vi "WVDIAL_3A_Data_v2.vi"() -> ()   [LabVIEW 2012]
uses:
  C:/H2O_DIAL/LabVIEW-2012/Newport_LabVIEW_v3-0-2/LabVIEW 2009/PowerMeterCommands.dll
  H2O_DIAL/LabVIEW-2012/Newport_LabVIEW_v3-0-2/LabVIEW 2009/PowerMeterCommands.dll
  <vilib>/DAQmx/write.llb/DAQmx Write (Digital 1D Bool NChan 1Samp 1Line).vi
  <vilib>/DAQmx/miscellaneous.llb/DAQmx Fill In Error Info.vi
  <vilib>/Analysis/baseanly.llb/Mean (DBL).vi
  H2O_DIAL/LabVIEW-2012/Scalar_Data.vi
  H2O_DIAL/LabVIEW-2012/Bristol WM V2_31b/CLDevIFace.dll
  <vilib>/Analysis/NI_AALBase.lvlib
panel:
  out "FileHour":i32=1
  out "L_Count":i32=91
  out "sigma_off_total":dbl[](array[numeric])=[5.2234200558950385e-25, 5.188441808210764e-25, 5.153565757684458e-25, 5.118792258898494e-25, 5.08412169128079e-25, 5.049554458516742e-25, 5.015090988058244e-25, 4.980731730520144e-25, 4.9464771591183625e-25, 4.912327769020908e-25, 4.878284076745431e-25, 4.844346619505553e-25, 4.810515954528075e-25, 4.776792658367297e-25, 4.743177326209202e-25, 4.709670571178148e-25, 4.676273023536675e-25, 4.642985329979768e-25, 4.60980815288796e-25, 4.576742169547043e-25, 4.543788071301696e-25, 4.510946562860497e-25, 4.478218361454665e-25, 4.445604195984992e-25, 4.413104806264462e-25, 4.380720942207995e-25, 4.348453362900999e-25, 4.316302835906913e-25, 4.284270136293901e-25, 4.252356045994737e-25, 4.220561352713886e-25, 4.188886849357295e-25, 4.157333332959233e-25, 4.125901604102425e-25, 4.0945924658480525e-25, 4.0634067231055894e-25, 4.0323451816809216e-25, 4.0014086475994155e-25, 3.970597926185606e-25, 3.9399138213596143e-25, 3.9093571347801357e-25, 3.878928665154662e-25, 3.848629207415147e-25, 3.8184595520156785e-25, 3.7884204841767665e-25, 3.7585127831272873e-25, 3.728737221470386e-25, 3.699094564429195e-25, 3.6695855692870667e-25, 3.6402109845120747e-25, 3.610971549313007e-25, 3.581867992981925e-25, 3.552901034160713e-25, 3.524071380427552e-25, 3.49537972759939e-25, 3.466826759230286e-25, 3.4384131460904257e-25, 3.4101395456540365e-25, 3.38200660154994e-25, 3.3540149432465886e-25, 3.326165185385074e-25, 3.298457927536896e-25, 3.270893753698064e-25, 3.2434732319867498e-25, 3.216196914181406e-25, 3.1890653354567716e-25, 3.1620790140097576e-25, 3.135238450817045e-25, 3.1085441293269563e-25, 3.081996515166733e-25, 3.0555960559996366e-25, 3.0293431812397327e-25, 3.0032383018574547e-25, 2.9772818102740086e-25, 2.951474080128153e-25, 2.925815466205591e-25, 2.9003063042754744e-25, 2.874946911049838e-25, 2.84973758409989e-25, 2.824678601768354e-25, 2.7997702231895546e-25, 2.775012688207971e-25, 2.7504062174242674e-25, 2.725951012245797e-25, 2.7016472548149107e-25, 2.677495108166955e-25, 2.6534947162834797e-25, 2.629646204115954e-25, 2.6059496777421353e-25, 2.5824052244655604e-25, 2.5590129129175218e-25, 2.535772793262254e-25, 2.5126848972851255e-25, 2.4897492386178596e-25, 2.4669658128642407e-25, 2.4443345978445496e-25, 2.4218555537559024e-25, 2.399528623422043e-25, 2.37735373247562e-25, 2.355330789669388e-25, 2.3334596869947745e-25, 2.311740300089403e-25, 2.2901724883551664e-25, 2.268756095284891e-25, 2.247490948773977e-25, 2.2263768613169987e-25, 2.205413630361226e-25, 2.184601038574965e-25, 2.163938854116898e-25, 2.1434268310139646e-25, 2.1230647093544735e-25, 2.1028522156937155e-25, 2.0827890633082375e-25, 2.0628749525435776e-25, 2.0431095710820085e-25, 2.0234925943095863e-25, 2.0040236856159133e-25, 1.9847024966907277e-25, 1.9655286678713153e-25, 1.946501828442999e-25, 1.9276215969536646e-25, 1.908887581541266e-25, 1.8902993802421601e-25, 1.8718565813176687e-25, 1.8535587635175008e-25, 1.8354054964632128e-25, 1.8173963408589502e-25, 1.7995308488869285e-25, 1.7818085644394773e-25, 1.7642290234549009e-25, 1.7467917541391984e-25, 1.729496277358023e-25, 1.7123421068169184e-25, 1.6953287493942957e-25, 1.6784557053870135e-25, 1.6617224687716046e-25, 1.645128527500769e-25, 1.6286733636906083e-25, 1.6123564539396905e-25, 1.5961772694937406e-25, 1.5801352765602062e-25, 1.5642299364526662e-25, 1.548460705871435e-25, 1.5328270370926741e-25, 1.51732837817522e-25, 1.5019641731424406e-25, 1.4867338622066092e-25, 1.4716368819285135e-25, 1.4566726653864935e-25, 1.44184064237116e-25, 1.42714023950682e-25, 1.412570880435065e-25, 1.3981319859339977e-25, 1.383822974081728e-25, 1.3696432603470826e-25, 1.3555922577345145e-25, 1.341669376883176e-25, 1.3278740261649085e-25, 1.3142056117906531e-25, 1.3006635378746162e-25, 1.2872472065372546e-25, 1.2739560179342136e-25, 1.2607893703627722e-25, 1.2477466602699388e-25, 1.234827282310524e-25, 1.222030629393837e-25, 1.2093560926749042e-25, 1.1968030615982307e-25, 1.1843709238949383e-25, 1.1720590655757887e-25, 1.1598668709159086e-25, 1.1477937224574596e-25, 1.1358390009609953e-25, 1.1240020853546206e-25, 1.1122823527270164e-25, 1.100679178237489e-25, 1.0891919350583027e-25, 1.077819994310042e-25, 1.0665627249682734e-25, 1.055419493776449e-25, 1.0443896651464614e-25, 1.0334726010358994e-25, 1.0226676608409127e-25, 1.0119742012573873e-25, 1.0013915761470858e-25, 9.909191363844297e-26, 9.805562297021883e-26, 9.703022005144416e-26, 9.60156389756751e-26, 9.501181346712233e-26, 9.401867686339235e-26, 9.303616209277055e-26, 9.206420165441348e-26, 9.110272759315423e-26, 9.015167147734415e-26, 8.921096437321057e-26, 8.828053681989907e-26, 8.73603188005984e-26, 8.645023971702555e-26, 8.555022835840961e-26, 8.466021287248513e-26, 8.378012073408909e-26, 8.290987871284668e-26, 8.204941284051091e-26, 8.119864837645385e-26, 8.035750977236182e-26, 7.952592063685049e-26, 7.870380369750861e-26, 7.78910807636565e-26, 7.708767268635035e-26, 7.629349932029705e-26, 7.550847948159768e-26, 7.47325309074078e-26, 7.396557021337458e-26, 7.320751285077931e-26, 7.245827306419816e-26, 7.171776384642328e-26, 7.098589689477262e-26, 7.026258256696376e-26, 6.954772983531929e-26, 6.884124624288349e-26, 6.814303785802483e-26, 6.745300923016202e-26, 6.677106334525768e-26, 6.609710158212605e-26, 6.543102366959471e-26, 6.477272764391407e-26, 6.412210980842389e-26, 6.34790646930539e-26, 6.284348501716449e-26, 6.221526165291305e-26, 6.159428359128027e-26, 6.098043791110177e-26, 6.037360974977726e-26, 5.977368227808834e-26, 5.918053667850245e-26, 5.859405212623739e-26, 5.801410577641224e-26, 5.744057275480635e-26, 5.687332615316891e-26, 5.631223703211629e-26, 5.575717442793144e-26, 5.520800536756566e-26, 5.466459488975701e-26, 5.412680607402506e-26, 5.35945000776066e-26, 5.306753618135332e-26, 5.254577184417943e-26, 5.202906276764818e-26, 5.1517262970050066e-26, 5.1010224871886087e-26, 5.050779939197868e-26, 5.000983605519522e-26, 4.9516183112447033e-26, 4.9026687672528495e-26, 4.854119584799368e-26, 4.8059552912484194e-26, 4.7581603473050947e-26, 4.710719165491264e-26, 4.663616130109859e-26, 4.616835618489491e-26, 4.570362023679514e-26, 4.524179778545254e-26, 4.478273381142984e-26, 4.432627421488372e-26, 4.3872266096240307e-26, 4.3420558048809627e-26, 4.297100046345158e-26, 4.252344584422084e-26, 4.2077749134265266e-26, 4.163376805034476e-26, 4.119136342586736e-26, 4.075039955995771e-26, 4.0310744572065636e-26, 3.987227076009789e-26, 3.943485496023477e-26, 3.8998378906971834e-26]
  out "sigma_on_total":dbl[](array[numeric])=[4.9081568957923354e-23, 4.92540132407037e-23, 4.9424189538428444e-23, 4.959204027078022e-23, 4.9757507806516237e-23, 4.992053449322544e-23, 5.008106268873085e-23, 5.0239034790046195e-23, 5.0394393268030595e-23, 5.054708069641985e-23, 5.0697039787676814e-23, 5.084421342075185e-23, 5.0988544683523154e-23, 5.1129976895868996e-23, 5.126845365311698e-23, 5.140391885773363e-23, 5.153631675468891e-23, 5.166559196475097e-23, 5.1791689527760933e-23, 5.1914554929330853e-23, 5.203413414598583e-23, 5.215037367456545e-23, 5.226322057682808e-23, 5.237262250900696e-23, 5.2478527766919827e-23, 5.2580885314179625e-23, 5.2679644828952156e-23, 5.277475673477536e-23, 5.2866172240694114e-23, 5.295384338012182e-23, 5.303772304537347e-23, 5.311776502184215e-23, 5.319392403512445e-23, 5.326615577767154e-23, 5.333441694809072e-23, 5.339866529189547e-23, 5.345885962979486e-23, 5.351495989921125e-23, 5.356692718784368e-23, 5.361472376181958e-23, 5.365831311243196e-23, 5.36976599768476e-23, 5.373273037898196e-23, 5.376349165681213e-23, 5.37899124988806e-23, 5.381196297008713e-23, 5.382961454332835e-23, 5.38428401304352e-23, 5.385161411059042e-23, 5.385591235070043e-23, 5.385571224246857e-23, 5.385099272271794e-23, 5.38417342942276e-23, 5.382791905459925e-23, 5.380953072059697e-23, 5.378655464011758e-23, 5.375897781966347e-23, 5.37267889433291e-23, 5.36899783827954e-23, 5.364853822719629e-23, 5.360246228475637e-23, 5.355174610231828e-23, 5.349638697779521e-23, 5.34363839732697e-23, 5.337173791660417e-23, 5.3302451421763e-23, 5.322852888345e-23, 5.314997649053672e-23, 5.306680222579485e-23, 5.29790158702747e-23, 5.28866290020075e-23, 5.278965499950113e-23, 5.268810903096198e-23, 5.2582008061107946e-23, 5.247137083724484e-23, 5.2356217884409377e-23, 5.2236571501233056e-23, 5.211245574333022e-23, 5.198389641603278e-23, 5.185092105901141e-23, 5.17135589337794e-23, 5.1571841000701964e-23, 5.142579991244177e-23, 5.127546998799546e-23, 5.112088718505753e-23, 5.096208909373192e-23, 5.0799114899221017e-23, 5.063200536129518e-23, 5.0460802792496746e-23, 5.028555101876762e-23, 5.0106295364265944e-23, 4.992308260936456e-23, 4.973596096602486e-23, 4.954498004029935e-23, 4.935019080307414e-23, 4.915164555028606e-23, 4.894939786914789e-23, 4.8743502601017755e-23, 4.8534015803309426e-23, 4.8320994710498925e-23, 4.8104497689477555e-23, 4.7884584208487056e-23, 4.766131478615105e-23, 4.7434750956610527e-23, 4.7204955219616444e-23, 4.69719910069179e-23, 4.6735922624026386e-23, 4.649681522533156e-23, 4.6254734750186114e-23, 4.600974789249439e-23, 4.57619220410126e-23, 4.5511325250906414e-23, 4.525802618610929e-23, 4.500209407611472e-23, 4.474359867273473e-23, 4.448261020445578e-23, 4.421919932603377e-23, 4.395343707548312e-23, 4.368539483365195e-23, 4.341514426954153e-23, 4.314275730762695e-23, 4.286830607379014e-23, 4.2591862848902865e-23, 4.2313500037219867e-23, 4.2033290113601744e-23, 4.1751305583264584e-23, 4.146761894203741e-23, 4.11823026276728e-23, 4.089542898843256e-23, 4.060707023565222e-23, 4.031729840885392e-23, 4.0026185329749454e-23, 3.9733802571128887e-23, 3.9440221417049496e-23, 3.914551282848814e-23, 3.8849747398167707e-23, 3.8552995327156094e-23, 3.8255326381372917e-23, 3.7956809869749994e-23, 3.7657514597924226e-23, 3.735750884129758e-23, 3.705686031888425e-23, 3.6755636163448055e-23, 3.64539028858424e-23, 3.6151726349373734e-23, 3.584917174725625e-23, 3.554630356985923e-23, 3.5243185586260696e-23, 3.4939880817830895e-23, 3.463645150634312e-23, 3.433295910921002e-23, 3.402946426295741e-23, 3.372602676523462e-23, 3.34227055661974e-23, 3.311955873523278e-23, 3.2816643454298113e-23, 3.25140159993815e-23, 3.221173171682913e-23, 3.1909845025572505e-23, 3.1608409383034083e-23, 3.1307477295284364e-23, 3.1007100281088115e-23, 3.070732888376049e-23, 3.04082126474433e-23, 3.0109800110649004e-23, 2.981213880845769e-23, 2.9515275248158936e-23, 2.921925492114598e-23, 2.8924122286396243e-23, 2.862992077239196e-23, 2.833669276844683e-23, 2.8044479630192115e-23, 2.7753321674532616e-23, 2.746325817565861e-23, 2.7174327372944447e-23, 2.688656646317821e-23, 2.6600011615395604e-23, 2.6314697957689884e-23, 2.6030659595305698e-23, 2.5747929606268752e-23, 2.5466540053635235e-23, 2.5186521982816548e-23, 2.4907905435188057e-23, 2.463071945366495e-23, 2.4354992087370023e-23, 2.4080750405260247e-23, 2.380802050198059e-23, 2.353682750766613e-23, 2.326719560301616e-23, 2.299914802049696e-23, 2.2732707065177826e-23, 2.2467894118572504e-23, 2.2204729660047475e-23, 2.1943233268536394e-23, 2.1683423643079143e-23, 2.1425318612924744e-23, 2.116893515101761e-23, 2.0914289389174596e-23, 2.0661396630556457e-23, 2.0410271362434758e-23, 2.016092727615468e-23, 1.991337727178575e-23, 1.9667633486579524e-23, 1.9423707291781575e-23, 1.9181609326455474e-23, 1.8941349497350253e-23, 1.8702937000488233e-23, 1.8466380333351368e-23, 1.8231687314796873e-23, 1.799886509336085e-23, 1.7767920163348423e-23, 1.753885838197544e-23, 1.7311684983845758e-23, 1.7086404592966803e-23, 1.686302123717775e-23, 1.6641538364768544e-23, 1.6421958857376648e-23, 1.620428504171699e-23, 1.598851870911703e-23, 1.5774661121324435e-23, 1.556271303190841e-23, 1.5352674693034418e-23, 1.5144545875226826e-23, 1.4938325872962545e-23, 1.473401352401079e-23, 1.4531607219009912e-23, 1.4331104915117057e-23, 1.4132504146459468e-23, 1.3935802040397153e-23, 1.374099532469008e-23, 1.3548080345265754e-23, 1.3357053070330198e-23, 1.3167909108681765e-23, 1.2980643720076896e-23, 1.2795251821945616e-23, 1.2611728005968538e-23, 1.2430066544509207e-23, 1.2250261405770924e-23, 1.2072306260846092e-23, 1.1896194495023627e-23, 1.1721919218843238e-23, 1.1549473277291007e-23, 1.1378849259678912e-23, 1.121003950934157e-23, 1.1043036133917084e-23, 1.0877831013862512e-23, 1.0714415811598837e-23, 1.0552781980469257e-23, 1.0392920773510609e-23, 1.023482325203656e-23, 1.0078480294731518e-23, 9.923882603736919e-24, 9.771020716164171e-24, 9.619885008426139e-24, 9.470465705295025e-24, 9.322752887996336e-24, 9.176736499509695e-24, 9.032406354244015e-24, 8.889752142972557e-24, 8.748763440184707e-24, 8.609429710000158e-24, 8.471740313713177e-24, 8.335684515307783e-24, 8.201251486848566e-24, 8.068430314303916e-24, 7.937210004283393e-24, 7.807579488329678e-24, 7.67952762979291e-24, 7.553043225158898e-24, 7.428115013769768e-24, 7.304731678841886e-24, 7.182881854618292e-24, 7.062554128232828e-24, 6.943737045965018e-24, 6.826419116313546e-24, 6.710588814858551e-24, 6.596234585700559e-24]
  out "background start":u32=269
  in  "Tab Control 2":enum32{"WV ND far", "WV ND near"}(tab)
  out "Water Vapor Number Density":dbl[][](graph)=[[-1.0252849343578538, 0.01224336928867699, 0.15835340670906267, 0.08290480575754477, 0.07669745638764922, 0.2620759623415424, 0.40352824259012626, 0.3765601485315456, 0.36227285880487015, 0.4059580103922654, 0.4019673046611201, 0.33405985865603577, 0.3170502464024163, 0.326931496733142, 0.3429736770934233, 0.3444364774253561, 0.2845356515320602, 0.21313783544633252, 0.23326342211099127, 0.28103729065715927, 0.21313141961111057, 0.18344699568861908, 0.1985633443430128, 0.15664306550500462, 0.14542928691246532, 0.1603391816642332, 0.16807578278873733, 0.15615183024203905, 0.07890698232192461, 0.05400641926340679, 0.10685143060938126, 0.08945067942871926, 0.0581898104690232, 0.029308456616610103, 0.03630780670213719, 0.10681104177716703, 0.100411545675493, 0.06706138343354981, 0.05685684243729449, 0.05193125527448508, 0.11348707030004936, 0.1035008699196596, 0.10995022367210285, 0.11937133833259062, 0.12610932475837994, 0.14237040514772434, 0.13877337413129362, 0.1368529199507475, 0.12016466926308586, 0.0995255538846496, 0.11327076262624056, 0.1147160375476178, 0.10327876531608772, 0.11333749442300015, 0.12152503880277782, 0.0905009235216747, 0.07461770257070978, 0.08412413953978554, 0.10800968932015705, 0.11174027116353434, 0.10857447444700312, 0.1321594882555679, 0.14442251058556227, 0.12312399237245467, 0.08690887689465081, 0.08885386048416666, 0.09841400838528362, 0.08885871503781699, 0.09065384006052782, 0.07631420811267337, 0.028801438306251165, 0.017317933019278177, 0.00535924647765615, -0.009366925462381862, 0.02537030105111806, 0.04553727504960618, 0.04087573332295979, 0.009566848406822514, -0.03765211983627373, -0.030845499715426574, 0.0094243698383032, -0.01191307862878305, -0.007766189150850719, 0.02512004862547047, -0.009588975820370573, -0.021862900628392096, -0.02332999129653946, -0.008298987729287529, 0.03829137791338236, 0.06788185167298495, 0.04415872088882591, 0.04626176957978276, 0.05722361632703139, -0.022937610835842275, -0.004658082206540099, 0.03497441915011394, 0.014559704329153577, 0.018331797591107316, 0.0002765651829681014, -0.01750292048905302, -0.01389136569261041, -0.0148966495460508, 0.03341365244368827, 0.07959799083893267, 0.001172873742239602, -0.04989443850404001, 0.019178610287384813, 0.022978059399375285, -0.021897118324035424, 0.014353504774367415, 0.05207825830382806, 0.02543732315528786, -0.08859996249031706, -0.07930855892996377, 0.02199957803258167, -0.005751854282845175, -0.06734218818626583, -0.06101837900811169, 0.00811186048587734, -0.030347870972451, -0.018601423955109716, 0.025343088130804294, -0.000654365715296774, -0.021410549313652594, -0.00711404508875446, 0.015640507400628483, 0.01980450921423653, -0.020816862317439747, -0.13136076782915793, -0.04953574617480027, -0.015688088030325335, 0.012270851704896515, 0.07078369570658659, -0.010036414876574785, -0.07560094992065346, 0.029113962431097925, 0.022316828296317252, 0.01590620564861339, 0.115062446638934, -0.02408844575634284, -0.17020265488657252, -0.1451398382852584, -0.02445566701513559, -0.03235393341027663, 0.02164604133106217, 0.03204665984442202, -0.027642125840527564, 0.0006023003531748955, 0.0003496841625749631, 0.020854103047599864, 0.10842911005120683, -0.03471048223400414, -0.24585708970897793, -0.05744168418466623, 0.10508588586604846, -0.0012595297900689863, -0.1422957818224093, -0.1528480963241691, -0.024891406845158556, 0.18064750429676343, 0.18870158459369052, 0.08124391772376854, 0.1925945351989546, 0.18885896239951047, -0.028423489511011396, 0.08782982844147444, 0.4018531072514305, 0.28295974281274405, 0.141752362604584, -0.04596416681267469, -0.19599669013524573, -0.1832886215602881, -0.221330016936266, -0.20746810479592004, -0.2533548550992385, -0.2640461399425933, -0.5552226085781474, -0.25658834207217607, 0.07631635532473394, 0.24357172305557667, 0.24357507864442013, 0.0054930164331440596, -0.26352244101342837, -0.21458731889229515, 0.4671152360442577, 0.35493908142470326, 0.540206234420223, 0.6253545626789414, -0.1918135463763898, -0.857997351327124, -0.6115474584870345, 0.12686579467009856, 1.1193396529920683, 0.9491303824250846, -0.24898239698578367, -0.2173961551411876, -0.4716937237467244, -0.9264813435003413, -0.0023983309321438844, 0.13861484422091855, 0.18306415863530784, 0.05031596208368666, -0.9039913856241271, -0.8292733524419981, -0.5087347525929017, -0.6153644321851048, -0.14914507407421404, -0.42810566981401466, -1.247232243863552, 0.05482762929954191, 0.6860297651363804, 0.9481996959641221, 0.5629045863681271, -0.04576191379675542, -0.08731851988840891, 0.15154855903866532, 0.9587585142774312, 2.6746560753275936, 2.531440286016611, 1.3601958991015755, 1.2395200095649133, -0.6781596022648028, -1.1160153572546019, 0.5812137856885836, 3.4687378449956365, 1.4464917210606263, -0.9295342166169639, -1.1204191549870324, 0.1034792544561276, -0.3306455660619927, -1.6655638739808207, -0.17082350185743553, 1.078813649527156, 1.0096264846682745, 5.118342980436561, -0.5598249934362547, -3.0525737805264908, -2.493481796852318, -0.6766514276077036, -1.9364332962989481, -0.9603886125585042, 9.722825473022084, 12.019451658920579, 1.5485181169999382, -10.639197997428594, 1.410760631694313, 1.6311961050885482, -0.7606371982561374, 8.050945482359824, 12.222718623912504, 2.8379417404869214, -8.467893225176228, -7.892104308000269, 7.561105736814597, 1.8338678599324048, -24.44144266759318, -5.501789806042863, inf, nan, nan, nan, nan, nan, nan, nan, nan, nan, -inf, -28.22132689188821, -35.53185818775793, -6.267550590333384, -0.5649805048183769, 4.752482348133581, -307.43485402739964, 20.288829520425445, 9.757029206652764, 0.0, 0.0, 0.0, 0.0]]
  out "Water Vapor Number Density 2":dbl[][](graph)=[[-0.2865898034035239, 0.005398347357826392, 0.270180194427171, 0.49934908193536914, 0.4610856820815434, 0.47919125201054663, 0.41713553122041214, 0.2839520922325461, 0.2139053579349078, 0.19008321561295816, 0.16210313849803437, 0.19767316841001897, 0.24678082445960892, 0.22934149302256987, 0.23106320058472932, 0.24935743336579463, 0.228712861153675, 0.19177244383258807, 0.13822796107116675, 0.12952096392054793, 0.184961155888618, 0.15625046859598593, 0.08149130905587414, 0.08347671564892852, 0.09292450724175014, 0.09897778476272892, 0.11869505217402627, 0.1020949650068219, 0.0680375451406521, 0.05526436285002661, 0.07701578642588422, 0.08986190584998056, 0.04739696394569468, 0.05155875974538851, 0.1075732163983899, 0.05848975405725049, 0.06027341501459341, 0.15577956438219154, 0.15426807453320523, 0.119550419057958, 0.09023852284476494, 0.10731660449440052, 0.10201202655632406, 0.09015213641438144, 0.10411287521775274, 0.10329612538676994, 0.09329592009020822, 0.094255010754596, 0.11657739187690068, 0.1226902118059504, 0.09973483618224008, 0.10146470794396166, 0.11296540573869736, 0.1015626599598415, 0.0670589224001955, 0.05571375145680353, 0.11089663210326146, 0.11357746332799534, 0.06533120875001214, 0.06501193077064142, 0.07135694632306648, 0.08396571641123735, 0.10053779135695375, 0.10873851949177482, 0.1112833067067629, 0.1253430050297553, 0.0751893159577234, 0.03758941994591285, 0.07455579053102862, 0.0833519595042809, 0.08073822675968761, 0.07046574397017079, 0.01628475622108129, -0.00979323785755199, -0.0064363595850521265, -0.05424049805498369, -0.04770145348367631, -0.0651157050563226, -0.05842221368779357, -0.010132741906781893, -0.04719311826522132, -0.08061528212640966, -0.05584093426722229, -0.03736190901125273, -0.026288927003514956, -0.02735758962233305, -0.016680414061933085, 0.08698302754384295, 0.03703409407182322, -0.07428276239552731, -0.08287843499135167, -0.07246514962772428, -0.037888971379870164, 0.05050165939688743, 0.04070516703725998, 0.0013689744815177922, -0.004086178413386218, -0.0567087326925041, -0.02261065358974721, 0.013323062997568018, 0.009012099767637038, 0.06812410181727888, 0.0873623313874923, -0.04033859274693685, -0.04056170573479139, 0.018164119949206622, 0.01698920493116969, 0.03200462135731041, 0.05597485931968883, 0.004660639245897041, -0.03363415325850763, -0.044356505658716565, -0.1326763990388899, -0.1163166059591595, -0.10490018463375138, -0.05536956764781129, -0.04811219794033331, -0.14629275993812393, -0.2638330330801213, -0.11815301138792501, -0.05480137234021616, -0.09557382991076353, 0.05065173829933405, -0.021513840363060137, -0.06814917790551435, 0.04024699076309072, 0.0523783228597919, 0.024958814896366536, 0.2367237292842569, 0.15812901488128575, 0.1896038115178739, 0.17481292374171756, 0.0304620500948119, 0.17383097270155906, -0.0259345430012192, -0.08930431039819542, -0.03743898194871775, -0.11917226232517714, -0.33721378185498047, -0.457167967758754, -0.3235026283764478, -0.10013715416333623, -0.02199546241885382, -0.14544493363592895, -0.0012521147959781197, -0.12646742039302086, -0.09850072568755051, 0.0784720451940167, 0.023479703348949714, 0.1557391494055616, 0.0758192113998383, -0.07227019057095403, -0.1648907418364726, -0.2554862575973906, -0.19723726926026697, -0.23979967592154308, -0.3956428807050192, -0.15151433375207188, 0.05856942593990406, 0.023473089930657325, -0.14087719685328506, -0.4039827327250235, -0.5481665412712616, -0.038628654542470754, 0.06243643308227342, -0.11889452169279512, 0.16177519315495192, -0.12021089755834058, -0.3297469880649382, -0.518217006463964, -0.6546943085223443, -0.40952325606659373, 0.011280533075510508, 0.03250743328819382, -0.10886758905219632, -0.021942577298229692, -0.4883511099304952, -0.44815383519345425, -0.03907380619628987, 0.023132386308057345, 0.8029360270671851, 1.1829320153858496, 0.40773978168304786, -0.38586510407162455, -0.17087296696587043, 0.24229231771964327, 0.7259049980139611, 1.087664173140548, 0.33172479606023236, 0.17410391403140907, -0.4906222320735112, -0.8636149031554697, -0.714888070381581, -0.5064304478291466, -0.15804241196057325, -0.708135007951393, -1.0726075380347868, -1.5391461936251392, -0.22970891454111933, 0.36396836324290655, -0.04868841888359483, 0.05730398934642209, 0.29784952872844606, 0.6519924801558464, 0.4451080921193637, 0.12546276730951203, 0.2049887743797555, 0.5372091833320591, -0.9537044878290641, -1.2245695847958014, -0.41139863470143095, -1.7400865412460473, -1.1839668465437496, 0.13325930619296222, 0.43022454257193565, 1.251772185641275, 0.3265410906776107, -0.2873287006786283, -0.6181403368800276, 0.2720806718243457, 0.8886029089360986, 1.1163369370933798, -0.47349237339872063, -2.3967729698196005, -2.207549933190577, -1.4281793307099488, -2.552445952127832, -3.068147980767434, 1.6399347380926848, 1.9114132952232707, 2.6314283459178442, 3.2209701873261984, 4.083938620485938, 1.6750231442344234, 0.7521082601842183, 0.6308908979632994, -1.7929692303061833, 0.4854925493859792, -1.848037270233985, -1.9599707690472083, 0.22935120759831343, -3.8719930860396916, -5.299588916827538, -1.5732432106802883, -2.5938334904711406, -4.391792042628007, 4.266433069695473, 13.43473735963336, 5.908032793145804, 1.2717711422320495, -3.429469533815916, -1.1590160228244126, -0.6038000728103482, -12.455047324042539, -5.212730955931867, -6.095310308846368, -9.413121255666667, -16.629619714029694, -4.639137025788683, -7.453414942524888, -8.645137330486625, -6.187073306219781, -3.0975960529606095, 31.089273555509546, 10.980893562167019, 19.41155124836945, 9.628163529298224, 13.46382743910762, -10.97019753650602, -9.201787138642892, -10.247187579852502, -10.523303442697749, -12.419610661601844, -35.596073167566956, -21.555444628010434, -28.144694005095776, 0.0, 0.0, 0.0, 0.0]] caption="Water Vapor Number Density"
  out "RingBuffer offline near":dbl[][](array[numeric])
  out "RingBuffer aerosol near":dbl[][](array[numeric])=[[17571.5, 17868.5, 12324.5, 82.5, 83.5, 164.5, 248.5, 292.5, 320.5, 359.5, 383.5, 402.5, 395.5, 359.5, 311.5, 314.5, 336.5, 344.5, 270.5, 256.5, 274.5, 222.5, 209.5, 199.5, 193.5, 161.5, 148.5, 149.5, 165.5, 133.5, 119.5, 104.5, 109.5, 100.5, 83.5, 89.5, 69.5, 67.5, 57.5, 61.5, 58.5, 72.5, 54.5, 63.5, 66.5, 59.5, 46.5, 39.5, 47.5, 38.5, 34.5, 33.5, 44.5, 28.5, 34.5, 23.5, 21.5, 26.5, 37.5, 16.5, 22.5, 15.5, 18.5, 14.5, 18.5, 16.5, 22.5, 10.5, 21.5, 17.5, 19.5, 21.5, 12.5, 14.5, 17.5, 18.5, 20.5, 16.5, 11.5, 12.5, 12.5, 16.5, 6.5, 9.5, 0.5, 14.5, 7.5, 8.5, 5.5, 7.5, 8.5, 8.5, 5.5, 8.5, 5.5, 5.5, 6.5, 8.5, 4.5, 2.5, 6.5, 3.5, 5.5, 2.5, 7.5, 10.5, 7.5, 3.5, 8.5, 3.5, 10.5, 10.5, 5.5, 3.5, 2.5, 5.5, 4.5, 9.5, 6.5, 3.5, 4.5, -0.5, 4.5, 1.5, 2.5, 3.5, 1.5, 6.5, -0.5, -0.5, -1.5, -0.5, 5.5, 5.5, 2.5, 0.5, -0.5, 2.5, -0.5, 0.5, -0.5, 0.5, 5.5, 0.5, 1.5, -0.5, 3.5, 1.5, 3.5, 3.5, 3.5, -1.5, 0.5, 1.5, 0.5, 0.5, 0.5, 0.5, -0.5, -0.5, 4.5, -0.5, 1.5, -1.5, 2.5, -0.5, -0.5, 4.5, -0.5, 0.5, 1.5, -0.5, -0.5, 4.5, 0.5, -0.5, -0.5, 0.5, -0.5, 1.5, -0.5, 0.5, -0.5, 0.5, -0.5, -0.5, -0.5, -1.5, -0.5, 1.5, 1.5, -1.5, -1.5, 0.5, 0.5, -1.5, 0.5, -1.5, 0.5, -0.5, 3.5, 1.5, 1.5, -1.5, -0.5, -0.5, 1.5, -0.5, -0.5, -0.5, -1.5, 0.5, -1.5, 0.5, 3.5, -0.5, -0.5, -0.5, 0.5, 0.5, -1.5, -0.5, -1.5, 0.5, -1.5, 1.5, 0.5, 0.5, -0.5, 3.5, -0.5, 1.5, 0.5, -1.5, -0.5, 0.5, -0.5, -0.5, -1.5, -0.5, -1.5, -0.5, 0.5, -1.5, -1.5, -1.5, 0.5, -0.5, -1.5, -1.5, 0.5, 0.5, -1.5, -0.5, 0.5, 0.5, 0.5, 0.5, -0.5, 0.5, -1.5, -1.5, -1.5, 0.5, -0.5, -0.5, 1.5, -1.5, 0.5, -1.5, -0.5, -0.5, -0.5, 0.5, -0.5, 0.5, 1.5, 0.5, 0.5], [18920.5, 19235.5, 12427.5, 85.5, 107.5, 173.5, 275.5, 258.5, 313.5, 342.5, 323.5, 399.5, 353.5, 364.5, 366.5, 322.5, 323.5, 295.5, 273.5, 289.5, 284.5, 247.5, 210.5, 195.5, 218.5, 157.5, 162.5, 151.5, 134.5, 117.5, 113.5, 101.5, 110.5, 98.5, 88.5, 87.5, 78.5, 75.5, 60.5, 47.5, 60.5, 44.5, 61.5, 54.5, 47.5, 60.5, 62.5, 41.5, 30.5, 48.5, 52.5, 37.5, 36.5, 24.5, 24.5, 26.5, 29.5, 35.5, 28.5, 19.5, 23.5, 23.5, 16.5, 25.5, 20.5, 19.5, 13.5, 13.5, 18.5, 19.5, 24.5, 18.5, 20.5, 21.5, 21.5, 26.5, 21.5, 11.5, 16.5, 11.5, 4.5, 13.5, 9.5, 6.5, 9.5, 8.5, 12.5, 10.5, 12.5, 7.5, 10.5, 10.5, 4.5, 8.5, 10.5, 1.5, 7.5, 3.5, 9.5, 8.5, 6.5, 4.5, 6.5, 3.5, 12.5, 6.5, 9.5, 1.5, 8.5, 8.5, 9.5, 11.5, -0.5, 2.5, 4.5, 3.5, -1.5, 4.5, 5.5, 7.5, 4.5, 3.5, 5.5, 1.5, 3.5, 3.5, 3.5, 2.5, 5.5, 4.5, 2.5, 3.5, -0.5, 8.5, 3.5, 0.5, 0.5, 3.5, 0.5, -0.5, 3.5, 0.5, 2.5, 1.5, 0.5, 2.5, 2.5, 4.5, 2.5, 2.5, 2.5, 0.5, 2.5, 3.5, 1.5, 0.5, 2.5, -0.5, 1.5, 1.5, 1.5, 2.5, 1.5, 3.5, 2.5, 2.5, 2.5, -1.5, -0.5, -0.5, -1.5, 0.5, -0.5, 3.5, 2.5, 1.5, 1.5, 1.5, 2.5, -0.5, -1.5, -1.5, -1.5, -0.5, 0.5, -1.5, -1.5, 0.5, -0.5, 0.5, -0.5, -1.5, 2.5, 1.5, 1.5, 0.5, 0.5, -0.5, 0.5, -1.5, -0.5, -0.5, 1.5, -0.5, -1.5, -1.5, 1.5, -1.5, 2.5, 0.5, 0.5, -0.5, 2.5, -1.5, -0.5, 0.5, -1.5, -0.5, -1.5, 1.5, 0.5, -0.5, -1.5, 2.5, -1.5, -0.5, 0.5, -0.5, -0.5, -0.5, 1.5, -0.5, -1.5, -1.5, -1.5, -1.5, 2.5, -1.5, -0.5, -1.5, -1.5, -1.5, -0.5, -0.5, 0.5, 0.5, -1.5, 2.5, 0.5, -0.5, 0.5, -1.5, -1.5, 1.5, -0.5, -0.5, -0.5, 2.5, 0.5, -0.5, -1.5, -1.5, 1.5, -0.5, 0.5, 0.5, -0.5, -0.5, -0.5, 0.5, -0.5, 0.5, -1.5, -0.5, 0.5, -0.5, -0.5, 2.5, -0.5], [18593.2, 18818.2, 12421.2, 94.2, 101.2, 173.2, 229.2, 257.2, 290.2, 347.2, 331.2, 348.2, 331.2, 330.2, 316.2, 327.2, 321.2, 310.2, 272.2, 279.2, 230.2, 216.2, 216.2, 158.2, 152.2, 184.2, 151.2, 139.2, 144.2, 124.2, 98.2, 113.2, 80.2, 87.2, 67.2, 85.2, 78.2, 68.2, 75.2, 67.2, 53.2, 82.2, 36.2, 50.2, 49.2, 34.2, 46.2, 51.2, 32.2, 39.2, 45.2, 46.2, 38.2, 28.2, 18.2, 31.2, 20.2, 21.2, 24.2, 22.2, 14.2, 28.2, 26.2, 14.2, 13.2, 18.2, 15.2, 20.2, 15.2, 14.2, 19.2, 14.2, 21.2, 13.2, 18.2, 12.2, 11.2, 18.2, 9.2, 13.2, 10.2, 10.2, 11.2, 11.2, 8.2, 8.2, 17.2, 13.2, 8.2, 3.2, 1.2, 7.2, 7.2, 6.2, 5.2, 10.2, 3.2, 6.2, 4.2, 6.2, 1.2, 2.2, 6.2, 2.2, 2.2, 5.2, 9.2, 3.2, 8.2, 6.2, 9.2, 4.2, 3.2, 1.2, 3.2, 8.2, 4.2, 2.2, 4.2, 3.2, 3.2, 1.2, 3.2, 2.2, 8.2, 1.2, 4.2, 3.2, -0.8, 3.2, 3.2, 6.2, 1.2, 2.2, -0.8, 1.2, 3.2, 2.2, 1.2, -0.8, 5.2, 2.2, 2.2, 0.19999999999999996, -1.8, -0.8, 2.2, 1.2, 2.2, 3.2, 1.2, 2.2, 2.2, 2.2, 1.2, 0.19999999999999996, 4.2, 0.19999999999999996, 0.19999999999999996, 1.2, 1.2, 0.19999999999999996, 1.2, 1.2, 0.19999999999999996, 3.2, -1.8, 0.19999999999999996, 0.19999999999999996, -0.8, 0.19999999999999996, -1.8, -0.8, 2.2, 0.19999999999999996, 0.19999999999999996, 0.19999999999999996, 0.19999999999999996, -0.8, 4.2, -0.8, 0.19999999999999996, -0.8, 1.2, 2.2, -1.8, -0.8, -0.8, 0.19999999999999996, 1.2, -0.8, 1.2, 2.2, -0.8, -1.8, 1.2, -0.8, 0.19999999999999996, 0.19999999999999996, -1.8, 0.19999999999999996, 0.19999999999999996, 0.19999999999999996, 1.2, -0.8, 1.2, 0.19999999999999996, 0.19999999999999996, 2.2, -1.8, 0.19999999999999996, -1.8, 0.19999999999999996, -1.8, -0.8, 0.19999999999999996, 1.2, -0.8, 1.2, 0.19999999999999996, 1.2, 0.19999999999999996, 1.2, -1.8, -1.8, -0.8, -0.8, 1.2, 1.2, 0.19999999999999996, -1.8, -0.8, -1.8, -0.8, -0.8, -1.8, 1.2, 1.2, 0.19999999999999996, -1.8, -0.8, -0.8, 0.19999999999999996, -1.8, -0.8, -0.8, -0.8, -1.8, -0.8, -0.8, -0.8, 0.19999999999999996, 0.19999999999999996, -0.8, 3.2, -0.8, -0.8, -1.8, 0.19999999999999996, -1.8, -1.8, -0.8, -0.8, -0.8, -0.8, 0.19999999999999996, 1.2, -1.8, -1.8, 0.19999999999999996, 2.2, 1.2, -1.8, 0.19999999999999996, 0.19999999999999996, -1.8, 0.19999999999999996, 0.19999999999999996, -0.8], [17590.3, 17550.3, 14081.3, 143.3, 259.3, 405.3, 599.3, 814.3, 813.3, 814.3, 799.3, 805.3, 855.3, 762.3, 747.3, 683.3, 617.3, 521.3, 525.3, 458.3, 410.3, 371.3, 318.3, 270.3, 239.3, 238.3, 243.3, 221.3, 194.3, 177.3, 178.3, 133.3, 132.3, 128.3, 84.3, 119.3, 97.3, 96.3, 88.3, 91.3, 71.3, 87.3, 70.3, 60.3, 74.3, 44.3, 57.3, 42.3, 68.3, 43.3, 43.3, 54.3, 53.3, 47.3, 36.3, 30.3, 41.3, 36.3, 45.3, 26.3, 29.3, 28.3, 19.3, 20.3, 32.3, 30.3, 31.3, 21.3, 22.3, 25.3, 33.3, 27.3, 19.3, 30.3, 26.3, 31.3, 31.3, 23.3, 34.3, 32.3, 23.3, 22.3, 23.3, 11.3, 22.3, 5.3, 8.3, 8.3, 7.3, 13.3, 4.3, 8.3, 12.3, 14.3, 4.3, 11.3, 9.3, 5.3, 12.3, 8.3, 8.3, 6.3, 9.3, 11.3, 1.3, 6.3, 7.3, 3.3, 3.3, 3.3, 5.3, 7.3, 4.3, 7.3, 2.3, 0.30000000000000004, 2.3, 4.3, 11.3, 4.3, 6.3, 3.3, 6.3, 2.3, 5.3, 5.3, 2.3, 2.3, 10.3, 1.3, 6.3, 3.3, 4.3, 7.3, 2.3, 2.3, 4.3, 3.3, 3.3, 3.3, 2.3, -0.7, 4.3, 1.3, 1.3, 0.30000000000000004, 4.3, -1.7, 2.3, 2.3, -0.7, -0.7, 1.3, 2.3, 0.30000000000000004, 1.3, 1.3, 4.3, 0.30000000000000004, 0.30000000000000004, 1.3, 4.3, 0.30000000000000004, 2.3, 1.3, 2.3, 0.30000000000000004, 3.3, 0.30000000000000004, -0.7, 0.30000000000000004, 2.3, 0.30000000000000004, 2.3, -0.7, 1.3, 0.30000000000000004, 0.30000000000000004, 4.3, 1.3, 1.3, -0.7, 2.3, 3.3, -0.7, -1.7, 0.30000000000000004, 1.3, 1.3, -0.7, 0.30000000000000004, 0.30000000000000004, 3.3, 1.3, 2.3, 0.30000000000000004, 1.3, 2.3, -0.7, -0.7, 0.30000000000000004, 0.30000000000000004, 2.3, 1.3, 2.3, 0.30000000000000004, 1.3, -0.7, 1.3, -0.7, -0.7, 0.30000000000000004, -1.7, -0.7, -0.7, 0.30000000000000004, 1.3, 2.3, -1.7, 2.3, -0.7, 1.3, -0.7, 3.3, 2.3, 1.3, 0.30000000000000004, -0.7, 2.3, 0.30000000000000004, 2.3, -0.7, -1.7, 1.3, -1.7, -1.7, -0.7, 0.30000000000000004, -0.7, 1.3, 2.3, 1.3, 0.30000000000000004, 2.3, 0.30000000000000004, -0.7, -1.7, 3.3, 2.3, -0.7, -0.7, 2.3, 3.3, 1.3, -0.7, -1.7, -1.7, 1.3, 1.3, 0.30000000000000004, -0.7, -1.7, -1.7, 0.30000000000000004, 2.3, -1.7, -0.7, 4.3, 0.30000000000000004, 0.30000000000000004, 0.30000000000000004, 0.30000000000000004, -0.7, -0.7, -0.7, 0.30000000000000004, 2.3, -1.7, 0.30000000000000004], [18528.9, 18571.9, 14214.9, 143.9, 231.9, 461.9, 613.9, 737.9, 830.9, 845.9, 835.9, 898.9, 891.9, 780.9, 732.9, 651.9, 604.9, 546.9, 495.9, 448.9, 415.9, 348.9, 315.9, 273.9, 291.9, 245.9, 228.9, 195.9, 196.9, 195.9, 165.9, 142.9, 135.9, 130.9, 127.9, 112.9, 108.9, 106.9, 103.9, 81.9, 66.9, 70.9, 77.9, 62.9, 69.9, 84.9, 56.9, 53.9, 47.9, 58.9, 51.9, 47.9, 47.9, 43.9, 31.9, 40.9, 43.9, 33.9, 42.9, 37.9, 27.9, 28.9, 34.9, 24.9, 20.9, 25.9, 23.9, 25.9, 32.9, 46.9, 44.9, 24.9, 36.9, 37.9, 43.9, 36.9, 31.9, 33.9, 34.9, 26.9, 33.9, 29.9, 24.9, 8.9, 15.9, 15.9, 13.9, 11.9, 8.9, 4.9, 5.9, 10.9, 4.9, 14.9, 7.9, 8.9, 8.9, 7.9, 14.9, 8.9, 11.9, 4.9, 6.9, 3.9, 3.9, 3.9, 5.9, 2.9, 6.9, 3.9, 4.9, 5.9, 8.9, 5.9, 8.9, 6.9, 4.9, 8.9, 2.9, 3.9, 3.9, 8.9, 2.9, 1.9, 0.8999999999999999, 2.9, 1.9, 7.9, 3.9, 8.9, 5.9, 4.9, 1.9, 4.9, 6.9, 2.9, 1.9, 3.9, 1.9, -0.10000000000000009, 1.9, 3.9, 3.9, 2.9, 2.9, 3.9, -1.1, 0.8999999999999999, 0.8999999999999999, 2.9, 3.9, 4.9, 5.9, 2.9, 3.9, 1.9, 2.9, 2.9, 2.9, 2.9, -0.10000000000000009, 6.9, 4.9, 2.9, -1.1, 2.9, 0.8999999999999999, 3.9, 0.8999999999999999, 2.9, 4.9, -0.10000000000000009, 0.8999999999999999, 2.9, 0.8999999999999999, 3.9, 1.9, 0.8999999999999999, -0.10000000000000009, 0.8999999999999999, 0.8999999999999999, -0.10000000000000009, 7.9, -0.10000000000000009, 5.9, 1.9, 3.9, 3.9, 2.9, 1.9, 0.8999999999999999, 0.8999999999999999, 0.8999999999999999, 0.8999999999999999, 3.9, 2.9, 1.9, 2.9, -1.1, 0.8999999999999999, -0.10000000000000009, 0.8999999999999999, 3.9, 5.9, -0.10000000000000009, 1.9, 0.8999999999999999, 0.8999999999999999, 3.9, -0.10000000000000009, 0.8999999999999999, 1.9, 2.9, 0.8999999999999999, 0.8999999999999999, 2.9, 2.9, 0.8999999999999999, 2.9, 0.8999999999999999, 2.9, 0.8999999999999999, -0.10000000000000009, 2.9, -0.10000000000000009, 0.8999999999999999, -0.10000000000000009, 0.8999999999999999, -1.1, -0.10000000000000009, -0.10000000000000009, 0.8999999999999999, 0.8999999999999999, -0.10000000000000009, -0.10000000000000009, 4.9, 2.9, -1.1, 1.9, -0.10000000000000009, 0.8999999999999999, 0.8999999999999999, 0.8999999999999999, -0.10000000000000009, 2.9, 0.8999999999999999, -0.10000000000000009, 2.9, -0.10000000000000009, -0.10000000000000009, 4.9, 1.9, -1.1, 1.9, 0.8999999999999999, 0.8999999999999999, 1.9, 0.8999999999999999, -0.10000000000000009, -0.10000000000000009, -0.10000000000000009, -0.10000000000000009, -0.10000000000000009, 0.8999999999999999, 0.8999999999999999, -1.1, -1.1, 1.9, 0.8999999999999999, -0.10000000000000009, -0.10000000000000009, -1.1, 0.8999999999999999, -1.1, 2.9, -0.10000000000000009, -1.1, -0.10000000000000009, -0.10000000000000009], [18991.7, 18829.7, 14030.7, 140.7, 236.7, 363.7, 432.7, 605.7, 702.7, 785.7, 796.7, 842.7, 723.7, 703.7, 710.7, 679.7, 614.7, 578.7, 569.7, 506.7, 417.7, 380.7, 358.7, 331.7, 292.7, 266.7, 264.7, 216.7, 198.7, 217.7, 189.7, 174.7, 149.7, 139.7, 132.7, 118.7, 126.7, 94.7, 81.7, 91.7, 89.7, 75.7, 65.7, 75.7, 60.7, 68.7, 56.7, 60.7, 61.7, 51.7, 53.7, 55.7, 59.7, 56.7, 50.7, 36.7, 32.7, 33.7, 34.7, 26.7, 17.7, 35.7, 31.7, 14.7, 24.7, 23.7, 16.7, 26.7, 33.7, 37.7, 27.7, 24.7, 34.7, 34.7, 40.7, 31.7, 30.7, 48.7, 30.7, 31.7, 16.7, 19.7, 22.7, 17.7, 12.7, 5.7, 7.7, 16.7, 14.7, 14.7, 11.7, 7.7, 7.7, 16.7, 10.7, 13.7, 5.7, 11.7, 3.7, 12.7, 5.7, 7.7, 7.7, 6.7, 3.7, 4.7, 10.7, 6.7, 6.7, 8.7, 7.7, 1.7, 8.7, 6.7, 8.7, 4.7, 8.7, 2.7, 7.7, 6.7, 4.7, 5.7, 5.7, 0.7, 3.7, 4.7, 0.7, 4.7, 0.7, 0.7, 2.7, 3.7, 8.7, 3.7, 1.7, 2.7, 6.7, 3.7, 3.7, 3.7, 0.7, 4.7, 2.7, 5.7, 3.7, -0.30000000000000004, 0.7, 0.7, 4.7, 1.7, 4.7, -0.30000000000000004, 1.7, 1.7, 2.7, 1.7, 2.7, 3.7, -0.30000000000000004, 3.7, 5.7, 0.7, 1.7, 3.7, 1.7, 0.7, 2.7, 3.7, 1.7, 0.7, -1.3, 1.7, 0.7, 0.7, 1.7, 1.7, 2.7, 4.7, 1.7, -0.30000000000000004, 0.7, -1.3, 1.7, 2.7, -0.30000000000000004, -0.30000000000000004, -0.30000000000000004, 4.7, 1.7, 1.7, -0.30000000000000004, 1.7, 2.7, 2.7, -0.30000000000000004, 1.7, -0.30000000000000004, 2.7, -0.30000000000000004, 0.7, -1.3, -0.30000000000000004, 2.7, -0.30000000000000004, 1.7, 0.7, 0.7, 0.7, 1.7, -1.3, 0.7, 2.7, 3.7, -0.30000000000000004, 0.7, -0.30000000000000004, -0.30000000000000004, 0.7, 2.7, 1.7, 0.7, 2.7, 0.7, -1.3, 2.7, 0.7, 2.7, -0.30000000000000004, 0.7, -0.30000000000000004, 3.7, 0.7, 0.7, 0.7, -1.3, -0.30000000000000004, 1.7, 0.7, -1.3, -0.30000000000000004, -0.30000000000000004, 1.7, 0.7, -0.30000000000000004, 1.7, 1.7, 1.7, -0.30000000000000004, 1.7, 0.7, -0.30000000000000004, 0.7, 1.7, 0.7, -1.3, 0.7, 2.7, -0.30000000000000004, 1.7, 0.7, 0.7, -0.30000000000000004, -0.30000000000000004, -0.30000000000000004, 0.7, 0.7, 0.7, -0.30000000000000004, 3.7, 0.7, 0.7, -0.30000000000000004, 0.7, -1.3, 0.7, -1.3, -0.30000000000000004, -1.3, 1.7], [18330.6, 18215.6, 13817.6, 117.6, 230.6, 328.6, 427.6, 580.6, 738.6, 764.6, 774.6, 740.6, 765.6, 753.6, 683.6, 637.6, 584.6, 556.6, 554.6, 484.6, 458.6, 361.6, 311.6, 294.6, 274.6, 279.6, 226.6, 211.6, 190.6, 176.6, 180.6, 166.6, 154.6, 133.6, 124.6, 136.6, 79.6, 85.6, 88.6, 86.6, 87.6, 75.6, 80.6, 75.6, 57.6, 57.6, 49.6, 56.6, 46.6, 37.6, 53.6, 46.6, 46.6, 55.6, 55.6, 43.6, 44.6, 26.6, 36.6, 39.6, 32.6, 22.6, 32.6, 23.6, 25.6, 21.6, 23.6, 41.6, 50.6, 45.6, 32.6, 37.6, 37.6, 32.6, 30.6, 31.6, 30.6, 28.6, 32.6, 32.6, 25.6, 26.6, 24.6, 16.6, 12.6, 11.6, 13.6, 8.6, 8.6, 5.6, 9.6, 8.6, 11.6, 9.6, 11.6, 10.6, 6.6, 10.6, 16.6, 7.6, 7.6, 9.6, 11.6, 2.6, 4.6, 8.6, 8.6, 2.6, 5.6, 1.6, 7.6, 4.6, 3.6, 5.6, 3.6, 7.6, 4.6, 5.6, 0.6000000000000001, 0.6000000000000001, 2.6, 4.6, 8.6, 3.6, 4.6, 5.6, 5.6, 2.6, 7.6, 0.6000000000000001, 3.6, 3.6, 2.6, 3.6, 3.6, 1.6, 3.6, 0.6000000000000001, 2.6, 2.6, 5.6, 3.6, -0.3999999999999999, 5.6, 1.6, 2.6, 2.6, 3.6, 0.6000000000000001, 3.6, 1.6, 0.6000000000000001, 1.6, 1.6, 1.6, 3.6, 1.6, 2.6, 1.6, 3.6, 1.6, 0.6000000000000001, 1.6, 3.6, -0.3999999999999999, 4.6, -0.3999999999999999, -0.3999999999999999, -0.3999999999999999, 3.6, 0.6000000000000001, 4.6, -1.4, 2.6, 0.6000000000000001, 0.6000000000000001, 0.6000000000000001, 0.6000000000000001, -0.3999999999999999, 0.6000000000000001, 1.6, 2.6, -0.3999999999999999, 0.6000000000000001, 1.6, 0.6000000000000001, 3.6, -0.3999999999999999, -0.3999999999999999, 1.6, -0.3999999999999999, 0.6000000000000001, 0.6000000000000001, 1.6, 1.6, -1.4, 2.6, -0.3999999999999999, -0.3999999999999999, 1.6, 1.6, 1.6, -0.3999999999999999, 1.6, -0.3999999999999999, -1.4, -1.4, 1.6, -0.3999999999999999, -1.4, 0.6000000000000001, 0.6000000000000001, 4.6, 0.6000000000000001, 0.6000000000000001, -0.3999999999999999, -0.3999999999999999, 0.6000000000000001, -0.3999999999999999, 0.6000000000000001, -1.4, 0.6000000000000001, 0.6000000000000001, 0.6000000000000001, -1.4, -0.3999999999999999, 1.6, 0.6000000000000001, -0.3999999999999999, 0.6000000000000001, 1.6, 0.6000000000000001, -0.3999999999999999, -0.3999999999999999, -0.3999999999999999, 0.6000000000000001, 1.6, 1.6, 0.6000000000000001, 0.6000000000000001, -1.4, -1.4, 1.6, 0.6000000000000001, -0.3999999999999999, 0.6000000000000001, 0.6000000000000001, -1.4, 1.6, -0.3999999999999999, 0.6000000000000001, 2.6, -1.4, 0.6000000000000001, 2.6, 0.6000000000000001, -0.3999999999999999, 0.6000000000000001, -0.3999999999999999, -0.3999999999999999, 0.6000000000000001, -1.4, 1.6, -0.3999999999999999, 0.6000000000000001, -0.3999999999999999, -0.3999999999999999, -0.3999999999999999, 2.6, -0.3999999999999999, 1.6, -0.3999999999999999, 0.6000000000000001, 0.6000000000000001, 1.6, -0.3999999999999999, -1.4, -1.4, -0.3999999999999999], [17633.1, 17673.1, 13273.1, 119.1, 160.1, 304.1, 408.1, 519.1, 552.1, 588.1, 584.1, 582.1, 591.1, 537.1, 551.1, 502.1, 484.1, 463.1, 448.1, 409.1, 404.1, 351.1, 329.1, 311.1, 265.1, 238.1, 242.1, 199.1, 213.1, 190.1, 170.1, 127.1, 147.1, 127.1, 121.1, 113.1, 103.1, 106.1, 78.1, 83.1, 88.1, 78.1, 64.1, 76.1, 78.1, 74.1, 56.1, 53.1, 63.1, 59.1, 43.1, 51.1, 60.1, 48.1, 43.1, 40.1, 41.1, 31.1, 37.1, 36.1, 29.1, 27.1, 30.1, 30.1, 25.1, 19.1, 21.1, 33.1, 115.1, 124.1, 36.1, 32.1, 37.1, 34.1, 30.1, 40.1, 32.1, 25.1, 37.1, 29.1, 29.1, 27.1, 13.1, 21.1, 10.1, 10.1, 16.1, 13.1, 6.1, 5.1, 13.1, 11.1, 9.1, 11.1, 12.1, 8.1, 6.1, 11.1, 6.1, 10.1, 4.1, 6.1, 5.1, -0.8999999999999999, 8.1, 9.1, 14.1, 5.1, 0.10000000000000009, 3.1, 2.1, 7.1, 3.1, 7.1, 3.1, 8.1, 6.1, 3.1, 9.1, 6.1, 3.1, 6.1, 8.1, 4.1, 2.1, 3.1, 5.1, 7.1, 4.1, 4.1, 5.1, -0.8999999999999999, 2.1, 3.1, 3.1, 2.1, 3.1, 4.1, 0.10000000000000009, 11.1, 0.10000000000000009, 3.1, 4.1, 3.1, 4.1, 3.1, 3.1, 3.1, -0.8999999999999999, -0.8999999999999999, 3.1, 0.10000000000000009, 3.1, 3.1, 1.1, 1.1, 0.10000000000000009, 0.10000000000000009, 2.1, 4.1, 1.1, 4.1, -1.9, 5.1, 2.1, 2.1, 0.10000000000000009, -0.8999999999999999, 0.10000000000000009, 4.1, 2.1, 3.1, 0.10000000000000009, 0.10000000000000009, 1.1, -0.8999999999999999, 0.10000000000000009, 0.10000000000000009, 2.1, 2.1, 1.1, -0.8999999999999999, 2.1, -1.9, -1.9, 2.1, 2.1, 1.1, -1.9, 3.1, 1.1, 3.1, 1.1, 0.10000000000000009, -0.8999999999999999, 0.10000000000000009, -0.8999999999999999, 0.10000000000000009, -1.9, -0.8999999999999999, 2.1, 3.1, 0.10000000000000009, 0.10000000000000009, -1.9, -0.8999999999999999, 1.1, 0.10000000000000009, -0.8999999999999999, -1.9, 0.10000000000000009, 0.10000000000000009, -0.8999999999999999, 0.10000000000000009, -0.8999999999999999, 0.10000000000000009, -0.8999999999999999, 0.10000000000000009, 0.10000000000000009, -0.8999999999999999, 2.1, 3.1, 3.1, -0.8999999999999999, 1.1, -1.9, -0.8999999999999999, -0.8999999999999999, -0.8999999999999999, -1.9, 0.10000000000000009, -0.8999999999999999, 0.10000000000000009, 0.10000000000000009, -0.8999999999999999, -0.8999999999999999, -1.9, -0.8999999999999999, -1.9, 2.1, 0.10000000000000009, -1.9, 0.10000000000000009, -0.8999999999999999, -0.8999999999999999, -1.9, -0.8999999999999999, -0.8999999999999999, 2.1, -0.8999999999999999, -0.8999999999999999, -0.8999999999999999, 1.1, 0.10000000000000009, 2.1, 1.1, 0.10000000000000009, -0.8999999999999999, 2.1, 1.1, -1.9, -1.9, 0.10000000000000009, 1.1, -0.8999999999999999, -0.8999999999999999, 1.1, 0.10000000000000009, -0.8999999999999999, 0.10000000000000009, -0.8999999999999999, 0.10000000000000009, -0.8999999999999999, 2.1, -0.8999999999999999, -0.8999999999999999, 0.10000000000000009, 0.10000000000000009, 1.1], [18619.1, 18688.1, 13301.1, 100.1, 146.1, 240.1, 373.1, 501.1, 528.1, 550.1, 521.1, 579.1, 542.1, 593.1, 538.1, 466.1, 457.1, 479.1, 416.1, 432.1, 344.1, 347.1, 321.1, 282.1, 258.1, 232.1, 226.1, 201.1, 190.1, 169.1, 179.1, 138.1, 145.1, 134.1, 111.1, 114.1, 109.1, 125.1, 115.1, 81.1, 75.1, 86.1, 80.1, 70.1, 70.1, 62.1, 62.1, 64.1, 55.1, 36.1, 51.1, 50.1, 45.1, 44.1, 45.1, 47.1, 38.1, 37.1, 33.1, 30.1, 27.1, 25.1, 26.1, 31.1, 22.1, 28.1, 21.1, 29.1, 99.1, 177.1, 58.1, 26.1, 42.1, 33.1, 40.1, 31.1, 35.1, 26.1, 25.1, 28.1, 23.1, 14.1, 17.1, 15.1, 16.1, 8.1, 12.1, 9.1, 15.1, 10.1, 2.1, 11.1, 2.1, 8.1, 5.1, 18.1, 11.1, 12.1, 11.1, 11.1, 4.1, 11.1, 7.1, 7.1, 4.1, 7.1, 5.1, 9.1, 0.10000000000000009, 2.1, 7.1, 4.1, 1.1, 8.1, 3.1, 4.1, 2.1, 7.1, 6.1, 1.1, 3.1, -0.8999999999999999, 5.1, 2.1, 8.1, 4.1, 2.1, 0.10000000000000009, 2.1, 4.1, 0.10000000000000009, 4.1, -0.8999999999999999, 0.10000000000000009, 5.1, 2.1, 4.1, 2.1, 4.1, 0.10000000000000009, 5.1, 4.1, -0.8999999999999999, 1.1, -0.8999999999999999, 2.1, 2.1, 5.1, 3.1, 1.1, 6.1, 2.1, 2.1, 0.10000000000000009, 1.1, 1.1, 5.1, -0.8999999999999999, 0.10000000000000009, 5.1, 2.1, 1.1, -0.8999999999999999, 1.1, 3.1, 5.1, -0.8999999999999999, 1.1, 2.1, 0.10000000000000009, 4.1, 0.10000000000000009, 3.1, 0.10000000000000009, 1.1, -0.8999999999999999, 1.1, 0.10000000000000009, 1.1, 2.1, -1.9, -1.9, 2.1, 2.1, 0.10000000000000009, -0.8999999999999999, 1.1, 1.1, 1.1, 0.10000000000000009, 2.1, -0.8999999999999999, -0.8999999999999999, 0.10000000000000009, 2.1, 1.1, 1.1, -1.9, 1.1, -1.9, 0.10000000000000009, 1.1, 0.10000000000000009, 0.10000000000000009, 1.1, 0.10000000000000009, 0.10000000000000009, -0.8999999999999999, 1.1, 0.10000000000000009, 1.1, 1.1, 1.1, 0.10000000000000009, 0.10000000000000009, -0.8999999999999999, 0.10000000000000009, -0.8999999999999999, 2.1, -0.8999999999999999, -0.8999999999999999, 0.10000000000000009, -0.8999999999999999, -1.9, -0.8999999999999999, -0.8999999999999999, 0.10000000000000009, 2.1, 1.1, -0.8999999999999999, -0.8999999999999999, -0.8999999999999999, -1.9, -1.9, 4.1, -0.8999999999999999, 4.1, 0.10000000000000009, -1.9, -0.8999999999999999, -0.8999999999999999, 2.1, 0.10000000000000009, -0.8999999999999999, 0.10000000000000009, 1.1, 2.1, 1.1, 1.1, 0.10000000000000009, 0.10000000000000009, 0.10000000000000009, 3.1, -0.8999999999999999, 2.1, 2.1, 2.1, 0.10000000000000009, 0.10000000000000009, -1.9, 0.10000000000000009, 0.10000000000000009, 0.10000000000000009, -1.9, 0.10000000000000009, -1.9, 2.1, -1.9, 1.1, -0.8999999999999999, -0.8999999999999999, -0.8999999999999999, 2.1, -0.8999999999999999, -0.8999999999999999, 1.1, -1.9, -0.8999999999999999, 4.1], [18654.9, 18674.9, 13816.9, 87.9, 177.9, 202.9, 300.9, 434.9, 539.9, 579.9, 550.9, 583.9, 598.9, 569.9, 526.9, 522.9, 513.9, 444.9, 411.9, 378.9, 323.9, 304.9, 264.9, 255.9, 239.9, 250.9, 214.9, 165.9, 193.9, 159.9, 166.9, 138.9, 111.9, 108.9, 115.9, 110.9, 91.9, 86.9, 85.9, 64.9, 80.9, 42.9, 71.9, 60.9, 64.9, 68.9, 61.9, 50.9, 61.9, 55.9, 39.9, 41.9, 64.9, 29.9, 43.9, 38.9, 36.9, 31.9, 29.9, 30.9, 23.9, 24.9, 16.9, 16.9, 18.9, 19.9, 35.9, 16.9, 18.9, 16.9, 21.9, 40.9, 28.9, 29.9, 30.9, 26.9, 23.9, 24.9, 37.9, 29.9, 14.9, 13.9, 15.9, 11.9, 13.9, 13.9, 8.9, 4.9, 9.9, 16.9, 12.9, 3.9, 8.9, 10.9, 7.9, 10.9, 1.9, 8.9, 3.9, 6.9, 6.9, 2.9, 7.9, 8.9, 5.9, 5.9, 6.9, 2.9, 6.9, 2.9, 2.9, 2.9, 2.9, 5.9, 4.9, 2.9, 5.9, 3.9, 6.9, 2.9, 5.9, -1.1, 1.9, -0.10000000000000009, 3.9, 0.8999999999999999, 3.9, 6.9, -0.10000000000000009, 0.8999999999999999, 3.9, 1.9, 5.9, 1.9, 5.9, 3.9, 1.9, 4.9, -1.1, 4.9, 1.9, 1.9, 1.9, 2.9, -1.1, -2.1, 1.9, -1.1, 0.8999999999999999, 0.8999999999999999, 2.9, 2.9, 1.9, 4.9, -1.1, 0.8999999999999999, -0.10000000000000009, -0.10000000000000009, -0.10000000000000009, 0.8999999999999999, -0.10000000000000009, 1.9, 2.9, 0.8999999999999999, 1.9, -0.10000000000000009, 2.9, -0.10000000000000009, 1.9, 0.8999999999999999, 3.9, 1.9, 0.8999999999999999, -0.10000000000000009, -1.1, -2.1, 3.9, 0.8999999999999999, 0.8999999999999999, 1.9, 5.9, -0.10000000000000009, 0.8999999999999999, 2.9, 1.9, -1.1, 3.9, 0.8999999999999999, -0.10000000000000009, 3.9, 0.8999999999999999, -0.10000000000000009, -2.1, -1.1, -2.1, -0.10000000000000009, -0.10000000000000009, -1.1, -0.10000000000000009, -0.10000000000000009, 1.9, -0.10000000000000009, -2.1, -1.1, -0.10000000000000009, -0.10000000000000009, 0.8999999999999999, 0.8999999999999999, 1.9, 0.8999999999999999, 0.8999999999999999, -0.10000000000000009, 3.9, -0.10000000000000009, 0.8999999999999999, -1.1, 1.9, -1.1, -1.1, -0.10000000000000009, -0.10000000000000009, 0.8999999999999999, -2.1, -1.1, 2.9, 1.9, -1.1, 1.9, -2.1, -0.10000000000000009, -2.1, -1.1, -1.1, -1.1, -1.1, -0.10000000000000009, 0.8999999999999999, -2.1, 0.8999999999999999, -1.1, 1.9, -0.10000000000000009, 5.9, -0.10000000000000009, -2.1, 1.9, 1.9, -0.10000000000000009, -2.1, -0.10000000000000009, 0.8999999999999999, -0.10000000000000009, 2.9, -0.10000000000000009, 0.8999999999999999, -2.1, -2.1, -0.10000000000000009, -1.1, -2.1, -2.1, -0.10000000000000009, -2.1, -2.1, -0.10000000000000009, -1.1, 0.8999999999999999, -0.10000000000000009, -0.10000000000000009, 0.8999999999999999, 0.8999999999999999, -1.1, -0.10000000000000009, -1.1, 0.8999999999999999, -1.1, 0.8999999999999999, -0.10000000000000009, -0.10000000000000009], [18976.7, 19074.7, 13689.7, 111.7, 150.7, 226.7, 284.7, 434.7, 461.7, 523.7, 525.7, 542.7, 525.7, 539.7, 542.7, 497.7, 470.7, 435.7, 387.7, 338.7, 320.7, 297.7, 300.7, 270.7, 245.7, 201.7, 205.7, 215.7, 175.7, 174.7, 150.7, 150.7, 100.7, 106.7, 89.7, 94.7, 95.7, 97.7, 88.7, 85.7, 93.7, 69.7, 77.7, 65.7, 56.7, 69.7, 55.7, 56.7, 67.7, 51.7, 42.7, 50.7, 51.7, 38.7, 38.7, 37.7, 31.7, 38.7, 27.7, 32.7, 34.7, 19.7, 22.7, 17.7, 20.7, 26.7, 29.7, 23.7, 50.7, 44.7, 26.7, 24.7, 27.7, 31.7, 28.7, 21.7, 28.7, 25.7, 29.7, 31.7, 17.7, 13.7, 14.7, 14.7, 8.7, 7.7, 10.7, 13.7, 15.7, 10.7, 8.7, 7.7, 8.7, 9.7, 5.7, 4.7, 14.7, 11.7, 13.7, 7.7, 7.7, 6.7, 8.7, 4.7, 4.7, 3.7, 5.7, 9.7, 9.7, 6.7, 4.7, 4.7, 7.7, 7.7, 6.7, 8.7, 1.7, 1.7, 0.7, 1.7, 2.7, 3.7, 3.7, 2.7, 0.7, 5.7, 7.7, 0.7, 4.7, 4.7, 3.7, 4.7, 0.7, 2.7, 3.7, 4.7, 1.7, 2.7, 1.7, 0.7, 1.7, 2.7, 1.7, 3.7, 2.7, 2.7, 3.7, 3.7, 1.7, 3.7, 2.7, 3.7, -0.30000000000000004, 0.7, 4.7, -0.30000000000000004, 0.7, 2.7, 1.7, 1.7, 0.7, 1.7, 3.7, 0.7, 1.7, 2.7, 2.7, 1.7, 1.7, 3.7, 0.7, 1.7, 0.7, 1.7, 0.7, -1.3, 1.7, 2.7, 2.7, 2.7, 2.7, 1.7, 1.7, 2.7, 2.7, 0.7, 0.7, 2.7, -0.30000000000000004, 1.7, -0.30000000000000004, 1.7, 0.7, 1.7, 1.7, -0.30000000000000004, 1.7, 0.7, 2.7, -1.3, 1.7, 0.7, -0.30000000000000004, 0.7, -1.3, -1.3, 1.7, 4.7, 0.7, 3.7, 1.7, 4.7, -1.3, 0.7, 1.7, 0.7, -0.30000000000000004, 2.7, 0.7, -0.30000000000000004, -0.30000000000000004, 0.7, 0.7, 0.7, 1.7, -1.3, -0.30000000000000004, 1.7, 0.7, -0.30000000000000004, 0.7, 0.7, 0.7, -0.30000000000000004, -0.30000000000000004, 3.7, 2.7, 0.7, 0.7, 0.7, 1.7, 1.7, 0.7, -1.3, 3.7, -0.30000000000000004, 1.7, 0.7, -1.3, 1.7, -0.30000000000000004, 2.7, 1.7, -0.30000000000000004, -0.30000000000000004, -1.3, 1.7, 0.7, 1.7, 4.7, 1.7, -0.30000000000000004, -1.3, -0.30000000000000004, 3.7, -1.3, 0.7, -0.30000000000000004, 0.7, -0.30000000000000004, 1.7, -0.30000000000000004, 1.7, -0.30000000000000004, -1.3, -0.30000000000000004, -1.3, -0.30000000000000004, 0.7], [17594.3, 17546.3, 13773.3, 117.3, 224.3, 547.3, 765.3, 909.3, 872.3, 906.3, 880.3, 804.3, 768.3, 745.3, 718.3, 637.3, 571.3, 524.3, 459.3, 417.3, 379.3, 331.3, 361.3, 274.3, 263.3, 263.3, 223.3, 197.3, 181.3, 162.3, 158.3, 157.3, 135.3, 108.3, 121.3, 101.3, 104.3, 91.3, 95.3, 79.3, 80.3, 70.3, 77.3, 58.3, 64.3, 59.3, 57.3, 55.3, 58.3, 40.3, 40.3, 41.3, 49.3, 37.3, 37.3, 33.3, 37.3, 27.3, 22.3, 30.3, 25.3, 20.3, 21.3, 19.3, 20.3, 16.3, 17.3, 19.3, 29.3, 20.3, 24.3, 22.3, 23.3, 28.3, 21.3, 23.3, 25.3, 28.3, 21.3, 23.3, 11.3, 18.3, 10.3, 10.3, 12.3, 10.3, 5.3, 12.3, 11.3, 5.3, 4.3, 12.3, 4.3, 11.3, 12.3, 10.3, 8.3, 8.3, 6.3, 8.3, 7.3, 19.3, 10.3, 6.3, 4.3, 10.3, 9.3, 6.3, 2.3, 7.3, 10.3, 9.3, 0.30000000000000004, 3.3, 9.3, 2.3, 1.3, 9.3, -0.7, 9.3, 4.3, 7.3, 1.3, 2.3, 0.30000000000000004, 2.3, 4.3, 9.3, 4.3, 6.3, 8.3, 5.3, 8.3, 3.3, 3.3, 4.3, 2.3, 2.3, 0.30000000000000004, 1.3, 10.3, 6.3, 1.3, 3.3, 1.3, 4.3, 0.30000000000000004, 0.30000000000000004, -0.7, 2.3, 2.3, 2.3, 2.3, 3.3, 4.3, 2.3, 3.3, 1.3, -0.7, 1.3, 0.30000000000000004, 4.3, -1.7, 0.30000000000000004, 2.3, 0.30000000000000004, 1.3, 0.30000000000000004, 1.3, 4.3, 0.30000000000000004, -0.7, 4.3, 3.3, 4.3, -0.7, -0.7, 2.3, -0.7, -0.7, 2.3, 0.30000000000000004, 0.30000000000000004, 3.3, 3.3, -0.7, -0.7, 1.3, 1.3, 3.3, 1.3, 2.3, 0.30000000000000004, 1.3, 1.3, -0.7, 0.30000000000000004, 0.30000000000000004, 0.30000000000000004, 0.30000000000000004, -0.7, 3.3, 1.3, -0.7, 1.3, 0.30000000000000004, 0.30000000000000004, -0.7, 0.30000000000000004, 0.30000000000000004, -0.7, 0.30000000000000004, 0.30000000000000004, -0.7, -1.7, -0.7, -1.7, -0.7, -0.7, 2.3, 1.3, 0.30000000000000004, 2.3, 0.30000000000000004, -1.7, 5.3, -1.7, 2.3, -1.7, 0.30000000000000004, 0.30000000000000004, 0.30000000000000004, 0.30000000000000004, 1.3, -0.7, 0.30000000000000004, -0.7, -0.7, -0.7, 0.30000000000000004, -1.7, -0.7, -0.7, 1.3, -1.7, -0.7, -0.7, 0.30000000000000004, 0.30000000000000004, -1.7, 0.30000000000000004, 1.3, 0.30000000000000004, -0.7, 0.30000000000000004, -0.7, 0.30000000000000004, -1.7, 1.3, 2.3, 0.30000000000000004, -0.7, 1.3, -0.7, -0.7, -0.7, 0.30000000000000004, -0.7, 0.30000000000000004, 0.30000000000000004, -0.7, 0.30000000000000004, 1.3, -0.7, 0.30000000000000004, -1.7, 1.3, -0.7, 0.30000000000000004], [18616.4, 18519.4, 13914.4, 118.4, 232.4, 502.4, 866.4, 940.4, 867.4, 832.4, 821.4, 863.4, 699.4, 742.4, 695.4, 681.4, 611.4, 503.4, 479.4, 424.4, 442.4, 377.4, 297.4, 314.4, 262.4, 270.4, 236.4, 208.4, 198.4, 160.4, 151.4, 140.4, 141.4, 120.4, 109.4, 96.4, 110.4, 94.4, 70.4, 97.4, 70.4, 69.4, 71.4, 66.4, 66.4, 58.4, 55.4, 59.4, 55.4, 46.4, 41.4, 53.4, 46.4, 43.4, 41.4, 33.4, 29.4, 33.4, 29.4, 25.4, 20.4, 25.4, 21.4, 15.4, 20.4, 33.4, 26.4, 27.4, 27.4, 23.4, 20.4, 26.4, 29.4, 17.4, 14.4, 32.4, 47.4, 26.4, 15.4, 22.4, 16.4, 15.4, 18.4, 18.4, 19.4, 6.4, 13.4, 12.4, 5.4, 7.4, 13.4, 9.4, 7.4, 8.4, 10.4, 15.4, 13.4, 8.4, 10.4, 7.4, 16.4, 16.4, 13.4, 11.4, 5.4, 5.4, 6.4, 6.4, 5.4, 12.4, 5.4, 5.4, 8.4, 3.4, 6.4, 1.4, 5.4, 2.4, 6.4, 2.4, 5.4, 5.4, 1.4, 6.4, 5.4, 2.4, 2.4, 3.4, 1.4, 0.3999999999999999, 8.4, 6.4, 5.4, -0.6000000000000001, 3.4, 5.4, 2.4, 4.4, 6.4, -0.6000000000000001, 0.3999999999999999, -0.6000000000000001, 6.4, 0.3999999999999999, 4.4, 6.4, 5.4, 1.4, 5.4, 1.4, 1.4, 3.4, -0.6000000000000001, 1.4, -1.6, 3.4, 3.4, 5.4, 1.4, 1.4, -0.6000000000000001, 3.4, -0.6000000000000001, 2.4, 0.3999999999999999, 1.4, 0.3999999999999999, 1.4, 0.3999999999999999, -0.6000000000000001, 3.4, 1.4, -1.6, 0.3999999999999999, -0.6000000000000001, 0.3999999999999999, -0.6000000000000001, -1.6, -0.6000000000000001, 1.4, 0.3999999999999999, 0.3999999999999999, 3.4, 1.4, 1.4, -0.6000000000000001, -0.6000000000000001, -1.6, 0.3999999999999999, -0.6000000000000001, 3.4, -0.6000000000000001, 0.3999999999999999, -0.6000000000000001, 2.4, 2.4, 2.4, 0.3999999999999999, 0.3999999999999999, 1.4, 1.4, 1.4, -0.6000000000000001, 0.3999999999999999, 4.4, -0.6000000000000001, 0.3999999999999999, -0.6000000000000001, 2.4, 0.3999999999999999, 0.3999999999999999, 0.3999999999999999, -1.6, -0.6000000000000001, 2.4, -0.6000000000000001, 3.4, 0.3999999999999999, 2.4, 2.4, -0.6000000000000001, 0.3999999999999999, -0.6000000000000001, -0.6000000000000001, -0.6000000000000001, -1.6, -1.6, 0.3999999999999999, 2.4, -1.6, -0.6000000000000001, 0.3999999999999999, -1.6, 0.3999999999999999, 0.3999999999999999, -0.6000000000000001, -0.6000000000000001, 1.4, 0.3999999999999999, 1.4, 0.3999999999999999, 0.3999999999999999, 0.3999999999999999, -0.6000000000000001, 1.4, 4.4, -1.6, -0.6000000000000001, -1.6, 0.3999999999999999, -1.6, 0.3999999999999999, 0.3999999999999999, 2.4, 3.4, 1.4, -0.6000000000000001, 0.3999999999999999, 0.3999999999999999, -0.6000000000000001, 1.4, 0.3999999999999999, -0.6000000000000001, -0.6000000000000001, -0.6000000000000001, 0.3999999999999999, -1.6, 2.4, 0.3999999999999999, -0.6000000000000001, -1.6, 0.3999999999999999, -1.6, 0.3999999999999999, -0.6000000000000001, -0.6000000000000001, 0.3999999999999999, 2.4, 1.4]]
  in  "?":T1(tab)=enum."Raw Counts far"
  out "NRB":dbl[][](graph)=[[0.003961842600932212, 0.013051074816415641, 0.010858466862098867, 0.00021951418804836656, 0.00048452377151986947, 0.0008443870166457608, 0.001238879302351734, 0.00172727750403078, 0.0025362072077704475, 0.003726245329745556, 0.005170533167390487, 0.007206066556166077, 0.009635756794465189, 0.012129519317002879, 0.014477004652397188, 0.016794499043595167, 0.019652915616501884, 0.022538120487975717, 0.025313486781851594, 0.028619643827708114, 0.031888990965589926, 0.034517444485275176, 0.0367906791814455, 0.039716931671749486, 0.04296873847827615, 0.045774093090992146, 0.048744516571550066, 0.050773919152275124, 0.052417319738859165, 0.053016454525943, 0.0526834903480619, 0.05320797660795933, 0.053526115452312915, 0.05236762506095251, 0.05130924391748835, 0.05314848243831867, 0.05397318746392932, 0.054057646504209286, 0.055697110372541214, 0.05531537945239545, 0.05450573245843037, 0.053995970253363355, 0.053002488060428433, 0.05370530293095405, 0.053042373514835206, 0.05206210964169696, 0.052450933615806064, 0.05315852347394766, 0.053193583599966676, 0.052641806348536685, 0.05416730353838234, 0.05601935320289867, 0.058275823565837284, 0.05695714317169725, 0.05364621988637239, 0.05156105293310504, 0.048750479217275676, 0.04753719593641571, 0.047858579297538464, 0.04525846524897866, 0.04178374376478684, 0.04055686625542295, 0.03800852809796118, 0.038249213645015066, 0.04183224059190708, 0.044166766469529356, 0.0470056645634688, 0.06711181730172716, 0.09591785634625702, 0.0895166666206842, 0.0672318754089738, 0.06502250113398857, 0.0684954070305699, 0.0684478541099905, 0.06803642356624809, 0.06769475674540076, 0.06888875682821222, 0.0694600597095466, 0.06436039677096586, 0.05666982440905235, 0.05217705468206588, 0.046971695294495526, 0.042656580960271084, 0.04343609170640711, 0.04312108541926721, 0.03827198528813693, 0.03392505822211576, 0.03253064966142212, 0.030874233700402695, 0.02970211930891976, 0.029947676031988172, 0.02957152350255454, 0.02753511030068474, 0.027684281271117855, 0.028146239436553387, 0.027811210562454933, 0.029004464405071144, 0.030298353629432548, 0.029717966927168514, 0.02873443145616173, 0.03100440497563779, 0.030045396411648616, 0.028341657458681863, 0.028504565205114935, 0.028180594499924508, 0.02920620263052312, 0.02819079377001229, 0.02543903946000797, 0.02694067221240294, 0.03171387026899185, 0.03158212470716164, 0.027448786965273305, 0.02388872408081428, 0.02206374806885885, 0.0251233785033342, 0.026435698148335168, 0.023141544231533518, 0.022434109160955586, 0.02312237080419315, 0.024343504780048413, 0.02432852202659332, 0.02269262865222648, 0.02186586901908458, 0.022333755756307045, 0.019652694123838164, 0.01905237019657747, 0.021217238244350206, 0.02013467497890564, 0.01985040635068856, 0.020037469295420066, 0.02022315320399282, 0.02103575184913102, 0.02059021083006454, 0.019605964726734877, 0.019111023516254582, 0.02032898298757211, 0.0198168370389047, 0.01942044115804922, 0.017891408272449706, 0.016877541618261, 0.020417372260953744, 0.019544591653461528, 0.01701869200520285, 0.016210697290593858, 0.016436627629954466, 0.018662655311665437, 0.017204870965539007, 0.014438263212123308, 0.014313806326798248, 0.015642476037701792, 0.014042885406117317, 0.01239662141510811, 0.013404394749873996, 0.015803703197763055, 0.016529419196279118, 0.014286231843443303, 0.01535881670700328, 0.015735133807332914, 0.012653082156830222, 0.008935633342175477, 0.010169308124959881, 0.013324331241774326, 0.012914496144511836, 0.012103585136079033, 0.013037016218459152, 0.01518283976958455, 0.017377663967772104, 0.01575444548889581, 0.012028944066510032, 0.011338027267904041, 0.01168269029461451, 0.013526580419507992, 0.014331858894481688, 0.014498023986412097, 0.014002552911960259, 0.010365328776495238, 0.011161270104915352, 0.01425825369763266, 0.011877076801889545, 0.01084183407665437, 0.01143516734074261, 0.01203964198139985, 0.011447757221440496, 0.012061539170481476, 0.010465225355264935, 0.009830169600040291, 0.010440533757824716, 0.009023133161404672, 0.011180281354723534, 0.008174755301911158, 0.0069455709965262815, 0.012601454872082845, 0.01112126288842154, 0.007436891405158593, 0.009433349992653746, 0.0075910197741676155, 0.00654915444848017, 0.007181270191410626, 0.00811076902045925, 0.012231088800894007, 0.01177097680959652, 0.009239964413827781, 0.007251351350307669, 0.005522229638963633, 0.007394938981695256, 0.008079335840809991, 0.006303872349082529, 0.01042104558396347, 0.010206471276199726, 0.004261662710765189, 0.006549854158871927, 0.00823270603720945, 0.006020233479674669, 0.0054163591282148735, 0.004133654438571071, 0.004845134134027975, 0.012021568510564299, 0.0111044239126878, 0.004288895630682686, 0.002582926371369708, 0.002606460886447684, 0.007250578656495677, 0.005881520724233502, 0.0008684435727611659, 0.003066757181283906, 0.007145868773258068, 0.0042363516738209645, 0.0012746268470077554, 0.0031767666833325305, 0.0032045719484428375, 0.007080730867088101, 0.007142168591108674, 0.0032887146788093246, 0.0060811871558024986, 0.008522876069431933, 0.00136564359939489, -0.0022683917396588717, -0.0006535935072729, 0.0005767107421962387, 0.005150859830431448, 0.003937287526636484, 0.0027029967739010713, 0.0005961764082552068, -0.001975017490684558, -0.000692605576478635, 0.0014838280677424089, 0.001935892142976152, -0.002040302938508854, -0.0007154058866680866, 0.0010817467175058364, 0.0024534425930784736, 0.00430491050587151, 0.0020310859083046856, 0.0025124411094276425, -0.002626042352032583, -0.004537159087849791, -0.00028579291175139567, -0.0026881950499146, -0.0017415486632951151, -0.0002925040626564276, 0.0011790346902914401, -0.00029702143309153677, -0.0032922184696705286, 0.001206294707572589, -0.0008102994853513068, -0.0008164264917837962, 0.005346766001957353, 0.005386891684896477, 0.0017742627207665473, -0.0003154370734859993, 0.0012711129708855384, 0.0028811526294236257, 0.0002149905472429408, -0.0024905336792971295, -0.0019633669393970417, -0.0025270245291989187, 0.0013280215022000853, 0.0, 0.0, 0.0]] caption="Water Vapor Number Density"
  out "NRB 2":dbl[][](graph)=[[0.003988903663970116, 0.013550702370854173, 0.012065081846482703, 0.0004394509176526181, 0.0011625538196166428, 0.002582554348974244, 0.004650531265063094, 0.007007505685040279, 0.009431126233211769, 0.011859542617438693, 0.01448481417333002, 0.01714797341627186, 0.0193735012413644, 0.021611617366321282, 0.023405249573866253, 0.024899360244024876, 0.026177372823358604, 0.0271196654809561, 0.027911090207824348, 0.028436864878968876, 0.028263031565344217, 0.027893905337575155, 0.02770565221947318, 0.027589932681669743, 0.02793749153970001, 0.028148005588714255, 0.027628322480772884, 0.027461691997907153, 0.027548765774014855, 0.02717159281818379, 0.026443138734315346, 0.025453469191017746, 0.024984070454531607, 0.02420794565399193, 0.024378699878903197, 0.024630950671828102, 0.02419912945828684, 0.023814732743300347, 0.023140707080925606, 0.023037236352545613, 0.023062692305958216, 0.02309349476662312, 0.023071715937141222, 0.023276857559674884, 0.02379146366936723, 0.02330271087319686, 0.022461457864406616, 0.022961826007357213, 0.02257692170621881, 0.021649511900276575, 0.022580463084716115, 0.024469862206415467, 0.023717256845124463, 0.021611643949487926, 0.021044349897883223, 0.020617284252503983, 0.020188068848097925, 0.02044147332806986, 0.020172925194438543, 0.018239273845897824, 0.017536918449700335, 0.017839294763123723, 0.0167873157688366, 0.016290281225465195, 0.0177481783437778, 0.018769843359418528, 0.019666776766910418, 0.028164636246010996, 0.03944273751935134, 0.03543192678131093, 0.026558372870720146, 0.026638556059193273, 0.028075693122013023, 0.028573607873330843, 0.02955399657347168, 0.030597387685635538, 0.030252945446491243, 0.02955148246287524, 0.02977377105024874, 0.026053763001677114, 0.02273349095052214, 0.021988670793275687, 0.019149138723361388, 0.01706855671759974, 0.015028044298589302, 0.014583538669354083, 0.015852754117703646, 0.015213874476485511, 0.013790525895337169, 0.012758463008787902, 0.013342194805833476, 0.0129044790896195, 0.014496543308392253, 0.015765933603797317, 0.015517317268759594, 0.015446889019556372, 0.014752430949334636, 0.01602794409261325, 0.015791190833471063, 0.01445293994130676, 0.014375573175088082, 0.01556210859889397, 0.013496729510699931, 0.010795769053291236, 0.012356131758954936, 0.015672050259842148, 0.013987355407314194, 0.01138981371761689, 0.012201530119934243, 0.01373546174544363, 0.01478609722037933, 0.012339597251738551, 0.011547916453037602, 0.01269050232117191, 0.01253259476854113, 0.011101709346424815, 0.011392669688214363, 0.013295420415042463, 0.012296145722122275, 0.011153566427368417, 0.010706682857882944, 0.011313761248577657, 0.009754218983931901, 0.008915445843494752, 0.010637446725205163, 0.010350334941848447, 0.011911151956332765, 0.011863143164791786, 0.009888957870570803, 0.011139813171697476, 0.012178212894084245, 0.01148521329607437, 0.011659890839890925, 0.011706387894673142, 0.010304501804416607, 0.0092571984646083, 0.0102059987146353, 0.008844753006552079, 0.0070226346631023255, 0.009102980410019992, 0.010093767466255692, 0.009801185876390783, 0.009939716821380435, 0.007836036626067943, 0.00673221801689597, 0.008516399645489382, 0.008477621104649728, 0.007803513660204015, 0.008709873948092398, 0.010287582281446111, 0.009109702961005973, 0.007397915104036361, 0.009014972958544202, 0.008449056335162457, 0.006653238258986829, 0.008143416013506006, 0.00895921131467363, 0.0058330661016684935, 0.006818740812347128, 0.008566381079296258, 0.009421547181940654, 0.008592612021820394, 0.007740968080457038, 0.008612115851721, 0.008913803623459084, 0.007432349267237744, 0.00551087551582801, 0.005373527335857202, 0.0056436629354786405, 0.007794850262126972, 0.007043305483113002, 0.004352344782077432, 0.006561501863645563, 0.007729294291351213, 0.0031803438582356353, 0.0034401839787646807, 0.005738747253764722, 0.0058037750323432415, 0.0067934555074496755, 0.006869572062088245, 0.002693376826289675, 0.004395381564757591, 0.009032586173992047, 0.008399086417040243, 0.0030605563757129636, 0.001846257326803409, 0.00615332373320033, 0.004689963954377258, 0.0062856494916540065, 0.007393715940578716, 0.004314657418422362, 0.0046258076011028906, 0.0052113765557364276, 0.005808360821674596, 0.005045718633012542, 0.004543512496535553, 0.004030235585118915, 0.001526716913084968, -0.0007425280910033846, 0.0018461818001865812, 0.006817804969743297, 0.006885812578535321, 0.0051710315059095326, 0.003421372058327619, 0.0007273659545921828, 0.0022646483963530313, 0.004140767581890091, 0.006364921736472352, 0.004536182859480515, 0.0007632799190366503, 0.00462341514816355, 0.007260327610329335, 0.0030755439060461396, 0.0011228987359393245, 0.0021334938428406174, 0.0018169193015226074, 0.0028525515465482967, 0.0035643580277486923, 0.006018293141180983, 0.004677195522963907, 0.004719812118534713, 0.004051780577725353, 0.0015779624176307998, 0.0015921462781685338, 0.001971483617103523, 0.001252362124133918, 0.0031215173106688868, 0.0038988634734973488, 0.0001512741475782408, 0.001297085840055686, 0.0016932102509038397, -0.0025618446960600067, -0.004150019200274745, -0.003395961921942926, -0.0010354817763607459, 0.006185578734545382, 0.005022889439515602, -0.0018790783384070582, -0.0014829672721145214, -0.0002492340464667618, 0.00016754359690875122, 0.004814716292385108, 0.002725379727980436, -0.00025761107969522794, 0.003636186934986123, 0.0027930884455022774, 0.0028158426361895774, 0.003282235247650506, -0.0007154053572609187, -0.0002704362483363295, 0.006088181717815063, 0.00888462124608677, 0.006647204245609954, 0.008560935787703802, 0.006283773530593553, 0.0016069152668032045, 0.0025721386948359616, 0.004512343330513241, 0.004547390525721994, -0.0012675159453505915, -0.00717242102094157, -0.006732455924221976, -0.004289854813698413, 0.00020104885470553666, -0.001316735314530256, -0.0018369572014799284, 0.0027761994188581353, 0.004350945279774149, 0.0033397890310825295, 0.0007360197124427317, 0.0002118518844471613, -0.0008536725206301811, -0.0013974363297490288, -0.0003248523484815737, -0.002508744074253828, -0.0036257260992692314, -0.00033200484637757247, 0.0, 0.0, 0.0]] caption="Water Vapor Number Density"
  out "raw counts":dbl[][](graph)=[[16897.1, 18435.1, 11496.1, 29.1, 47.1, 65.1, 95.1, 94.1, 86.1, 128.1, 128.1, 158.1, 205.1, 190.1, 194.1, 234.1, 223.1, 240.1, 268.1, 251.1, 278.1, 273.1, 261.1, 275.1, 277.1, 284.1, 254.1, 225.1, 256.1, 233.1, 238.1, 207.1, 215.1, 208.1, 178.1, 177.1, 185.1, 151.1, 174.1, 159.1, 131.1, 149.1, 135.1, 131.1, 124.1, 114.1, 116.1, 107.1, 113.1, 92.1, 98.1, 85.1, 95.1, 91.1, 75.1, 74.1, 65.1, 61.1, 56.1, 45.1, 53.1, 47.1, 43.1, 40.1, 41.1, 40.1, 47.1, 41.1, 37.1, 59.1, 44.1, 52.1, 56.1, 62.1, 45.1, 30.1, 40.1, 38.1, 39.1, 29.1, 20.1, 29.1, 22.1, 22.1, 26.1, 16.1, 15.1, 19.1, 10.1, 21.1, 21.1, 22.1, 14.1, 15.1, 15.1, 17.1, 14.1, 10.1, 17.1, 13.1, 12.1, 19.1, 5.1, 18.1, 17.1, 18.1, 10.1, 14.1, 15.1, 20.1, 16.1, 23.1, 7.1, 11.1, 3.1, 16.1, 7.1, 4.1, 8.1, 10.1, 10.1, 5.1, 7.1, 5.1, 3.1, 5.1, 3.1, 4.1, 4.1, 7.1, 7.1, 4.1, 5.1, 2.1, 2.1, 6.1, 3.1, 5.1, 6.1, 4.1, 2.1, 4.1, 5.1, 4.1, 4.1, -0.8999999999999999, 3.1, 4.1, 3.1, 5.1, 3.1, 0.10000000000000009, 7.1, 1.1, 2.1, 3.1, 1.1, 1.1, 4.1, -0.8999999999999999, -0.8999999999999999, 3.1, 0.10000000000000009, 0.10000000000000009, 2.1, 3.1, 1.1, 1.1, 1.1, 0.10000000000000009, 2.1, 4.1, 2.1, 1.1, 4.1, 1.1, 0.10000000000000009, 2.1, -0.8999999999999999, 4.1, -0.8999999999999999, 4.1, 0.10000000000000009, 2.1, 1.1, 1.1, 1.1, 2.1, 0.10000000000000009, -0.8999999999999999, 1.1, 3.1, 1.1, -0.8999999999999999, 1.1, 3.1, 0.10000000000000009, 1.1, 0.10000000000000009, 2.1, 2.1, 1.1, 0.10000000000000009, -0.8999999999999999, -0.8999999999999999, 1.1, -0.8999999999999999, -0.8999999999999999, 0.10000000000000009, -0.8999999999999999, -1.9, -1.9, 1.1, 0.10000000000000009, 1.1, 0.10000000000000009, -0.8999999999999999, 4.1, -0.8999999999999999, 1.1, 0.10000000000000009, -0.8999999999999999, 3.1, 0.10000000000000009, 1.1, 4.1, -1.9, -0.8999999999999999, 0.10000000000000009, -1.9, -0.8999999999999999, 0.10000000000000009, 0.10000000000000009, -1.9, -0.8999999999999999, -0.8999999999999999, -1.9, -0.8999999999999999, 0.10000000000000009, -1.9, -1.9, 0.10000000000000009, 2.1, -0.8999999999999999, -0.8999999999999999, -1.9, -0.8999999999999999, -0.8999999999999999, -1.9, 0.10000000000000009, -1.9, -0.8999999999999999, -0.8999999999999999, 0.10000000000000009, 0.10000000000000009, -0.8999999999999999, -1.9, -0.8999999999999999, -1.9, 0.10000000000000009, -1.9, -0.8999999999999999, 0.10000000000000009, -0.8999999999999999, -1.9, -0.8999999999999999, -0.8999999999999999, -0.8999999999999999, 1.1, 1.1, 0.10000000000000009, 1.1, -0.8999999999999999, -0.8999999999999999, 0.10000000000000009, 0.10000000000000009, -1.9, 1.1, 0.10000000000000009, 0.0]] caption="Water Vapor Number Density"
  out "raw counts near":dbl[][](graph)=[[18593.2, 18818.2, 12421.2, 94.2, 101.2, 173.2, 229.2, 257.2, 290.2, 347.2, 331.2, 348.2, 331.2, 330.2, 316.2, 327.2, 321.2, 310.2, 272.2, 279.2, 230.2, 216.2, 216.2, 158.2, 152.2, 184.2, 151.2, 139.2, 144.2, 124.2, 98.2, 113.2, 80.2, 87.2, 67.2, 85.2, 78.2, 68.2, 75.2, 67.2, 53.2, 82.2, 36.2, 50.2, 49.2, 34.2, 46.2, 51.2, 32.2, 39.2, 45.2, 46.2, 38.2, 28.2, 18.2, 31.2, 20.2, 21.2, 24.2, 22.2, 14.2, 28.2, 26.2, 14.2, 13.2, 18.2, 15.2, 20.2, 15.2, 14.2, 19.2, 14.2, 21.2, 13.2, 18.2, 12.2, 11.2, 18.2, 9.2, 13.2, 10.2, 10.2, 11.2, 11.2, 8.2, 8.2, 17.2, 13.2, 8.2, 3.2, 1.2, 7.2, 7.2, 6.2, 5.2, 10.2, 3.2, 6.2, 4.2, 6.2, 1.2, 2.2, 6.2, 2.2, 2.2, 5.2, 9.2, 3.2, 8.2, 6.2, 9.2, 4.2, 3.2, 1.2, 3.2, 8.2, 4.2, 2.2, 4.2, 3.2, 3.2, 1.2, 3.2, 2.2, 8.2, 1.2, 4.2, 3.2, -0.8, 3.2, 3.2, 6.2, 1.2, 2.2, -0.8, 1.2, 3.2, 2.2, 1.2, -0.8, 5.2, 2.2, 2.2, 0.19999999999999996, -1.8, -0.8, 2.2, 1.2, 2.2, 3.2, 1.2, 2.2, 2.2, 2.2, 1.2, 0.19999999999999996, 4.2, 0.19999999999999996, 0.19999999999999996, 1.2, 1.2, 0.19999999999999996, 1.2, 1.2, 0.19999999999999996, 3.2, -1.8, 0.19999999999999996, 0.19999999999999996, -0.8, 0.19999999999999996, -1.8, -0.8, 2.2, 0.19999999999999996, 0.19999999999999996, 0.19999999999999996, 0.19999999999999996, -0.8, 4.2, -0.8, 0.19999999999999996, -0.8, 1.2, 2.2, -1.8, -0.8, -0.8, 0.19999999999999996, 1.2, -0.8, 1.2, 2.2, -0.8, -1.8, 1.2, -0.8, 0.19999999999999996, 0.19999999999999996, -1.8, 0.19999999999999996, 0.19999999999999996, 0.19999999999999996, 1.2, -0.8, 1.2, 0.19999999999999996, 0.19999999999999996, 2.2, -1.8, 0.19999999999999996, -1.8, 0.19999999999999996, -1.8, -0.8, 0.19999999999999996, 1.2, -0.8, 1.2, 0.19999999999999996, 1.2, 0.19999999999999996, 1.2, -1.8, -1.8, -0.8, -0.8, 1.2, 1.2, 0.19999999999999996, -1.8, -0.8, -1.8, -0.8, -0.8, -1.8, 1.2, 1.2, 0.19999999999999996, -1.8, -0.8, -0.8, 0.19999999999999996, -1.8, -0.8, -0.8, -0.8, -1.8, -0.8, -0.8, -0.8, 0.19999999999999996, 0.19999999999999996, -0.8, 3.2, -0.8, -0.8, -1.8, 0.19999999999999996, -1.8, -1.8, -0.8, -0.8, -0.8, -0.8, 0.19999999999999996, 1.2, -1.8, -1.8, 0.19999999999999996, 2.2, 1.2, -1.8, 0.19999999999999996, 0.19999999999999996, -1.8, 0.19999999999999996, 0.19999999999999996, -0.8, 0.0]] caption="Water Vapor Number Density"
  out "Aerosol Smoothed 2":dbl[](array[numeric])=[18380.284615384615, 15936.63076923077, 6790.323076923078, 146.3230769230769, 247.55384615384617, 381.5153846153846, 504.28461538461534, 581.4384615384615, 618.1307692307693, 629.5538461538463, 635.4384615384615, 632.1307692307693, 608.6307692307693, 585.5153846153846, 552.5153846153846, 516.7461538461539, 481.36153846153843, 444.9384615384615, 411.0923076923077, 378.0923076923077, 340.9384615384615, 306.66923076923075, 278.74615384615385, 254.97692307692307, 237.97692307692307, 221.7076923076923, 201.8230769230769, 186.55384615384617, 174.47692307692307, 160.8230769230769, 146.59230769230768, 132.43846153846152, 122.24615384615385, 111.59230769230768, 106.05384615384617, 101.28461538461539, 94.20769230769231, 87.9, 81.09230769230768, 76.74615384615385, 73.13076923076923, 69.78461538461538, 66.51538461538462, 64.09230769230768, 62.63076923076923, 58.70769230769231, 54.20769230769231, 53.13076923076923, 50.13076923076923, 46.16923076923077, 46.284615384615385, 48.246153846153845, 45.01538461538462, 39.51538461538462, 37.09230769230769, 35.05384615384615, 33.13076923076923, 32.4, 30.899999999999995, 27.015384615384612, 25.130769230769232, 24.746153846153845, 22.553846153846152, 21.207692307692305, 22.399999999999995, 22.976923076923075, 23.361538461538462, 32.47692307692307, 44.169230769230765, 38.55384615384615, 28.092307692307685, 27.4, 28.092307692307692, 27.823076923076922, 28.015384615384612, 28.24615384615384, 27.207692307692305, 25.9, 25.438461538461535, 21.70769230769231, 18.47692307692308, 17.43846153846154, 14.823076923076924, 12.899999999999999, 11.092307692307692, 10.515384615384615, 11.169230769230769, 10.476923076923075, 9.284615384615384, 8.399999999999999, 8.592307692307692, 8.130769230769232, 8.938461538461539, 9.515384615384615, 9.16923076923077, 8.93846153846154, 8.361538461538462, 8.9, 8.592307692307692, 7.707692307692307, 7.515384615384614, 7.976923076923077, 6.784615384615385, 5.323076923076924, 5.976923076923077, 7.438461538461539, 6.515384615384615, 5.207692307692307, 5.476923076923077, 6.0538461538461545, 6.4, 5.246153846153846, 4.823076923076923, 5.207692307692308, 5.053846153846154, 4.4, 4.43846153846154, 5.092307692307694, 4.63076923076923, 4.13076923076923, 3.8999999999999995, 4.053846153846154, 3.4384615384615382, 3.092307692307692, 3.6307692307692303, 3.4769230769230766, 3.938461538461538, 3.861538461538461, 3.1692307692307686, 3.5153846153846153, 3.7846153846153845, 3.5153846153846153, 3.5153846153846153, 3.476923076923077, 3.0153846153846158, 2.6692307692307695, 2.9000000000000004, 2.476923076923077, 1.9384615384615382, 2.4769230769230766, 2.7076923076923074, 2.592307692307692, 2.592307692307692, 2.0153846153846153, 1.7076923076923078, 2.130769230769231, 2.0923076923076924, 1.9, 2.092307692307693, 2.4384615384615387, 2.1307692307692307, 1.7076923076923078, 2.0538461538461537, 1.9, 1.476923076923077, 1.7846153846153845, 1.9384615384615385, 1.2461538461538462, 1.4384615384615382, 1.7846153846153845, 1.9384615384615382, 1.746153846153846, 1.5538461538461539, 1.7076923076923076, 1.746153846153846, 1.4384615384615382, 1.0538461538461539, 1.0153846153846153, 1.0538461538461539, 1.4384615384615382, 1.2846153846153845, 0.7846153846153845, 1.1692307692307693, 1.3615384615384616, 0.5538461538461538, 0.5923076923076922, 0.976923076923077, 0.976923076923077, 1.1307692307692307, 1.1307692307692307, 0.4384615384615385, 0.7076923076923076, 1.4384615384615382, 1.323076923076923, 0.4769230769230769, 0.2846153846153846, 0.9384615384615386, 0.7076923076923077, 0.9384615384615383, 1.0923076923076922, 0.6307692307692307, 0.6692307692307693, 0.7461538461538462, 0.823076923076923, 0.7076923076923078, 0.6307692307692307, 0.5538461538461539, 0.20769230769230768, -0.09999999999999998, 0.24615384615384622, 0.9000000000000001, 0.9000000000000001, 0.6692307692307693, 0.43846153846153846, 0.09230769230769231, 0.2846153846153846, 0.5153846153846153, 0.7846153846153846, 0.5538461538461538, 0.09230769230769224, 0.5538461538461539, 0.8615384615384616, 0.36153846153846153, 0.1307692307692308, 0.2461538461538462, 0.2076923076923077, 0.3230769230769231, 0.4, 0.6692307692307693, 0.5153846153846154, 0.5153846153846153, 0.43846153846153846, 0.16923076923076924, 0.16923076923076924, 0.20769230769230768, 0.13076923076923075, 0.3230769230769231, 0.4, 0.015384615384615365, 0.13076923076923067, 0.16923076923076913, -0.25384615384615383, -0.40769230769230763, -0.3307692307692307, -0.09999999999999994, 0.5923076923076924, 0.476923076923077, -0.1769230769230769, -0.13846153846153844, -0.02307692307692308, 0.0153846153846154, 0.4384615384615385, 0.2461538461538462, -0.023076923076923078, 0.3230769230769231, 0.24615384615384617, 0.24615384615384617, 0.28461538461538466, -0.0615384615384615, -0.023076923076923037, 0.5153846153846154, 0.7461538461538462, 0.5538461538461539, 0.7076923076923076, 0.5153846153846153, 0.13076923076923078, 0.20769230769230768, 0.3615384615384615, 0.36153846153846153, -0.09999999999999994, -0.5615384615384614, -0.523076923076923, -0.3307692307692308, 0.01538461538461533, -0.09999999999999995, -0.13846153846153836, 0.20769230769230773, 0.3230769230769231, 0.24615384615384617, 0.053846153846153835, 0.015384615384615372, -0.061538461538461556, -0.10000000000000002, -0.023076923076923134, -0.176923076923077, -0.2538461538461539, -0.023076923076923096]
  out "Off-Line Smoothed 2":dbl[](array[numeric])=[18288.89480286739, 15820.930645161294, 6707.0964157706085, 155.50053763440863, 299.60089605734765, 504.3580645161288, 636.4073476702506, 671.3777777777775, 671.6080645161288, 656.5820788530464, 635.1896057347668, 608.5372759856627, 576.9897849462362, 542.4826164874551, 504.20752688172036, 464.1627240143368, 424.314157706093, 385.86702508960553, 349.08476702508943, 314.6340501792113, 283.4646953405017, 255.64121863799278, 231.6940860215053, 211.74605734767022, 193.63315412186375, 177.38494623655913, 163.11523297491044, 149.80340501792125, 138.11164874551977, 126.87867383512551, 116.37688172043018, 107.43333333333338, 99.1376344086022, 91.4387096774194, 84.60627240143374, 78.82670250896061, 74.21827956989249, 70.18691756272402, 66.14659498207885, 62.40645161290324, 59.47455197132617, 56.75860215053764, 53.82580645161291, 51.121505376344096, 48.589247311827975, 46.07491039426523, 43.9853046594982, 42.03727598566307, 40.34283154121863, 39.03727598566307, 38.38405017921146, 37.698566308243706, 35.962903225806436, 33.416308243727585, 30.718279569892456, 27.982616487455186, 25.71200716845877, 24.49874551971325, 23.537275985663072, 22.410035842293897, 21.224551971326157, 19.919892473118267, 19.16272401433691, 18.636738351254476, 18.38046594982078, 18.70304659498207, 19.202150537634402, 21.52562724014336, 23.49605734767024, 22.438709677419347, 21.003225806451606, 20.88405017921146, 20.892114695340496, 20.643906810035837, 20.715591397849455, 20.40645161290322, 19.318637992831533, 17.856272401433685, 16.180645161290315, 14.540860215053758, 13.016666666666666, 11.821326164874549, 11.042652329749103, 10.27921146953405, 9.686917562724016, 9.308781362007172, 8.83476702508961, 8.26308243727599, 7.72813620071685, 7.396594982078856, 7.283691756272404, 7.054301075268819, 6.856272401433695, 6.804301075268821, 6.578494623655917, 6.364336917562727, 6.145698924731185, 6.018458781362009, 6.041756272401435, 6.017562724014338, 6.186917562724016, 6.348207885304662, 5.8974910394265265, 5.299820788530468, 5.194086021505379, 5.158243727598569, 4.878673835125451, 4.7505376344086025, 4.84820788530466, 5.211111111111112, 5.307885304659498, 4.594623655913979, 4.058781362007169, 3.9387096774193555, 3.9333333333333345, 3.8204301075268816, 3.5847670250896053, 3.496953405017921, 3.3849462365591396, 3.3939068100358423, 3.3374551971326163, 3.1358422939068107, 3.0802867383512553, 2.9853046594982082, 2.8428315412186382, 2.811469534050179, 2.749641577060932, 2.7200716845878135, 2.7236559139784946, 2.6492831541218633, 2.5740143369175623, 2.5551971326164864, 2.4512544802867375, 2.38853046594982, 2.4440860215053757, 2.2989247311827947, 2.2568100358422933, 2.214695340501791, 2.1170250896057343, 2.1591397849462357, 2.0892473118279566, 2.069534050179211, 2.0068100358422933, 1.8383512544802856, 1.7594982078853039, 1.7155913978494617, 1.6654121863799276, 1.724551971326164, 1.7335125448028665, 1.620609318996415, 1.60358422939068, 1.5417562724014329, 1.5139784946236552, 1.5292114695340495, 1.445878136200716, 1.373297491039426, 1.384050179211469, 1.3643369175627236, 1.3249103942652325, 1.246953405017921, 1.2039426523297487, 1.1672043010752684, 1.0838709677419354, 1.1026881720430108, 1.0829749103942654, 1.0811827956989244, 1.0775985663082432, 1.0094982078853045, 0.953942652329749, 1.0094982078853043, 0.9548387096774192, 0.8741935483870968, 0.9225806451612903, 0.88584229390681, 0.8930107526881721, 0.8356630824372759, 0.7406810035842292, 0.7559139784946235, 0.7872759856630824, 0.8661290322580644, 0.8034050179211469, 0.6985663082437277, 0.6869175627240146, 0.6761648745519715, 0.6967741935483869, 0.6645161290322577, 0.6663082437275984, 0.721863799283154, 0.7173835125448027, 0.6528673835125449, 0.6035842293906812, 0.5901433691756274, 0.5892473118279572, 0.5919354838709681, 0.5623655913978497, 0.5560931899641579, 0.4942652329749106, 0.5121863799283156, 0.5112903225806453, 0.4637992831541221, 0.47186379928315436, 0.4225806451612905, 0.399283154121864, 0.38942652329749117, 0.4494623655913982, 0.4315412186379932, 0.381362007168459, 0.40017921146953417, 0.4252688172043012, 0.44587813620071703, 0.4118279569892474, 0.3401433691756274, 0.3168458781362009, 0.31057347670250907, 0.2657706093189965, 0.25949820788530475, 0.2827956989247313, 0.28010752688172047, 0.3051971326164875, 0.3051971326164875, 0.31415770609319005, 0.3616487455197135, 0.3724014336917565, 0.33297491039426536, 0.24426523297491046, 0.2218637992831542, 0.256810035842294, 0.2514336917562725, 0.224551971326165, 0.24964157706093199, 0.23620071684587812, 0.19677419354838707, 0.1546594982078853, 0.14928315412186383, 0.22634408602150546, 0.19856630824372762, 0.20931899641577068, 0.23351254480286754, 0.15555555555555556, 0.12508960573476696, 0.1421146953405018, 0.13046594982078852, 0.11164874551971327, 0.12508960573476702, 0.14390681003584227, 0.12598566308243725, 0.121505376344086, 0.11881720430107523, 0.07759856630824374, 0.0668458781362007, 0.09641577060931894, 0.08476702508960574, 0.08207885304659497, 0.1250896057347669, 0.09551971326164868, 0.11344086021505377, 0.12598566308243728, 0.10896057347670249, 0.08655913978494621, 0.01666666666666667, -0.0200716845878136, -0.022759856630824356, -0.02455197132616489, 0.011290322580645143, 0.06505376344086018, 0.03817204301075268, -0.0290322580645161, -0.042473118279569885, -0.010215053763440887, 0.038172043010752665, 0.04086021505376346, 0.028315412186379955, -0.016487455197132597, -0.0586021505376344, -0.02813620071684588, -0.007526881720430098, 0.011290322580645187]
  out "Off-Line Bin Readings 2":dbl[](array[numeric])=[18595.0, 18820.0, 12423.0, 96.0, 103.0, 175.0, 231.0, 259.0, 292.0, 349.0, 333.0, 350.0, 333.0, 332.0, 318.0, 329.0, 323.0, 312.0, 274.0, 281.0, 232.0, 218.0, 218.0, 160.0, 154.0, 186.0, 153.0, 141.0, 146.0, 126.0, 100.0, 115.0, 82.0, 89.0, 69.0, 87.0, 80.0, 70.0, 77.0, 69.0, 55.0, 84.0, 38.0, 52.0, 51.0, 36.0, 48.0, 53.0, 34.0, 41.0, 47.0, 48.0, 40.0, 30.0, 20.0, 33.0, 22.0, 23.0, 26.0, 24.0, 16.0, 30.0, 28.0, 16.0, 15.0, 20.0, 17.0, 22.0, 17.0, 16.0, 21.0, 16.0, 23.0, 15.0, 20.0, 14.0, 13.0, 20.0, 11.0, 15.0, 12.0, 12.0, 13.0, 13.0, 10.0, 10.0, 19.0, 15.0, 10.0, 5.0, 3.0, 9.0, 9.0, 8.0, 7.0, 12.0, 5.0, 8.0, 6.0, 8.0, 3.0, 4.0, 8.0, 4.0, 4.0, 7.0, 11.0, 5.0, 10.0, 8.0, 11.0, 6.0, 5.0, 3.0, 5.0, 10.0, 6.0, 4.0, 6.0, 5.0, 5.0, 3.0, 5.0, 4.0, 10.0, 3.0, 6.0, 5.0, 1.0, 5.0, 5.0, 8.0, 3.0, 4.0, 1.0, 3.0, 5.0, 4.0, 3.0, 1.0, 7.0, 4.0, 4.0, 2.0, 0.0, 1.0, 4.0, 3.0, 4.0, 5.0, 3.0, 4.0, 4.0, 4.0, 3.0, 2.0, 6.0, 2.0, 2.0, 3.0, 3.0, 2.0, 3.0, 3.0, 2.0, 5.0, 0.0, 2.0, 2.0, 1.0, 2.0, 0.0, 1.0, 4.0, 2.0, 2.0, 2.0, 2.0, 1.0, 6.0, 1.0, 2.0, 1.0, 3.0, 4.0, 0.0, 1.0, 1.0, 2.0, 3.0, 1.0, 3.0, 4.0, 1.0, 0.0, 3.0, 1.0, 2.0, 2.0, 0.0, 2.0, 2.0, 2.0, 3.0, 1.0, 3.0, 2.0, 2.0, 4.0, 0.0, 2.0, 0.0, 2.0, 0.0, 1.0, 2.0, 3.0, 1.0, 3.0, 2.0, 3.0, 2.0, 3.0, 0.0, 0.0, 1.0, 1.0, 3.0, 3.0, 2.0, 0.0, 1.0, 0.0, 1.0, 1.0, 0.0, 3.0, 3.0, 2.0, 0.0, 1.0, 1.0, 2.0, 0.0, 1.0, 1.0, 1.0, 0.0, 1.0, 1.0, 1.0, 2.0, 2.0, 1.0, 5.0, 1.0, 1.0, 0.0, 2.0, 0.0, 0.0, 1.0, 1.0, 1.0, 1.0, 2.0, 3.0, 0.0, 0.0, 2.0, 4.0, 3.0, 0.0, 2.0, 2.0, 0.0, 2.0, 2.0, 1.0]
  out "On-Line Smoothed 2":dbl[](array[numeric])=[17613.06218637991, 15906.821146953394, 6734.596236559142, 156.22168458781346, 289.0962365591401, 470.7252688172051, 573.5845878136209, 583.5684587813628, 568.848028673836, 547.0021505376354, 521.0218637992841, 492.68942652329827, 461.8507168458788, 426.26379928315475, 388.7584229390686, 352.2154121863805, 315.82293906810094, 281.8426523297494, 250.87132616487457, 223.13476702508947, 199.41881720430095, 177.70376344086006, 158.39283154121844, 143.6643369175625, 130.70555555555535, 118.79426523297474, 108.51827956989233, 98.77992831541206, 90.1885304659497, 82.33189964157691, 75.18584229390669, 69.10878136200711, 63.27365591397849, 57.98960573476704, 53.59534050179214, 49.58369175627243, 46.21810035842297, 43.740501792114735, 40.79784946236565, 37.93763440860221, 35.79068100358429, 33.85161290322586, 32.29964157706098, 30.335483870967785, 28.68584229390685, 27.207347670250932, 25.485125448028707, 24.04336917562727, 22.932258064516155, 22.078315412186413, 21.249462365591434, 20.69659498207889, 20.02544802867387, 18.385663082437304, 16.51648745519714, 14.975268817204302, 13.752150537634405, 12.91702508960573, 12.220788530465944, 11.683154121863794, 11.134767025089598, 10.458243727598555, 9.76379928315411, 9.363261648745507, 9.37939068100357, 9.502150537634396, 9.70107526881719, 10.61505376344085, 11.262903225806443, 10.729749103942641, 10.085483870967728, 9.925089605734755, 10.028136200716833, 10.065770609318983, 9.963620071684574, 9.705555555555542, 9.156272401433675, 8.331003584229375, 7.658064516129019, 7.0057347670250785, 6.280824372759849, 5.858781362007161, 5.498566308243719, 5.267383512544793, 4.873118279569885, 4.464516129032253, 4.343548387096771, 4.103405017921146, 3.819354838709678, 3.6679211469534065, 3.5872759856630845, 3.5684587813620094, 3.456451612903227, 3.2655913978494637, 3.218100358422941, 3.2270609318996435, 3.2118279569892487, 3.1517921146953425, 3.0711469534050195, 2.8784946236559157, 2.9609318996415794, 3.206451612903228, 2.980645161290325, 2.652688172043013, 2.5845878136200744, 2.5899641577060963, 2.52903225806452, 2.367741935483875, 2.3175627240143415, 2.5675627240143406, 2.6168458781362043, 2.290681003584233, 2.026344086021509, 1.9286738351254513, 1.8847670250896087, 1.910752688172046, 1.8955197132616517, 1.794265232974913, 1.7691756272401458, 1.8059139784946263, 1.7637992831541243, 1.6222222222222247, 1.588172043010755, 1.608781362007171, 1.616845878136203, 1.5191756272401453, 1.5048387096774214, 1.4842293906810058, 1.3820788530465968, 1.42867383512545, 1.4188172043010772, 1.2933691756272419, 1.2279569892473137, 1.267383512544805, 1.203763440860217, 1.1302867383512556, 1.1025089605734777, 1.0881720430107538, 1.0559139784946243, 1.0505376344086028, 1.1607526881720445, 1.1007168458781371, 1.027240143369176, 1.0379928315412192, 1.0442652329749111, 1.0845878136200728, 0.9743727598566314, 0.9008960573476701, 0.8811827956989244, 0.858781362007168, 0.8910394265232973, 0.8775985663082435, 0.8202508960573472, 0.8292114695340498, 0.843548387096774, 0.7951612903225802, 0.776344086021505, 0.7413978494623652, 0.7342293906810031, 0.7494623655913972, 0.7351254480286733, 0.7431899641577058, 0.7091397849462362, 0.6455197132616479, 0.6159498207885296, 0.620430107526881, 0.6464157706093183, 0.6607526881720422, 0.6768817204301067, 0.6186379928315404, 0.5684587813620063, 0.5836917562724004, 0.5612903225806442, 0.5478494623655905, 0.5863799283154112, 0.5971326164874542, 0.58189964157706, 0.5827956989247303, 0.553225806451612, 0.5290322580645154, 0.5048387096774185, 0.47078853046594915, 0.5075268817204295, 0.49946236559139723, 0.46720430107526834, 0.469892473118279, 0.38745519713261595, 0.3605734767025084, 0.43315412186379854, 0.4582437275985656, 0.4035842293906804, 0.36505376344085966, 0.33637992831541164, 0.2996415770609314, 0.3345878136200713, 0.3650537634408597, 0.3372759856630818, 0.3435483870967736, 0.3874551971326159, 0.3767025089605729, 0.33010752688171996, 0.3256272401433687, 0.31935483870967696, 0.32114695340501753, 0.29247311827956957, 0.2584229390681001, 0.26559139784946206, 0.26648745519713235, 0.2951612903225803, 0.29874551971326113, 0.2557347670250894, 0.25035842293906807, 0.23602150537634403, 0.21810035842293912, 0.22168458781362016, 0.21541218637992843, 0.21899641577060933, 0.28888888888888853, 0.2853046594982076, 0.20197132616487462, 0.1813620071684589, 0.20017921146953416, 0.2575268817204298, 0.251254480286738, 0.23064516129032253, 0.17150537634408605, 0.16344086021505383, 0.19569892473118294, 0.22437275985663063, 0.27544802867383483, 0.22258064516129036, 0.1526881720430109, 0.18225806451612914, 0.21003584229390687, 0.1553763440860216, 0.10878136200716856, 0.08458781362007174, 0.10071684587813631, 0.071146953405018, 0.09623655913978499, 0.11236559139784949, 0.08906810035842302, 0.16612903225806466, 0.14731182795698938, 0.13476702508960592, 0.09892473118279578, 0.051433691756272465, 0.10250896057347689, 0.08817204301075277, 0.06666666666666671, 0.11505376344086041, 0.1168458781362009, 0.06129032258064518, 0.020071684587813596, 0.037096774193548426, 0.07293906810035847, 0.0917562724014338, 0.10698924731182813, 0.09982078853046608, 0.08279569892473136, 0.04516129032258073, 0.06487455197132623, 0.06308243727598573, 0.019175627240143357, 0.0541218637992832, 0.06845878136200723, 0.0666666666666667, 0.09444444444444454, 0.01827956989247318, -0.005017921146953416, 0.02544802867383512, -0.008602150537634416, -0.013082437275985688, 0.021863799283154125, 0.07204301075268821, 0.03082437275985666, -0.06326164874551964]
  out "On-Line Bin Readings 2":dbl[](array[numeric])=[15808.0, 18262.0, 12448.0, 96.0, 95.0, 163.0, 203.0, 242.0, 237.0, 253.0, 245.0, 290.0, 289.0, 244.0, 237.0, 234.0, 227.0, 201.0, 197.0, 176.0, 158.0, 164.0, 155.0, 151.0, 114.0, 94.0, 84.0, 95.0, 76.0, 100.0, 51.0, 68.0, 60.0, 59.0, 46.0, 48.0, 46.0, 32.0, 37.0, 38.0, 32.0, 29.0, 28.0, 36.0, 32.0, 27.0, 33.0, 24.0, 25.0, 25.0, 25.0, 22.0, 16.0, 16.0, 12.0, 16.0, 22.0, 14.0, 18.0, 12.0, 19.0, 8.0, 8.0, 9.0, 12.0, 11.0, 5.0, 10.0, 11.0, 12.0, 11.0, 8.0, 6.0, 8.0, 10.0, 7.0, 9.0, 7.0, 10.0, 7.0, 6.0, 11.0, 5.0, 6.0, 4.0, 4.0, 5.0, 6.0, 6.0, 8.0, 4.0, 6.0, 4.0, 4.0, 3.0, 3.0, 3.0, 3.0, 6.0, 4.0, 2.0, 4.0, 3.0, 2.0, 3.0, 5.0, 1.0, 4.0, 2.0, 4.0, 10.0, 4.0, 7.0, 6.0, 1.0, 5.0, 2.0, 1.0, 2.0, 2.0, 6.0, 3.0, 7.0, 2.0, 8.0, 2.0, 3.0, 2.0, 5.0, 0.0, 0.0, 3.0, 3.0, 1.0, 2.0, 3.0, 2.0, 3.0, 0.0, 4.0, 4.0, 1.0, 0.0, 3.0, 1.0, 2.0, 7.0, 0.0, 4.0, 1.0, 5.0, 4.0, 1.0, 2.0, 2.0, 0.0, 1.0, 2.0, 2.0, 0.0, 2.0, 2.0, 3.0, 0.0, 3.0, 2.0, 1.0, 2.0, 4.0, 1.0, 1.0, 3.0, 2.0, 0.0, 1.0, 3.0, 3.0, 2.0, 1.0, 2.0, 3.0, 2.0, 3.0, 2.0, 3.0, 1.0, 1.0, 0.0, 3.0, 2.0, 1.0, 1.0, 1.0, 0.0, 3.0, 0.0, 0.0, 1.0, 2.0, 2.0, 1.0, 0.0, 3.0, 1.0, 2.0, 3.0, 2.0, 0.0, 2.0, 2.0, 3.0, 3.0, 1.0, 0.0, 1.0, 0.0, 4.0, 2.0, 1.0, 1.0, 2.0, 2.0, 1.0, 0.0, 2.0, 3.0, 0.0, 2.0, 3.0, 0.0, 2.0, 1.0, 0.0, 2.0, 3.0, 2.0, 2.0, 0.0, 1.0, 1.0, 0.0, 2.0, 3.0, 0.0, 0.0, 4.0, 0.0, 3.0, 2.0, 1.0, 0.0, 1.0, 2.0, 2.0, 4.0, 3.0, 1.0, 3.0, 1.0, 2.0, 2.0, 2.0, 1.0, 0.0, 4.0, 4.0, 1.0, 1.0, 0.0, 2.0, 1.0, 0.0, 2.0, 1.0, 2.0, 2.0, 1.0, 0.0, 1.0]
  in  "stop":bool
  in  "Reset Average":bool=TRUE
  in  "Save Data?":bool=TRUE
  in  "Collect Data?":bool=TRUE
  in  "ILX Address":i32=6 min=0 step=1
  in  "Lambda On DBR Current":dbl=158.08
  in  "Lambda Off DBR Current":dbl=160.0
  in  "Tab Control":T2(tab)=enum."OD"
  out "Water Vapor Number Density  2":cluster{"Y":dbl[], "Y":dbl[]}[](graph)
  out "Absolute Humidity":cluster{"Y":dbl[], "Y":dbl[]}[](graph)
  out "NRB plot":cluster{"Y":dbl[], "Y":dbl[]}[](graph)
  in  "background length":i32=10
  out "Correction":cluster{"Y":dbl[], "Y":dbl[]}[](graph)
  in  "dead time":dbl=3.7e-08
  out "Optical Depth":cluster{"Y":dbl[], "Y":dbl[]}[](graph) caption="XY Graph"
  out "RingBuffer offline far":dbl[][](array[numeric])
  out "RingBuffer aerosol far":dbl[][](array[numeric])=[[16071.7, 17535.7, 11503.7, 53.7, 66.7, 93.7, 98.7, 104.7, 103.7, 121.7, 159.7, 155.7, 219.7, 219.7, 229.7, 247.7, 251.7, 229.7, 261.7, 287.7, 312.7, 321.7, 328.7, 329.7, 307.7, 312.7, 311.7, 271.7, 298.7, 262.7, 272.7, 240.7, 230.7, 225.7, 209.7, 205.7, 180.7, 177.7, 179.7, 156.7, 146.7, 140.7, 137.7, 118.7, 128.7, 111.7, 123.7, 109.7, 107.7, 114.7, 96.7, 109.7, 97.7, 100.7, 77.7, 74.7, 64.7, 54.7, 76.7, 49.7, 46.7, 46.7, 59.7, 47.7, 55.7, 30.7, 34.7, 35.7, 43.7, 50.7, 45.7, 53.7, 42.7, 42.7, 55.7, 50.7, 40.7, 45.7, 30.7, 32.7, 23.7, 27.7, 24.7, 25.7, 20.7, 25.7, 15.7, 17.7, 17.7, 17.7, 12.7, 15.7, 18.7, 11.7, 17.7, 8.7, 5.7, 13.7, 10.7, 13.7, 10.7, 6.7, 8.7, 11.7, 7.7, 20.7, 19.7, 8.7, 7.7, 10.7, 28.7, 20.7, 11.7, 11.7, 1.7, 9.7, 6.7, 12.7, 3.7, 8.7, 9.7, 13.7, 6.7, 5.7, 8.7, 2.7, 8.7, 5.7, 10.7, 3.7, 3.7, 4.7, 6.7, 5.7, 3.7, 1.7, 3.7, 8.7, 0.7, 1.7, 4.7, 8.7, 3.7, 3.7, 2.7, 5.7, 4.7, 0.7, 2.7, 2.7, 0.7, 2.7, 3.7, 4.7, -0.30000000000000004, 1.7, 1.7, 3.7, 0.7, 1.7, 1.7, 2.7, -0.30000000000000004, 1.7, 0.7, -0.30000000000000004, 1.7, -0.30000000000000004, 1.7, 4.7, 0.7, -0.30000000000000004, 2.7, 0.7, -1.3, -0.30000000000000004, 1.7, 0.7, 2.7, 3.7, 1.7, -0.30000000000000004, 1.7, 2.7, 4.7, 0.7, 0.7, -0.30000000000000004, 0.7, 2.7, -0.30000000000000004, 1.7, 1.7, -0.30000000000000004, 0.7, 1.7, 1.7, 2.7, -0.30000000000000004, 0.7, 4.7, 0.7, -0.30000000000000004, 0.7, 1.7, 1.7, -0.30000000000000004, 1.7, -0.30000000000000004, -1.3, 0.7, 2.7, -1.3, 3.7, -0.30000000000000004, -0.30000000000000004, 1.7, -0.30000000000000004, -0.30000000000000004, -0.30000000000000004, -0.30000000000000004, -1.3, -1.3, 1.7, -0.30000000000000004, 0.7, -0.30000000000000004, -1.3, -0.30000000000000004, -0.30000000000000004, -1.3, 1.7, -0.30000000000000004, -0.30000000000000004, 0.7, 0.7, -1.3, -0.30000000000000004, -1.3, -1.3, 0.7, -0.30000000000000004, -1.3, 1.7, 0.7, -0.30000000000000004, -0.30000000000000004, -1.3, -1.3, 1.7, 1.7, -0.30000000000000004, -0.30000000000000004, -0.30000000000000004, -0.30000000000000004, -0.30000000000000004, -0.30000000000000004, -0.30000000000000004, 0.7, -1.3, 0.7, 0.7, -0.30000000000000004, 0.7, 0.7, -0.30000000000000004, 0.7, 3.7, 3.7, -1.3, -1.3, 0.7, 1.7, 0.7, -1.3, 0.7, 0.7, -0.30000000000000004, -0.30000000000000004], [17341.9, 18807.9, 11523.9, 36.9, 59.9, 80.9, 94.9, 87.9, 96.9, 120.9, 166.9, 151.9, 216.9, 198.9, 250.9, 239.9, 275.9, 304.9, 303.9, 262.9, 297.9, 280.9, 296.9, 300.9, 294.9, 283.9, 308.9, 290.9, 272.9, 299.9, 261.9, 224.9, 208.9, 231.9, 193.9, 186.9, 185.9, 161.9, 167.9, 151.9, 158.9, 146.9, 135.9, 119.9, 112.9, 129.9, 99.9, 122.9, 92.9, 91.9, 80.9, 122.9, 96.9, 82.9, 74.9, 69.9, 66.9, 57.9, 65.9, 56.9, 44.9, 48.9, 45.9, 44.9, 44.9, 51.9, 40.9, 47.9, 40.9, 40.9, 37.9, 39.9, 50.9, 46.9, 49.9, 59.9, 27.9, 25.9, 33.9, 39.9, 34.9, 22.9, 34.9, 30.9, 31.9, 18.9, 22.9, 12.9, 19.9, 23.9, 14.9, 16.9, 10.9, 19.9, 11.9, 10.9, 18.9, 18.9, 9.9, 15.9, 8.9, 8.9, 12.9, 12.9, 14.9, 14.9, 22.9, 13.9, 21.9, 12.9, 18.9, 22.9, 3.9, 7.9, 8.9, 13.9, 6.9, 8.9, 7.9, 4.9, 4.9, 8.9, 4.9, 8.9, 2.9, 8.9, 3.9, 0.8999999999999999, 4.9, 4.9, 4.9, 1.9, -0.10000000000000009, 4.9, 5.9, 5.9, 4.9, 3.9, 5.9, 0.8999999999999999, 6.9, 3.9, 0.8999999999999999, 1.9, 3.9, 3.9, 2.9, 1.9, 4.9, 2.9, 6.9, 1.9, 1.9, -0.10000000000000009, 1.9, 1.9, 4.9, 5.9, 0.8999999999999999, 0.8999999999999999, 1.9, 2.9, -0.10000000000000009, 2.9, 2.9, 1.9, 1.9, 4.9, -0.10000000000000009, 0.8999999999999999, 0.8999999999999999, -0.10000000000000009, 1.9, -0.10000000000000009, 0.8999999999999999, 2.9, -0.10000000000000009, 2.9, 3.9, 1.9, 0.8999999999999999, -1.1, 1.9, 1.9, 7.9, 1.9, 4.9, 1.9, 0.8999999999999999, 0.8999999999999999, 0.8999999999999999, -0.10000000000000009, 0.8999999999999999, 0.8999999999999999, 2.9, 1.9, -0.10000000000000009, -1.1, -0.10000000000000009, 0.8999999999999999, -0.10000000000000009, 1.9, -0.10000000000000009, -1.1, 0.8999999999999999, -0.10000000000000009, 2.9, -0.10000000000000009, 0.8999999999999999, -0.10000000000000009, 0.8999999999999999, -1.1, 0.8999999999999999, 0.8999999999999999, 1.9, -0.10000000000000009, -0.10000000000000009, 1.9, 2.9, 0.8999999999999999, -0.10000000000000009, 3.9, -0.10000000000000009, -0.10000000000000009, 0.8999999999999999, -0.10000000000000009, 1.9, -1.1, 1.9, 1.9, 1.9, 1.9, -0.10000000000000009, -0.10000000000000009, -0.10000000000000009, 0.8999999999999999, 0.8999999999999999, -0.10000000000000009, -0.10000000000000009, 1.9, 0.8999999999999999, -0.10000000000000009, 2.9, -1.1, -0.10000000000000009, 0.8999999999999999, -0.10000000000000009, -1.1, -1.1, 0.8999999999999999, 0.8999999999999999, 1.9, 0.8999999999999999, 1.9, -0.10000000000000009, -0.10000000000000009, 1.9, -1.1, -0.10000000000000009, 2.9, -0.10000000000000009, -1.1, 0.8999999999999999, 0.8999999999999999, 0.8999999999999999, 1.9, -0.10000000000000009, -1.1, -0.10000000000000009, 1.9, -0.10000000000000009, -1.1, 0.8999999999999999, -1.1, 0.8999999999999999, -0.10000000000000009, -1.1, -0.10000000000000009, -0.10000000000000009], [16897.1, 18435.1, 11496.1, 29.1, 47.1, 65.1, 95.1, 94.1, 86.1, 128.1, 128.1, 158.1, 205.1, 190.1, 194.1, 234.1, 223.1, 240.1, 268.1, 251.1, 278.1, 273.1, 261.1, 275.1, 277.1, 284.1, 254.1, 225.1, 256.1, 233.1, 238.1, 207.1, 215.1, 208.1, 178.1, 177.1, 185.1, 151.1, 174.1, 159.1, 131.1, 149.1, 135.1, 131.1, 124.1, 114.1, 116.1, 107.1, 113.1, 92.1, 98.1, 85.1, 95.1, 91.1, 75.1, 74.1, 65.1, 61.1, 56.1, 45.1, 53.1, 47.1, 43.1, 40.1, 41.1, 40.1, 47.1, 41.1, 37.1, 59.1, 44.1, 52.1, 56.1, 62.1, 45.1, 30.1, 40.1, 38.1, 39.1, 29.1, 20.1, 29.1, 22.1, 22.1, 26.1, 16.1, 15.1, 19.1, 10.1, 21.1, 21.1, 22.1, 14.1, 15.1, 15.1, 17.1, 14.1, 10.1, 17.1, 13.1, 12.1, 19.1, 5.1, 18.1, 17.1, 18.1, 10.1, 14.1, 15.1, 20.1, 16.1, 23.1, 7.1, 11.1, 3.1, 16.1, 7.1, 4.1, 8.1, 10.1, 10.1, 5.1, 7.1, 5.1, 3.1, 5.1, 3.1, 4.1, 4.1, 7.1, 7.1, 4.1, 5.1, 2.1, 2.1, 6.1, 3.1, 5.1, 6.1, 4.1, 2.1, 4.1, 5.1, 4.1, 4.1, -0.8999999999999999, 3.1, 4.1, 3.1, 5.1, 3.1, 0.10000000000000009, 7.1, 1.1, 2.1, 3.1, 1.1, 1.1, 4.1, -0.8999999999999999, -0.8999999999999999, 3.1, 0.10000000000000009, 0.10000000000000009, 2.1, 3.1, 1.1, 1.1, 1.1, 0.10000000000000009, 2.1, 4.1, 2.1, 1.1, 4.1, 1.1, 0.10000000000000009, 2.1, -0.8999999999999999, 4.1, -0.8999999999999999, 4.1, 0.10000000000000009, 2.1, 1.1, 1.1, 1.1, 2.1, 0.10000000000000009, -0.8999999999999999, 1.1, 3.1, 1.1, -0.8999999999999999, 1.1, 3.1, 0.10000000000000009, 1.1, 0.10000000000000009, 2.1, 2.1, 1.1, 0.10000000000000009, -0.8999999999999999, -0.8999999999999999, 1.1, -0.8999999999999999, -0.8999999999999999, 0.10000000000000009, -0.8999999999999999, -1.9, -1.9, 1.1, 0.10000000000000009, 1.1, 0.10000000000000009, -0.8999999999999999, 4.1, -0.8999999999999999, 1.1, 0.10000000000000009, -0.8999999999999999, 3.1, 0.10000000000000009, 1.1, 4.1, -1.9, -0.8999999999999999, 0.10000000000000009, -1.9, -0.8999999999999999, 0.10000000000000009, 0.10000000000000009, -1.9, -0.8999999999999999, -0.8999999999999999, -1.9, -0.8999999999999999, 0.10000000000000009, -1.9, -1.9, 0.10000000000000009, 2.1, -0.8999999999999999, -0.8999999999999999, -1.9, -0.8999999999999999, -0.8999999999999999, -1.9, 0.10000000000000009, -1.9, -0.8999999999999999, -0.8999999999999999, 0.10000000000000009, 0.10000000000000009, -0.8999999999999999, -1.9, -0.8999999999999999, -1.9, 0.10000000000000009, -1.9, -0.8999999999999999, 0.10000000000000009, -0.8999999999999999, -1.9, -0.8999999999999999, -0.8999999999999999, -0.8999999999999999, 1.1, 1.1, 0.10000000000000009, 1.1, -0.8999999999999999, -0.8999999999999999, 0.10000000000000009, 0.10000000000000009, -1.9, 1.1, 0.10000000000000009], [17272.9, 17907.9, 12394.9, 54.9, 80.9, 108.9, 140.9, 134.9, 147.9, 187.9, 228.9, 248.9, 298.9, 359.9, 375.9, 370.9, 387.9, 391.9, 376.9, 390.9, 379.9, 379.9, 385.9, 378.9, 331.9, 365.9, 404.9, 392.9, 328.9, 355.9, 326.9, 280.9, 247.9, 271.9, 243.9, 229.9, 223.9, 179.9, 195.9, 189.9, 165.9, 158.9, 144.9, 149.9, 166.9, 139.9, 130.9, 119.9, 130.9, 91.9, 109.9, 113.9, 116.9, 129.9, 106.9, 93.9, 104.9, 80.9, 84.9, 71.9, 66.9, 49.9, 74.9, 48.9, 57.9, 57.9, 59.9, 62.9, 55.9, 54.9, 80.9, 74.9, 75.9, 72.9, 70.9, 75.9, 65.9, 59.9, 67.9, 72.9, 47.9, 59.9, 33.9, 32.9, 38.9, 38.9, 22.9, 17.9, 27.9, 13.9, 16.9, 29.9, 16.9, 10.9, 18.9, 16.9, 20.9, 16.9, 15.9, 14.9, 23.9, 19.9, 9.9, 15.9, 8.9, 12.9, 15.9, 16.9, 10.9, 17.9, 7.9, 8.9, 8.9, 10.9, 14.9, 10.9, 12.9, 6.9, 9.9, 22.9, 9.9, 8.9, 9.9, 11.9, 7.9, 2.9, 4.9, 7.9, 5.9, 2.9, 3.9, 8.9, 5.9, 12.9, 5.9, 6.9, 5.9, 4.9, 3.9, 7.9, 7.9, 4.9, 4.9, 8.9, 3.9, 3.9, 10.9, 6.9, 2.9, 5.9, 2.9, -0.10000000000000009, 2.9, 2.9, 3.9, 3.9, 3.9, 2.9, 0.8999999999999999, 1.9, 3.9, 5.9, 5.9, 0.8999999999999999, 2.9, 3.9, 3.9, 5.9, 4.9, 1.9, 4.9, 1.9, 1.9, 1.9, 1.9, 0.8999999999999999, 3.9, -0.10000000000000009, 5.9, 3.9, 2.9, 0.8999999999999999, 2.9, -0.10000000000000009, 3.9, 1.9, 1.9, -0.10000000000000009, 3.9, -0.10000000000000009, 0.8999999999999999, 0.8999999999999999, 4.9, 1.9, -0.10000000000000009, 1.9, -1.1, 0.8999999999999999, 1.9, 0.8999999999999999, 1.9, -1.1, 1.9, -1.1, 0.8999999999999999, -1.1, 0.8999999999999999, -0.10000000000000009, 3.9, -0.10000000000000009, 2.9, 0.8999999999999999, 1.9, -1.1, -0.10000000000000009, 1.9, -0.10000000000000009, 2.9, 2.9, 0.8999999999999999, 0.8999999999999999, 0.8999999999999999, 0.8999999999999999, -0.10000000000000009, -1.1, -0.10000000000000009, -0.10000000000000009, -0.10000000000000009, -0.10000000000000009, -0.10000000000000009, -0.10000000000000009, 2.9, -1.1, 0.8999999999999999, -0.10000000000000009, 2.9, -0.10000000000000009, -0.10000000000000009, 0.8999999999999999, 0.8999999999999999, 0.8999999999999999, 0.8999999999999999, 1.9, -0.10000000000000009, -1.1, -0.10000000000000009, -1.1, -0.10000000000000009, -1.1, 1.9, -1.1, 0.8999999999999999, 2.9, -1.1, 1.9, -0.10000000000000009, -0.10000000000000009, 0.8999999999999999, 1.9, 0.8999999999999999, 1.9, 1.9, -1.1, -1.1, 0.8999999999999999, -1.1, 0.8999999999999999, 0.8999999999999999, -1.1, 0.8999999999999999, -0.10000000000000009, -0.10000000000000009, -1.1, -1.1, -0.10000000000000009, -1.1, 1.9, -0.10000000000000009, 0.8999999999999999], [18227.2, 18929.2, 12599.2, 70.2, 99.2, 143.2, 130.2, 121.2, 140.2, 190.2, 204.2, 267.2, 309.2, 364.2, 355.2, 391.2, 410.2, 419.2, 413.2, 376.2, 400.2, 413.2, 422.2, 384.2, 389.2, 405.2, 391.2, 398.2, 332.2, 389.2, 317.2, 314.2, 300.2, 261.2, 223.2, 214.2, 244.2, 197.2, 209.2, 202.2, 165.2, 190.2, 160.2, 162.2, 146.2, 112.2, 131.2, 112.2, 123.2, 94.2, 117.2, 103.2, 116.2, 124.2, 98.2, 95.2, 90.2, 82.2, 76.2, 80.2, 68.2, 61.2, 48.2, 45.2, 44.2, 63.2, 63.2, 60.2, 72.2, 110.2, 102.2, 67.2, 85.2, 81.2, 71.2, 78.2, 61.2, 71.2, 46.2, 51.2, 56.2, 63.2, 39.2, 48.2, 39.2, 36.2, 25.2, 28.2, 23.2, 19.2, 24.2, 20.2, 19.2, 12.2, 21.2, 15.2, 14.2, 20.2, 15.2, 15.2, 14.2, 14.2, 12.2, 11.2, 11.2, 17.2, 14.2, 16.2, 10.2, 14.2, 13.2, 6.2, 11.2, 2.2, 8.2, 12.2, 6.2, 9.2, 6.2, 3.2, 12.2, 9.2, 15.2, 7.2, 5.2, 9.2, 17.2, 6.2, 5.2, 9.2, 6.2, 10.2, 3.2, 2.2, 6.2, 8.2, 9.2, 6.2, 6.2, 4.2, 6.2, 5.2, 9.2, 6.2, 2.2, 7.2, 9.2, 5.2, 2.2, 1.2, 4.2, 3.2, 1.2, 4.2, 4.2, 3.2, 3.2, 6.2, 7.2, 5.2, 2.2, 5.2, 7.2, 4.2, 3.2, 5.2, 2.2, 3.2, 1.2, 3.2, 5.2, 2.2, 2.2, 1.2, 4.2, 1.2, 1.2, 3.2, 3.2, 1.2, 3.2, 3.2, 4.2, 1.2, 2.2, 3.2, 4.2, 0.19999999999999996, 2.2, 1.2, 0.19999999999999996, 1.2, 5.2, 0.19999999999999996, 5.2, 0.19999999999999996, -0.8, 1.2, 2.2, 3.2, 0.19999999999999996, 1.2, 2.2, 0.19999999999999996, 0.19999999999999996, 3.2, 1.2, 4.2, 1.2, 2.2, 0.19999999999999996, 3.2, 2.2, 0.19999999999999996, 0.19999999999999996, 0.19999999999999996, 0.19999999999999996, 3.2, 1.2, 0.19999999999999996, 1.2, 0.19999999999999996, 1.2, 0.19999999999999996, 0.19999999999999996, 2.2, 5.2, 2.2, 3.2, -0.8, 2.2, 0.19999999999999996, -0.8, -0.8, 0.19999999999999996, 0.19999999999999996, 1.2, 0.19999999999999996, 0.19999999999999996, 0.19999999999999996, 4.2, 1.2, 2.2, 0.19999999999999996, 1.2, 1.2, 3.2, 0.19999999999999996, 0.19999999999999996, -0.8, 0.19999999999999996, -0.8, 0.19999999999999996, -0.8, 0.19999999999999996, -0.8, 2.2, 0.19999999999999996, -0.8, -0.8, -0.8, 2.2, -0.8, 0.19999999999999996, 1.2, -0.8, -0.8, 2.2, -0.8, -0.8, -0.8, 0.19999999999999996, 0.19999999999999996, 0.19999999999999996, 0.19999999999999996, 0.19999999999999996, 0.19999999999999996, 0.19999999999999996, 0.19999999999999996], [19294.0, 19383.0, 12665.0, 82.0, 158.0, 138.0, 161.0, 187.0, 205.0, 261.0, 296.0, 334.0, 378.0, 440.0, 415.0, 416.0, 435.0, 441.0, 423.0, 447.0, 475.0, 428.0, 428.0, 401.0, 450.0, 426.0, 399.0, 402.0, 399.0, 373.0, 355.0, 268.0, 290.0, 269.0, 263.0, 242.0, 217.0, 232.0, 225.0, 221.0, 193.0, 167.0, 177.0, 157.0, 146.0, 145.0, 148.0, 136.0, 124.0, 104.0, 116.0, 111.0, 127.0, 131.0, 108.0, 105.0, 91.0, 101.0, 82.0, 80.0, 58.0, 78.0, 46.0, 57.0, 44.0, 66.0, 56.0, 80.0, 89.0, 78.0, 84.0, 83.0, 75.0, 76.0, 66.0, 73.0, 84.0, 87.0, 93.0, 66.0, 54.0, 39.0, 41.0, 30.0, 35.0, 48.0, 31.0, 36.0, 18.0, 12.0, 14.0, 28.0, 25.0, 17.0, 13.0, 10.0, 24.0, 16.0, 25.0, 21.0, 24.0, 21.0, 17.0, 15.0, 11.0, 13.0, 6.0, 10.0, 8.0, 13.0, 8.0, 11.0, 7.0, 9.0, 12.0, 10.0, 9.0, 11.0, 13.0, 10.0, 10.0, 12.0, 1.0, 6.0, 5.0, 4.0, 8.0, 4.0, 9.0, 4.0, 5.0, 6.0, 9.0, 3.0, 7.0, 8.0, 5.0, 3.0, 8.0, 3.0, 8.0, 13.0, 2.0, 3.0, 7.0, 6.0, 4.0, 5.0, 6.0, 1.0, 3.0, 3.0, 1.0, 4.0, 3.0, 0.0, 6.0, 0.0, 4.0, 5.0, 0.0, 0.0, 2.0, 6.0, 2.0, 3.0, 0.0, 4.0, 4.0, 2.0, 1.0, 3.0, 1.0, 1.0, 2.0, 3.0, 0.0, 3.0, 0.0, -2.0, 2.0, -1.0, 1.0, 0.0, 0.0, 4.0, 2.0, 0.0, 0.0, -2.0, 1.0, -1.0, 1.0, 0.0, 0.0, 0.0, -1.0, 0.0, 1.0, 3.0, 0.0, 3.0, 4.0, -1.0, 1.0, 0.0, -1.0, -2.0, 4.0, 1.0, -1.0, -1.0, 1.0, 1.0, 2.0, 1.0, -1.0, 2.0, 2.0, -1.0, -1.0, 0.0, 0.0, -2.0, 0.0, -1.0, -1.0, 0.0, -1.0, -1.0, -1.0, 4.0, 1.0, 3.0, 3.0, 2.0, 0.0, -2.0, 0.0, 0.0, -1.0, -1.0, -2.0, 0.0, -1.0, -2.0, -2.0, 2.0, 2.0, 0.0, -2.0, -1.0, -1.0, -2.0, 1.0, -1.0, 0.0, -1.0, -2.0, 0.0, -2.0, 3.0, -2.0, 3.0, 0.0, -2.0, -1.0, 1.0, 1.0, -1.0, 1.0, -1.0, -1.0, 0.0, 1.0, 1.0, 1.0, -1.0, 0.0], [18604.8, 18754.8, 12488.8, 81.8, 93.8, 134.8, 132.8, 177.8, 213.8, 284.8, 300.8, 337.8, 381.8, 408.8, 427.8, 432.8, 486.8, 486.8, 461.8, 461.8, 483.8, 455.8, 433.8, 360.8, 430.8, 405.8, 385.8, 383.8, 371.8, 345.8, 283.8, 311.8, 287.8, 263.8, 232.8, 207.8, 240.8, 208.8, 183.8, 202.8, 186.8, 170.8, 169.8, 184.8, 143.8, 120.8, 123.8, 118.8, 138.8, 122.8, 106.8, 101.8, 105.8, 95.8, 109.8, 110.8, 93.8, 69.8, 65.8, 73.8, 74.8, 55.8, 51.8, 43.8, 58.8, 47.8, 46.8, 65.8, 116.8, 117.8, 78.8, 67.8, 80.8, 80.8, 80.8, 73.8, 58.8, 91.8, 75.8, 69.8, 67.8, 49.8, 29.8, 32.8, 27.8, 25.8, 18.8, 20.8, 20.8, 22.8, 25.8, 22.8, 17.8, 16.8, 21.8, 18.8, 14.8, 16.8, 9.8, 16.8, 18.8, 20.8, 10.8, 10.8, 11.8, 11.8, 5.8, 5.8, 7.8, 10.8, 12.8, 10.8, 8.8, 9.8, 10.8, 10.8, 12.8, 6.8, 8.8, 4.8, 4.8, 8.8, 7.8, 5.8, 8.8, 4.8, 3.8, 11.8, 4.8, 8.8, 2.8, 9.8, 10.8, 12.8, 4.8, 9.8, 3.8, 4.8, 6.8, 0.8, 4.8, 4.8, 1.8, 4.8, 3.8, 1.8, 2.8, 5.8, 3.8, 2.8, 3.8, 7.8, 1.8, 1.8, 1.8, 1.8, 3.8, 3.8, -0.19999999999999996, 1.8, 0.8, 1.8, 1.8, 6.8, 2.8, 6.8, 8.8, 5.8, 3.8, 1.8, 1.8, 4.8, 5.8, 1.8, 3.8, 5.8, 0.8, 1.8, 0.8, 0.8, 4.8, 0.8, 3.8, 1.8, 4.8, -0.19999999999999996, -0.19999999999999996, 1.8, -1.2, 3.8, 1.8, 0.8, 0.8, -0.19999999999999996, 3.8, 4.8, 0.8, -0.19999999999999996, -0.19999999999999996, 0.8, 1.8, -0.19999999999999996, 0.8, 0.8, 0.8, 0.8, 0.8, 1.8, -0.19999999999999996, 0.8, 0.8, 1.8, 1.8, 2.8, -0.19999999999999996, -1.2, 2.8, 2.8, -0.19999999999999996, -0.19999999999999996, -0.19999999999999996, -0.19999999999999996, 3.8, -0.19999999999999996, -1.2, -1.2, -0.19999999999999996, 1.8, 3.8, -0.19999999999999996, 0.8, 0.8, 1.8, 0.8, 2.8, -0.19999999999999996, -1.2, 2.8, -1.2, 0.8, -0.19999999999999996, -0.19999999999999996, -0.19999999999999996, -0.19999999999999996, -0.19999999999999996, -0.19999999999999996, 1.8, -0.19999999999999996, -1.2, -0.19999999999999996, -1.2, 2.8, -1.2, 1.8, -1.2, -1.2, 0.8, 1.8, -0.19999999999999996, -0.19999999999999996, -0.19999999999999996, -0.19999999999999996, -0.19999999999999996, -0.19999999999999996, 1.8, -1.2, 2.8, 1.8, -0.19999999999999996, -0.19999999999999996, 1.8, -0.19999999999999996, 0.8, -0.19999999999999996, 0.8, -1.2, 0.8, -1.2, -1.2], [17832.1, 18048.1, 12179.1, 70.1, 100.1, 141.1, 146.1, 159.1, 160.1, 175.1, 216.1, 258.1, 260.1, 329.1, 351.1, 364.1, 350.1, 374.1, 414.1, 404.1, 370.1, 408.1, 394.1, 416.1, 385.1, 398.1, 372.1, 354.1, 396.1, 340.1, 323.1, 348.1, 279.1, 246.1, 218.1, 205.1, 220.1, 231.1, 228.1, 187.1, 193.1, 187.1, 160.1, 155.1, 160.1, 144.1, 137.1, 128.1, 122.1, 123.1, 120.1, 95.1, 97.1, 99.1, 107.1, 105.1, 92.1, 74.1, 71.1, 88.1, 64.1, 56.1, 60.1, 47.1, 50.1, 53.1, 56.1, 74.1, 290.1, 325.1, 99.1, 78.1, 85.1, 81.1, 74.1, 70.1, 71.1, 67.1, 76.1, 67.1, 59.1, 53.1, 35.1, 36.1, 38.1, 20.1, 23.1, 23.1, 27.1, 22.1, 23.1, 11.1, 17.1, 21.1, 9.1, 26.1, 21.1, 18.1, 20.1, 20.1, 10.1, 9.1, 11.1, 17.1, 17.1, 13.1, 9.1, 12.1, 9.1, 13.1, 14.1, 10.1, 10.1, 9.1, 7.1, 8.1, 14.1, 10.1, 5.1, 9.1, 13.1, 8.1, 7.1, 9.1, 3.1, 6.1, 11.1, 10.1, 10.1, 7.1, 8.1, 2.1, 1.1, 8.1, 9.1, 5.1, 4.1, 10.1, 10.1, 5.1, 2.1, 9.1, 4.1, 7.1, 2.1, 9.1, 0.10000000000000009, 2.1, 3.1, 2.1, 1.1, 0.10000000000000009, 2.1, 7.1, 5.1, 4.1, 0.10000000000000009, 2.1, 3.1, 1.1, -0.8999999999999999, 1.1, 3.1, 0.10000000000000009, 3.1, 2.1, -0.8999999999999999, 4.1, 1.1, 4.1, 6.1, 2.1, 2.1, 4.1, 3.1, 3.1, 0.10000000000000009, 6.1, 2.1, 0.10000000000000009, -0.8999999999999999, 1.1, -0.8999999999999999, 2.1, -0.8999999999999999, -1.9, 1.1, -1.9, 1.1, 1.1, 1.1, 1.1, 2.1, 2.1, -0.8999999999999999, 2.1, 0.10000000000000009, 2.1, -0.8999999999999999, 1.1, 4.1, 2.1, 1.1, 1.1, 1.1, 0.10000000000000009, 3.1, 3.1, 5.1, 1.1, -0.8999999999999999, 1.1, 0.10000000000000009, 0.10000000000000009, 2.1, 1.1, 2.1, 1.1, -0.8999999999999999, 1.1, 0.10000000000000009, 1.1, -1.9, -0.8999999999999999, 0.10000000000000009, -1.9, 0.10000000000000009, -0.8999999999999999, -0.8999999999999999, 2.1, -0.8999999999999999, 1.1, 1.1, -0.8999999999999999, -0.8999999999999999, 3.1, 0.10000000000000009, 0.10000000000000009, 0.10000000000000009, -0.8999999999999999, -0.8999999999999999, 0.10000000000000009, -1.9, -0.8999999999999999, 0.10000000000000009, 1.1, -0.8999999999999999, -1.9, 0.10000000000000009, -1.9, 2.1, -0.8999999999999999, -0.8999999999999999, -1.9, 2.1, -1.9, -0.8999999999999999, -0.8999999999999999, -0.8999999999999999, -0.8999999999999999, -0.8999999999999999, -1.9, 0.10000000000000009, -1.9, -1.9, -0.8999999999999999, 1.1, -1.9, 1.1, 0.10000000000000009, -1.9, 2.1, 2.1, -1.9, -0.8999999999999999, -1.9, 0.10000000000000009, 1.1, 1.1], [18621.7, 19022.7, 12283.7, 61.7, 87.7, 132.7, 127.7, 163.7, 144.7, 183.7, 190.7, 232.7, 284.7, 309.7, 368.7, 343.7, 374.7, 377.7, 397.7, 411.7, 421.7, 420.7, 399.7, 367.7, 392.7, 373.7, 352.7, 393.7, 344.7, 333.7, 340.7, 318.7, 318.7, 297.7, 257.7, 241.7, 259.7, 227.7, 214.7, 217.7, 207.7, 169.7, 176.7, 154.7, 155.7, 167.7, 140.7, 127.7, 127.7, 115.7, 113.7, 133.7, 122.7, 137.7, 99.7, 112.7, 80.7, 83.7, 90.7, 79.7, 65.7, 59.7, 50.7, 43.7, 56.7, 67.7, 78.7, 75.7, 231.7, 439.7, 187.7, 71.7, 85.7, 80.7, 86.7, 63.7, 80.7, 75.7, 97.7, 45.7, 59.7, 40.7, 35.7, 31.7, 37.7, 31.7, 25.7, 28.7, 26.7, 23.7, 18.7, 19.7, 16.7, 20.7, 22.7, 17.7, 18.7, 20.7, 19.7, 12.7, 18.7, 21.7, 15.7, 15.7, 14.7, 10.7, 14.7, 19.7, 3.7, 13.7, 10.7, 13.7, 9.7, 18.7, 4.7, 18.7, 5.7, 8.7, 9.7, 13.7, 10.7, 9.7, 7.7, 5.7, 15.7, 6.7, 7.7, 7.7, 3.7, 7.7, 8.7, 4.7, 7.7, 7.7, 3.7, 6.7, 9.7, 0.7, 9.7, 6.7, 0.7, 5.7, 2.7, 2.7, 4.7, 6.7, 2.7, 3.7, 2.7, 7.7, 1.7, 3.7, 4.7, 5.7, 6.7, 6.7, 0.7, 1.7, 5.7, 2.7, -1.3, 1.7, 2.7, 5.7, 0.7, -0.30000000000000004, 1.7, 2.7, 2.7, 2.7, 0.7, 0.7, 2.7, 7.7, 5.7, 4.7, 3.7, 4.7, 5.7, 1.7, 4.7, 3.7, 3.7, 1.7, -0.30000000000000004, -0.30000000000000004, -0.30000000000000004, 1.7, 1.7, 2.7, 1.7, 2.7, 3.7, 2.7, 0.7, 0.7, 0.7, 2.7, 1.7, 2.7, 1.7, 1.7, 1.7, 2.7, 0.7, 0.7, 0.7, 0.7, -0.30000000000000004, 3.7, 0.7, 1.7, 0.7, -1.3, 0.7, -0.30000000000000004, 0.7, 0.7, 0.7, 0.7, -0.30000000000000004, -1.3, -0.30000000000000004, 0.7, 0.7, 0.7, -0.30000000000000004, -0.30000000000000004, -0.30000000000000004, 2.7, -0.30000000000000004, -0.30000000000000004, 0.7, -0.30000000000000004, 0.7, -0.30000000000000004, -1.3, -0.30000000000000004, 0.7, -0.30000000000000004, -0.30000000000000004, 1.7, 1.7, -1.3, -1.3, 0.7, 2.7, 1.7, -0.30000000000000004, -0.30000000000000004, -0.30000000000000004, 1.7, 4.7, 1.7, -1.3, -1.3, -1.3, -1.3, -0.30000000000000004, 0.7, 0.7, 1.7, -0.30000000000000004, -1.3, 2.7, 0.7, -0.30000000000000004, -0.30000000000000004, -0.30000000000000004, -0.30000000000000004, 1.7, 0.7, -1.3, -0.30000000000000004, -0.30000000000000004, -0.30000000000000004, -0.30000000000000004, -1.3, 1.7], [18536.4, 18948.4, 12753.4, 57.4, 88.4, 100.4, 96.4, 122.4, 161.4, 203.4, 253.4, 274.4, 331.4, 368.4, 410.4, 334.4, 363.4, 412.4, 380.4, 395.4, 453.4, 395.4, 418.4, 429.4, 400.4, 403.4, 405.4, 396.4, 343.4, 340.4, 325.4, 316.4, 292.4, 275.4, 237.4, 224.4, 220.4, 222.4, 217.4, 204.4, 187.4, 198.4, 181.4, 148.4, 135.4, 140.4, 124.4, 136.4, 123.4, 107.4, 124.4, 114.4, 122.4, 122.4, 107.4, 89.4, 82.4, 72.4, 72.4, 83.4, 69.4, 58.4, 56.4, 58.4, 56.4, 48.4, 60.4, 47.4, 57.4, 61.4, 63.4, 60.4, 62.4, 85.4, 72.4, 67.4, 71.4, 67.4, 66.4, 67.4, 40.4, 46.4, 36.4, 38.4, 25.4, 27.4, 30.4, 26.4, 23.4, 21.4, 20.4, 19.4, 20.4, 17.4, 15.4, 8.4, 15.4, 15.4, 15.4, 14.4, 11.4, 10.4, 14.4, 18.4, 9.4, 17.4, 13.4, 9.4, 11.4, 10.4, 12.4, 4.4, 8.4, 5.4, 10.4, 9.4, 3.4, 5.4, 7.4, 6.4, 9.4, 3.4, 10.4, 11.4, 10.4, 3.4, 4.4, 4.4, 5.4, 7.4, 7.4, 9.4, 8.4, 5.4, 10.4, 3.4, 2.4, 3.4, 3.4, 7.4, 5.4, 5.4, 4.4, 1.4, 1.4, 5.4, 4.4, 5.4, 2.4, 6.4, 6.4, 4.4, 4.4, 0.3999999999999999, 1.4, 5.4, 0.3999999999999999, 2.4, 1.4, 2.4, 5.4, 1.4, 3.4, -0.6000000000000001, 1.4, 3.4, 6.4, 6.4, 3.4, 4.4, 0.3999999999999999, 1.4, 0.3999999999999999, 2.4, 1.4, 2.4, 1.4, -0.6000000000000001, 0.3999999999999999, -0.6000000000000001, 0.3999999999999999, 3.4, 2.4, 1.4, -0.6000000000000001, -0.6000000000000001, 5.4, -0.6000000000000001, 3.4, 1.4, -0.6000000000000001, 1.4, -0.6000000000000001, 0.3999999999999999, -0.6000000000000001, 0.3999999999999999, -1.6, 0.3999999999999999, 1.4, 0.3999999999999999, 2.4, 1.4, 1.4, 1.4, 3.4, 0.3999999999999999, 0.3999999999999999, 1.4, 1.4, 0.3999999999999999, 1.4, 1.4, -0.6000000000000001, 1.4, 0.3999999999999999, -0.6000000000000001, -0.6000000000000001, -0.6000000000000001, -0.6000000000000001, -0.6000000000000001, 0.3999999999999999, 0.3999999999999999, -0.6000000000000001, -0.6000000000000001, 1.4, 1.4, 0.3999999999999999, 0.3999999999999999, -0.6000000000000001, 0.3999999999999999, -0.6000000000000001, 0.3999999999999999, 0.3999999999999999, -1.6, -0.6000000000000001, -0.6000000000000001, -1.6, -0.6000000000000001, -0.6000000000000001, 1.4, 0.3999999999999999, -0.6000000000000001, -0.6000000000000001, -0.6000000000000001, -0.6000000000000001, -1.6, 1.4, 3.4, -1.6, 0.3999999999999999, 1.4, 1.4, -1.6, 1.4, -0.6000000000000001, -0.6000000000000001, 1.4, 0.3999999999999999, -0.6000000000000001, -0.6000000000000001, 0.3999999999999999, 0.3999999999999999, -0.6000000000000001, 0.3999999999999999, -0.6000000000000001, -0.6000000000000001, -1.6, -0.6000000000000001, 0.3999999999999999, 1.4, -0.6000000000000001, 0.3999999999999999, 1.4, 1.4, -1.6, -1.6, -0.6000000000000001, 1.4, -1.6], [18904.6, 19301.6, 12745.6, 53.6, 90.6, 105.6, 102.6, 117.6, 140.6, 195.6, 196.6, 261.6, 312.6, 324.6, 397.6, 388.6, 362.6, 383.6, 396.6, 364.6, 378.6, 396.6, 340.6, 345.6, 370.6, 323.6, 343.6, 375.6, 317.6, 324.6, 295.6, 269.6, 273.6, 245.6, 213.6, 221.6, 204.6, 232.6, 210.6, 181.6, 200.6, 185.6, 148.6, 157.6, 155.6, 119.6, 131.6, 121.6, 123.6, 135.6, 112.6, 114.6, 117.6, 121.6, 93.6, 104.6, 88.6, 101.6, 75.6, 71.6, 69.6, 61.6, 54.6, 55.6, 56.6, 51.6, 48.6, 59.6, 121.6, 86.6, 72.6, 54.6, 57.6, 66.6, 67.6, 56.6, 66.6, 71.6, 55.6, 43.6, 48.6, 36.6, 29.6, 34.6, 32.6, 36.6, 31.6, 21.6, 11.6, 20.6, 21.6, 16.6, 16.6, 11.6, 13.6, 20.6, 16.6, 15.6, 21.6, 12.6, 13.6, 18.6, 8.6, 13.6, 15.6, 13.6, 14.6, 17.6, 5.6, 15.6, 15.6, 9.6, 9.6, 4.6, 8.6, 11.6, 9.6, 6.6, 4.6, 8.6, 13.6, 6.6, 6.6, 11.6, 7.6, 9.6, 6.6, 10.6, 3.6, 5.6, 4.6, 8.6, 9.6, 6.6, 2.6, 5.6, 8.6, 3.6, 5.6, 2.6, 3.6, 5.6, 2.6, 2.6, 3.6, 1.6, 6.6, 3.6, 6.6, 0.6000000000000001, 5.6, 5.6, 0.6000000000000001, 2.6, 9.6, 3.6, 0.6000000000000001, 5.6, 4.6, 2.6, 3.6, 3.6, 1.6, 2.6, 1.6, 2.6, 5.6, 0.6000000000000001, 0.6000000000000001, -0.3999999999999999, -0.3999999999999999, -0.3999999999999999, 5.6, 5.6, 3.6, 2.6, 0.6000000000000001, 3.6, 3.6, 0.6000000000000001, -0.3999999999999999, 1.6, 1.6, 3.6, 0.6000000000000001, 1.6, 1.6, 2.6, 0.6000000000000001, 1.6, -0.3999999999999999, 5.6, 0.6000000000000001, 1.6, -0.3999999999999999, 0.6000000000000001, 1.6, 4.6, 1.6, 1.6, 2.6, 2.6, 1.6, 3.6, 0.6000000000000001, 5.6, 2.6, -0.3999999999999999, 2.6, -0.3999999999999999, -1.4, 3.6, -1.4, -0.3999999999999999, 0.6000000000000001, -0.3999999999999999, 2.6, 2.6, 0.6000000000000001, 0.6000000000000001, 1.6, 0.6000000000000001, 5.6, 0.6000000000000001, -1.4, -1.4, 1.6, -0.3999999999999999, -0.3999999999999999, 0.6000000000000001, 0.6000000000000001, 0.6000000000000001, -0.3999999999999999, 0.6000000000000001, 2.6, -0.3999999999999999, -0.3999999999999999, 3.6, -0.3999999999999999, 3.6, 0.6000000000000001, 0.6000000000000001, -0.3999999999999999, -1.4, -0.3999999999999999, 0.6000000000000001, -1.4, -0.3999999999999999, 0.6000000000000001, -0.3999999999999999, -0.3999999999999999, -0.3999999999999999, 0.6000000000000001, -1.4, 0.6000000000000001, 0.6000000000000001, -0.3999999999999999, 1.6, 0.6000000000000001, -0.3999999999999999, 0.6000000000000001, -0.3999999999999999, 0.6000000000000001, -1.4, 0.6000000000000001, -1.4, 0.6000000000000001, 0.6000000000000001, 0.6000000000000001, -1.4, 0.6000000000000001, -1.4, -0.3999999999999999, 0.6000000000000001, 0.6000000000000001, 0.6000000000000001, -1.4, 3.6, -1.4], [17306.8, 17931.8, 11994.8, 63.8, 87.8, 157.8, 199.8, 172.8, 166.8, 188.8, 222.8, 245.8, 272.8, 335.8, 348.8, 378.8, 343.8, 380.8, 384.8, 415.8, 366.8, 399.8, 371.8, 360.8, 365.8, 359.8, 360.8, 361.8, 338.8, 311.8, 270.8, 283.8, 287.8, 244.8, 262.8, 230.8, 234.8, 197.8, 190.8, 210.8, 164.8, 161.8, 146.8, 142.8, 154.8, 132.8, 137.8, 126.8, 135.8, 143.8, 139.8, 108.8, 109.8, 105.8, 92.8, 85.8, 81.8, 81.8, 73.8, 79.8, 54.8, 64.8, 45.8, 50.8, 58.8, 52.8, 65.8, 47.8, 56.8, 61.8, 53.8, 65.8, 73.8, 45.8, 42.8, 59.8, 63.8, 58.8, 47.8, 34.8, 27.8, 21.8, 38.8, 32.8, 41.8, 40.8, 27.8, 24.8, 29.8, 24.8, 13.8, 21.8, 17.8, 18.8, 14.8, 21.8, 13.8, 25.8, 14.8, 12.8, 12.8, 22.8, 27.8, 17.8, 12.8, 9.8, 18.8, 7.8, 12.8, 14.8, 13.8, 9.8, 15.8, 13.8, 11.8, 10.8, 10.8, 11.8, 15.8, 10.8, 4.8, 10.8, 4.8, 6.8, 11.8, 6.8, 5.8, 8.8, 1.8, 7.8, 8.8, 8.8, 7.8, 7.8, 7.8, 4.8, 9.8, 7.8, 3.8, 4.8, 7.8, 5.8, 5.8, 4.8, 5.8, 5.8, 6.8, 3.8, 3.8, 6.8, 8.8, 2.8, 3.8, 1.8, 5.8, 5.8, 8.8, 7.8, 0.8, 0.8, -1.2, 6.8, 2.8, 1.8, 2.8, 0.8, 1.8, 2.8, 3.8, 1.8, 0.8, 2.8, 0.8, 2.8, 1.8, 0.8, 1.8, 2.8, 0.8, 0.8, 0.8, 2.8, 1.8, -0.19999999999999996, 4.8, -0.19999999999999996, 2.8, 1.8, 1.8, 3.8, -0.19999999999999996, 0.8, 5.8, 1.8, -1.2, -0.19999999999999996, 1.8, -1.2, 1.8, -1.2, 0.8, -1.2, -0.19999999999999996, 0.8, -1.2, 2.8, 0.8, 0.8, 4.8, 2.8, 0.8, -0.19999999999999996, 0.8, 0.8, 0.8, 0.8, -0.19999999999999996, 2.8, 0.8, 1.8, 0.8, 0.8, 1.8, -1.2, 1.8, 2.8, 5.8, -1.2, -0.19999999999999996, -0.19999999999999996, 0.8, -1.2, -0.19999999999999996, 0.8, -0.19999999999999996, -0.19999999999999996, -0.19999999999999996, -1.2, -1.2, -0.19999999999999996, 3.8, -0.19999999999999996, 1.8, -0.19999999999999996, 1.8, -0.19999999999999996, 1.8, -1.2, -1.2, 0.8, -1.2, 2.8, -1.2, -1.2, -0.19999999999999996, -1.2, -0.19999999999999996, 0.8, -0.19999999999999996, -1.2, -0.19999999999999996, -1.2, -1.2, -0.19999999999999996, -0.19999999999999996, -0.19999999999999996, 0.8, -0.19999999999999996, -0.19999999999999996, -0.19999999999999996, -1.2, 1.8, 0.8, -0.19999999999999996, -1.2, 0.8, -1.2, 0.8, -0.19999999999999996], [18278.0, 18888.0, 12295.0, 56.0, 70.0, 153.0, 168.0, 165.0, 163.0, 165.0, 189.0, 236.0, 292.0, 276.0, 310.0, 322.0, 344.0, 353.0, 342.0, 403.0, 403.0, 404.0, 403.0, 383.0, 406.0, 363.0, 369.0, 342.0, 369.0, 342.0, 286.0, 304.0, 270.0, 259.0, 236.0, 241.0, 232.0, 189.0, 177.0, 211.0, 190.0, 173.0, 166.0, 148.0, 182.0, 138.0, 147.0, 130.0, 136.0, 133.0, 111.0, 124.0, 107.0, 100.0, 113.0, 72.0, 83.0, 73.0, 73.0, 81.0, 65.0, 67.0, 70.0, 37.0, 49.0, 67.0, 49.0, 46.0, 54.0, 38.0, 57.0, 72.0, 66.0, 62.0, 65.0, 69.0, 64.0, 54.0, 38.0, 41.0, 26.0, 46.0, 31.0, 30.0, 32.0, 34.0, 27.0, 27.0, 22.0, 19.0, 19.0, 11.0, 18.0, 19.0, 27.0, 18.0, 10.0, 11.0, 23.0, 19.0, 17.0, 32.0, 21.0, 17.0, 18.0, 11.0, 11.0, 13.0, 13.0, 10.0, 14.0, 18.0, 22.0, 11.0, 8.0, 11.0, 14.0, 13.0, 8.0, 5.0, 3.0, 9.0, 8.0, 8.0, 8.0, 6.0, 5.0, 10.0, 9.0, 11.0, 6.0, 7.0, 6.0, 1.0, 2.0, 2.0, 8.0, 6.0, 3.0, 6.0, 4.0, 2.0, 9.0, 8.0, 4.0, 3.0, 4.0, 0.0, -1.0, 1.0, 2.0, 0.0, 4.0, 4.0, 7.0, 2.0, 3.0, 5.0, 6.0, 5.0, 3.0, 0.0, 4.0, 1.0, 3.0, 5.0, 5.0, 6.0, 2.0, 1.0, 2.0, 7.0, 5.0, 2.0, 3.0, 1.0, 2.0, 2.0, 2.0, 5.0, 6.0, 4.0, 3.0, 2.0, 1.0, 2.0, 1.0, 6.0, 5.0, 7.0, 1.0, 0.0, 2.0, 2.0, 4.0, 2.0, 6.0, 2.0, 0.0, 2.0, 2.0, 3.0, 1.0, 2.0, 0.0, 0.0, 0.0, -1.0, 1.0, -1.0, 2.0, 3.0, 3.0, 0.0, -1.0, 2.0, 3.0, 2.0, -1.0, 0.0, -1.0, 1.0, 3.0, 3.0, -1.0, 1.0, 1.0, 1.0, -1.0, 1.0, 3.0, 2.0, 2.0, 4.0, 4.0, 3.0, -1.0, 0.0, 0.0, 0.0, 1.0, -1.0, -1.0, 1.0, 1.0, 1.0, 0.0, 0.0, 2.0, 1.0, 1.0, -1.0, 1.0, 3.0, 2.0, -1.0, -1.0, -1.0, -1.0, 2.0, 0.0, 0.0, 0.0, 0.0, 0.0, 1.0, 2.0, 1.0, -1.0, -1.0, 1.0, -1.0, 0.0, 0.0, 0.0, 1.0, -1.0, 1.0, 0.0]]
  in  "Weather":T3(tab)=enum."Background (Mc/s)"
  in  "Temperature (C)":dbl=15.0
  out "Temperature (C)":dbl(graph)=15.0
  in  "Pressure (mbar or hPa)":dbl=832.0
  out "Pressure (mb)":dbl(graph)=832.0
  out "Relative Humdity (%)":dbl(graph)=40.0
  out "Pulse Energy (Micro Joule)":T4(graph)
  in  "PRF (kHz)":dbl=7.0
  out "?":cluster{"mean":dbl, "mean":dbl}(graph)={"mean"=380.0, "mean"=360.0}
  out "Index":i32=92
  out "Aerosol Smoothed":dbl[](array[numeric])=[18272.438461538462, 15416.053846153845, 6142.092307692307, 73.13076923076923, 103.28461538461538, 124.97692307692307, 134.7076923076923, 143.7846153846154, 166.7846153846154, 198.43846153846152, 227.51538461538462, 266.36153846153843, 303.4, 329.2461538461538, 342.28461538461534, 348.9769230769231, 361.7076923076923, 369.9769230769231, 372.9384615384615, 380.5153846153846, 384.5538461538462, 379.28461538461545, 369.9, 366.7461538461538, 365.66923076923075, 360.16923076923075, 355.66923076923075, 344.5153846153846, 331.59230769230766, 313.4384615384615, 291.74615384615385, 276.55384615384617, 261.6307692307692, 241.16923076923075, 223.01538461538462, 218.36153846153843, 209.93846153846152, 199.3615384615385, 195.01538461538465, 184.13076923076926, 172.7076923076923, 163.05384615384614, 152.7076923076923, 147.7846153846154, 139.55384615384617, 131.09230769230768, 126.5153846153846, 122.93846153846154, 118.05384615384615, 112.2076923076923, 110.97692307692307, 110.4, 110.55384615384617, 104.09230769230768, 94.51538461538459, 87.63076923076923, 79.97692307692309, 75.32307692307694, 73.28461538461539, 67.01538461538462, 59.861538461538466, 56.24615384615385, 51.05384615384615, 49.78461538461538, 52.784615384615385, 54.05384615384616, 55.823076923076925, 77.36153846153847, 107.36153846153846, 97.36153846153846, 71.0923076923077, 66.86153846153846, 68.51538461538462, 66.63076923076923, 64.47692307692307, 62.476923076923086, 61.93846153846154, 60.861538461538466, 54.976923076923086, 47.20769230769231, 42.400000000000006, 37.24615384615385, 33.01538461538462, 32.823076923076925, 31.823076923076925, 27.592307692307696, 23.9, 22.4, 20.784615384615385, 19.553846153846152, 19.284615384615385, 18.630769230769232, 16.976923076923075, 16.707692307692305, 16.630769230769232, 16.092307692307692, 16.43846153846154, 16.823076923076925, 16.16923076923077, 15.323076923076922, 16.207692307692305, 15.399999999999999, 14.246153846153845, 14.053846153846155, 13.630769230769232, 13.861538461538462, 13.130769230769232, 11.630769230769232, 12.092307692307692, 13.976923076923075, 13.669230769230769, 11.669230769230769, 9.976923076923075, 9.053846153846152, 10.13076923076923, 10.476923076923077, 9.015384615384615, 8.592307692307692, 8.707692307692309, 9.015384615384615, 8.86153846153846, 8.13076923076923, 7.707692307692307, 7.746153846153845, 6.707692307692307, 6.4, 7.015384615384615, 6.553846153846154, 6.361538461538461, 6.323076923076924, 6.2846153846153845, 6.438461538461539, 6.207692307692308, 5.823076923076924, 5.592307692307692, 5.861538461538461, 5.63076923076923, 5.438461538461539, 4.938461538461539, 4.592307692307692, 5.476923076923076, 5.169230769230769, 4.438461538461539, 4.1692307692307695, 4.1692307692307695, 4.669230769230769, 4.246153846153846, 3.5153846153846153, 3.4384615384615387, 3.707692307692308, 3.2846153846153845, 2.861538461538462, 3.0538461538461537, 3.5538461538461537, 3.6692307692307695, 3.130769230769231, 3.323076923076923, 3.361538461538461, 2.669230769230769, 1.8615384615384616, 2.0923076923076924, 2.707692307692308, 2.592307692307693, 2.4000000000000004, 2.5538461538461537, 2.9384615384615387, 3.3230769230769237, 2.976923076923077, 2.246153846153846, 2.092307692307693, 2.130769230769231, 2.4384615384615387, 2.553846153846154, 2.553846153846154, 2.4384615384615387, 1.7846153846153845, 1.9, 2.4000000000000004, 1.976923076923077, 1.7846153846153847, 1.8615384615384616, 1.9384615384615385, 1.8230769230769233, 1.9, 1.6307692307692307, 1.5153846153846158, 1.5923076923076924, 1.3615384615384616, 1.669230769230769, 1.2076923076923076, 1.0153846153846153, 1.823076923076923, 1.5923076923076924, 1.0538461538461539, 1.323076923076923, 1.0538461538461537, 0.8999999999999999, 0.9769230769230768, 1.0923076923076924, 1.6307692307692307, 1.5538461538461539, 1.2076923076923076, 0.9384615384615383, 0.7076923076923076, 0.9384615384615383, 1.0153846153846153, 0.7846153846153845, 1.2846153846153847, 1.2461538461538462, 0.5153846153846153, 0.7846153846153846, 0.976923076923077, 0.7076923076923076, 0.6307692307692307, 0.4769230769230769, 0.5538461538461539, 1.3615384615384616, 1.2461538461538462, 0.4769230769230769, 0.2846153846153846, 0.2846153846153846, 0.7846153846153845, 0.6307692307692306, 0.09230769230769231, 0.32307692307692304, 0.7461538461538462, 0.43846153846153846, 0.1307692307692307, 0.32307692307692304, 0.3230769230769231, 0.7076923076923077, 0.7076923076923077, 0.3230769230769231, 0.5923076923076923, 0.823076923076923, 0.13076923076923075, -0.21538461538461542, -0.06153846153846155, 0.05384615384615386, 0.4769230769230769, 0.36153846153846153, 0.24615384615384608, 0.053846153846153794, -0.1769230769230769, -0.06153846153846154, 0.13076923076923078, 0.16923076923076924, -0.176923076923077, -0.06153846153846161, 0.09230769230769229, 0.20769230769230762, 0.3615384615384615, 0.16923076923076924, 0.2076923076923077, -0.21538461538461542, -0.36923076923076925, -0.02307692307692307, -0.21538461538461542, -0.13846153846153852, -0.023076923076923106, 0.09230769230769222, -0.02307692307692319, -0.2538461538461539, 0.09230769230769231, -0.0615384615384616, -0.061538461538461625, 0.4, 0.3999999999999999, 0.1307692307692307, -0.023076923076923085, 0.09230769230769231, 0.2076923076923077, 0.015384615384615358, -0.17692307692307696, -0.1384615384615384, -0.17692307692307688, 0.09230769230769233]
  out "Off-Line  Bin Readings":dbl[](array[numeric])=[16899.0, 18437.0, 11498.0, 31.0, 49.0, 67.0, 97.0, 96.0, 88.0, 130.0, 130.0, 160.0, 207.0, 192.0, 196.0, 236.0, 225.0, 242.0, 270.0, 253.0, 280.0, 275.0, 263.0, 277.0, 279.0, 286.0, 256.0, 227.0, 258.0, 235.0, 240.0, 209.0, 217.0, 210.0, 180.0, 179.0, 187.0, 153.0, 176.0, 161.0, 133.0, 151.0, 137.0, 133.0, 126.0, 116.0, 118.0, 109.0, 115.0, 94.0, 100.0, 87.0, 97.0, 93.0, 77.0, 76.0, 67.0, 63.0, 58.0, 47.0, 55.0, 49.0, 45.0, 42.0, 43.0, 42.0, 49.0, 43.0, 39.0, 61.0, 46.0, 54.0, 58.0, 64.0, 47.0, 32.0, 42.0, 40.0, 41.0, 31.0, 22.0, 31.0, 24.0, 24.0, 28.0, 18.0, 17.0, 21.0, 12.0, 23.0, 23.0, 24.0, 16.0, 17.0, 17.0, 19.0, 16.0, 12.0, 19.0, 15.0, 14.0, 21.0, 7.0, 20.0, 19.0, 20.0, 12.0, 16.0, 17.0, 22.0, 18.0, 25.0, 9.0, 13.0, 5.0, 18.0, 9.0, 6.0, 10.0, 12.0, 12.0, 7.0, 9.0, 7.0, 5.0, 7.0, 5.0, 6.0, 6.0, 9.0, 9.0, 6.0, 7.0, 4.0, 4.0, 8.0, 5.0, 7.0, 8.0, 6.0, 4.0, 6.0, 7.0, 6.0, 6.0, 1.0, 5.0, 6.0, 5.0, 7.0, 5.0, 2.0, 9.0, 3.0, 4.0, 5.0, 3.0, 3.0, 6.0, 1.0, 1.0, 5.0, 2.0, 2.0, 4.0, 5.0, 3.0, 3.0, 3.0, 2.0, 4.0, 6.0, 4.0, 3.0, 6.0, 3.0, 2.0, 4.0, 1.0, 6.0, 1.0, 6.0, 2.0, 4.0, 3.0, 3.0, 3.0, 4.0, 2.0, 1.0, 3.0, 5.0, 3.0, 1.0, 3.0, 5.0, 2.0, 3.0, 2.0, 4.0, 4.0, 3.0, 2.0, 1.0, 1.0, 3.0, 1.0, 1.0, 2.0, 1.0, 0.0, 0.0, 3.0, 2.0, 3.0, 2.0, 1.0, 6.0, 1.0, 3.0, 2.0, 1.0, 5.0, 2.0, 3.0, 6.0, 0.0, 1.0, 2.0, 0.0, 1.0, 2.0, 2.0, 0.0, 1.0, 1.0, 0.0, 1.0, 2.0, 0.0, 0.0, 2.0, 4.0, 1.0, 1.0, 0.0, 1.0, 1.0, 0.0, 2.0, 0.0, 1.0, 1.0, 2.0, 2.0, 1.0, 0.0, 1.0, 0.0, 2.0, 0.0, 1.0, 2.0, 1.0, 0.0, 1.0, 1.0, 1.0, 3.0, 3.0, 2.0, 3.0, 1.0, 1.0, 2.0, 2.0, 0.0, 3.0, 2.0]
  out "Off-Line Smoothed":dbl[](array[numeric])=[16787.129032258068, 14411.543906810039, 5568.406810035844, 55.58333333333336, 79.1442652329749, 101.16845878136195, 108.58960573476699, 113.9901433691756, 128.7007168458781, 150.64247311827953, 177.3655913978494, 206.3306451612903, 232.74731182795693, 252.65322580645153, 266.07974910394256, 274.3387096774193, 280.1245519713261, 284.43100358422936, 286.5573476702508, 287.2706093189964, 288.9578853046595, 288.97580645161287, 286.6603942652329, 284.15860215053755, 279.88888888888874, 274.83422939068083, 268.56182795698913, 259.67741935483866, 249.09229390680997, 237.89784946236554, 225.84587813620072, 214.01523297491042, 202.0627240143369, 189.77240143369173, 179.18458781362003, 169.82616487455192, 161.7302867383512, 154.67204301075265, 147.53136200716844, 141.0232974910394, 134.47670250896053, 127.60573476702503, 121.87096774193543, 116.3360215053763, 110.73835125448025, 105.8969534050179, 101.25896057347668, 96.4901433691756, 92.40860215053758, 89.59587813620067, 87.97043010752682, 86.88530465949816, 83.61469534050175, 77.81093189964156, 70.5663082437276, 63.97401433691758, 59.50896057347671, 55.81899641577061, 53.02060931899641, 50.85752688172043, 48.75448028673836, 46.00268817204302, 42.97401433691758, 41.387992831541226, 41.485663082437284, 41.805555555555564, 43.741935483870975, 49.512544802867396, 53.71236559139786, 50.81810035842295, 46.6478494623656, 46.10394265232975, 46.24014336917563, 45.98924731182797, 46.01344086021506, 44.69623655913979, 41.75896057347671, 38.715053763440864, 35.51433691756273, 32.004480286738364, 28.603942652329756, 26.08243727598567, 24.171146953405028, 22.613799283154137, 20.901433691756278, 19.50179211469534, 18.520609318996414, 17.051971326164868, 16.24462365591397, 15.775089605734758, 15.207885304659495, 14.944444444444443, 14.57168458781362, 14.11111111111111, 13.89516129032258, 13.49372759856631, 12.886200716845877, 12.615591397849462, 12.302867383512545, 11.871863799283153, 12.327956989247312, 12.746415770609318, 11.748207885304657, 10.578853046594979, 10.263440860215052, 10.332437275985662, 9.99910394265233, 9.718637992831543, 9.882616487455195, 10.561827956989244, 10.97311827956989, 9.626344086021504, 8.287634408602148, 7.838709677419352, 7.562724014336915, 7.561827956989244, 7.433691756272398, 7.100358422939066, 6.809139784946236, 6.6200716845878125, 6.4829749103942635, 6.274193548387094, 6.0421146953405, 5.888888888888887, 5.758960573476699, 5.647849462365588, 5.456989247311824, 5.326164874551967, 5.18906810035842, 5.042114695340501, 4.947132616487455, 4.762544802867383, 4.626344086021504, 4.439964157706093, 4.281362007168461, 4.292114695340504, 4.275985663082439, 4.0994623655914, 3.9686379928315425, 3.948028673835127, 3.7965949820788536, 3.7016129032258065, 3.6129032258064515, 3.427419354838709, 3.3351254480286734, 3.2437275985663083, 3.1630824372759854, 3.1747311827956985, 3.124551971326165, 2.9802867383512552, 2.8718637992831546, 2.8001792114695347, 2.7437275985663088, 2.6496415770609323, 2.5143369175627246, 2.4668458781362013, 2.459677419354839, 2.4112903225806455, 2.376344086021505, 2.369175627240143, 2.306451612903226, 2.1711469534050183, 2.0268817204301084, 2.000000000000001, 2.0232974910394272, 2.005376344086022, 1.9354838709677424, 1.8333333333333341, 1.8709677419354847, 1.9130824372759863, 1.78405017921147, 1.6845878136200723, 1.6917562724014341, 1.6890681003584231, 1.5770609318996418, 1.5259856630824378, 1.541218637992832, 1.4327956989247317, 1.349462365591398, 1.3028673835125448, 1.257168458781362, 1.2939068100358428, 1.2813620071684593, 1.2795698924731187, 1.3010752688172051, 1.3073476702508968, 1.2535842293906816, 1.1066308243727598, 1.0152329749103939, 0.9883512544802864, 1.0430107526881716, 1.0949820788530462, 1.0286738351254476, 0.9059139784946235, 0.8870967741935485, 0.9130824372759857, 0.9130824372759857, 0.9229390681003584, 0.9032258064516128, 0.9229390681003582, 0.8557347670250894, 0.7813620071684588, 0.7768817204301075, 0.7249103942652327, 0.7105734767025088, 0.6657706093189963, 0.6738351254480286, 0.6639784946236558, 0.5707885304659497, 0.5734767025089604, 0.5788530465949819, 0.5483870967741935, 0.5134408602150536, 0.46505376344086, 0.41845878136200704, 0.46505376344086014, 0.5340501792114695, 0.5080645161290321, 0.4937275985663081, 0.4516129032258063, 0.45250896057347656, 0.4704301075268815, 0.41487455197132594, 0.3808243727598565, 0.3870967741935482, 0.4274193548387095, 0.38172043010752676, 0.364695340501792, 0.4238351254480285, 0.39247311827956965, 0.36021505376344054, 0.3637992831541216, 0.32258064516129015, 0.31630824372759847, 0.34677419354838696, 0.31182795698924715, 0.3046594982078852, 0.2921146953405017, 0.30734767025089593, 0.2706093189964157, 0.23028673835125452, 0.22759856630824377, 0.19892473118279574, 0.19175627240143372, 0.1989247311827957, 0.217741935483871, 0.19534050179211476, 0.18906810035842297, 0.2051971326164875, 0.18727598566308246, 0.16308243727598565, 0.15322580645161293, 0.11469534050179214, 0.11111111111111113, 0.1299283154121864, 0.10483870967741934, 0.1129032258064516, 0.13709677419354843, 0.13620071684587817, 0.13799283154121864, 0.057347670250896064, 0.010752688172043015, 0.031362007168458786, 0.018817204301075266, 0.03584229390681002, 0.05197132616487454, 0.06899641577060932, 0.07347670250896056, 0.049283154121863786, 0.041218637992831535, -0.008960573476702491, -0.01344086021505374, 0.03315412186379928, 0.03136200716845876, 0.002688172043010734, -0.00716845878136201, 0.010752688172043022]
  out "On-Line  Smoothed":dbl[](array[numeric])=[15041.73297491039, 14820.93637992831, 5793.450716845874, 57.05734767025088, 80.44892473118276, 102.59050179211462, 109.13261648745512, 111.17652329749097, 121.7974910394264, 138.88440860215047, 158.97759856630825, 178.95788530465956, 196.34498207885315, 208.3360215053765, 213.9202508960575, 215.2392473118281, 213.7275985663084, 211.7025089605736, 209.299283154122, 206.92204301075282, 203.59498207885315, 199.30286738351265, 195.41845878136212, 190.47580645161298, 184.99731182795705, 179.78046594982084, 173.5215053763441, 165.65412186379928, 156.7535842293907, 148.08154121863797, 140.37096774193543, 132.08512544802858, 123.48655913978487, 115.47759856630819, 108.49999999999994, 102.86111111111106, 97.36738351254475, 92.10394265232969, 87.41039426523292, 83.0833333333333, 78.95609318996414, 74.55734767025088, 70.35573476702507, 66.48387096774191, 62.466845878136155, 58.80555555555551, 55.67383512544799, 52.891577060931866, 50.1379928315412, 47.9722222222222, 46.687275985663064, 45.29121863799282, 43.188172043010745, 39.84587813620071, 36.14874551971327, 32.799283154121895, 29.8772401433692, 27.907706093189983, 26.48028673835127, 24.865591397849478, 23.474014336917577, 22.302867383512556, 20.90860215053764, 19.814516129032263, 19.493727598566316, 19.602150537634415, 20.138888888888896, 22.280465949820794, 23.911290322580655, 22.528673835125456, 20.959677419354847, 20.82526881720431, 20.802867383512552, 20.51702508960574, 20.125448028673844, 19.728494623655923, 18.788530465949826, 17.185483870967744, 15.744623655913987, 14.293010752688183, 12.600358422939074, 11.370967741935486, 10.53405017921147, 10.012544802867385, 9.411290322580644, 8.813620071684586, 8.27060931899641, 7.637992831541213, 7.2446236559139745, 6.912186379928311, 6.749103942652324, 6.626344086021501, 6.465949820788527, 6.2876344086021465, 6.079749103942648, 5.797491039426519, 5.568996415770605, 5.4596774193548345, 5.259856630824371, 5.288530465949819, 5.4865591397849425, 5.508960573476699, 5.155913978494622, 4.648745519713261, 4.489247311827956, 4.497311827956988, 4.365591397849462, 4.2517921146953395, 4.132616487455195, 4.448924731182794, 4.873655913978494, 4.3055555555555545, 3.5887096774193523, 3.3897849462365564, 3.3557347670250874, 3.2598566308243706, 3.134408602150536, 3.0528673835125435, 3.023297491039425, 2.9417562724014323, 2.836021505376343, 2.8127240143369163, 2.7329749103942644, 2.6496415770609314, 2.5412186379928317, 2.4847670250896057, 2.3342293906810037, 2.258064516129033, 2.3037634408602155, 2.268817204301076, 2.1747311827957, 2.112903225806453, 2.06451612903226, 2.0197132616487474, 2.0412186379928334, 1.9453405017921157, 1.8512544802867388, 1.7320788530465956, 1.6926523297491047, 1.7849462365591409, 1.742831541218639, 1.6164874551971335, 1.5922939068100366, 1.543010752688173, 1.4856630824372767, 1.4865591397849471, 1.5026881720430116, 1.455197132616488, 1.35573476702509, 1.370071684587814, 1.301971326164875, 1.2060931899641583, 1.2284946236559144, 1.1926523297491043, 1.120967741935484, 1.1173835125448033, 1.1030465949820791, 1.1218637992831542, 1.163978494623656, 1.1182795698924735, 0.9955197132616491, 0.9399641577060935, 0.9704301075268822, 0.9668458781362013, 0.9148745519713268, 0.8387096774193554, 0.7992831541218641, 0.8207885304659501, 0.8360215053763443, 0.8279569892473123, 0.7813620071684593, 0.7043010752688175, 0.6792114695340503, 0.7186379928315414, 0.6693548387096777, 0.6514336917562724, 0.6908602150537635, 0.6872759856630826, 0.6559139784946237, 0.6120071684587814, 0.6075268817204302, 0.6021505376344087, 0.6415770609318998, 0.6039426523297491, 0.5421146953405016, 0.5152329749103942, 0.5161290322580645, 0.5268817204301074, 0.5376344086021503, 0.49910394265232955, 0.4274193548387095, 0.450716845878136, 0.42473118279569877, 0.34498207885304644, 0.3951612903225804, 0.48028673835125424, 0.461469534050179, 0.4202508960573475, 0.33154121863799274, 0.3422939068100358, 0.37992831541218625, 0.34498207885304644, 0.3709677419354837, 0.368279569892473, 0.31720430107526876, 0.3306451612903225, 0.3189964157706093, 0.29749103942652333, 0.27508960573476693, 0.2732974910394264, 0.29659498207885304, 0.28763440860215056, 0.2553763440860215, 0.26254480286738346, 0.2598566308243727, 0.2284946236559139, 0.21505376344086014, 0.18279569892473108, 0.20788530465949812, 0.21774193548387083, 0.23476702508960562, 0.23566308243727585, 0.1648745519713261, 0.11469534050179216, 0.13082437275985664, 0.15232974910394265, 0.11738351254480285, 0.15322580645161288, 0.22401433691756267, 0.16397849462365593, 0.08870967741935488, 0.1308243727598566, 0.15232974910394265, 0.12186379928315418, 0.11648745519713263, 0.11917562724014343, 0.13172043010752688, 0.1254480286738351, 0.12813620071684595, 0.0931899641577061, 0.02419354838709676, 0.08960573476702503, 0.15232974910394262, 0.11200716845878138, 0.07616487455197132, 0.11469534050179206, 0.09767025089605731, 0.017025089605734768, -0.012544802867383516, 0.04928315412186375, 0.09946236559139779, 0.04749103942652328, 0.06093189964157706, 0.06630824372759857, 0.01523297491039426, -0.008960573476702517, 0.034050179211469564, 0.04480286738351258, 0.029569892473118278, 0.013440860215053774, 0.024193548387096787, 0.07437275985663085, 0.0313620071684588, 0.0, -0.010752688172042979, 0.00716845878136204, 0.025985663082437275, -0.053763440860215034, -0.06630824372759853, 2.949029909160572e-17, 0.037634408602150574, 0.017921146953405048, 0.01075268817204305, -0.01433691756272397, -0.00985663082437271, 0.028673835125448053, -0.005376344086021505]
  out "On-Line Bin Readings":dbl[](array[numeric])=[11947.0, 18291.0, 11768.0, 44.0, 47.0, 80.0, 72.0, 72.0, 95.0, 89.0, 112.0, 116.0, 139.0, 172.0, 174.0, 193.0, 170.0, 178.0, 164.0, 171.0, 184.0, 186.0, 189.0, 190.0, 172.0, 157.0, 159.0, 170.0, 163.0, 155.0, 130.0, 121.0, 125.0, 148.0, 130.0, 90.0, 82.0, 106.0, 74.0, 80.0, 86.0, 74.0, 94.0, 79.0, 73.0, 56.0, 49.0, 59.0, 45.0, 53.0, 49.0, 53.0, 42.0, 34.0, 26.0, 30.0, 25.0, 35.0, 27.0, 23.0, 21.0, 22.0, 29.0, 24.0, 22.0, 28.0, 16.0, 19.0, 25.0, 19.0, 14.0, 25.0, 20.0, 12.0, 19.0, 23.0, 23.0, 21.0, 19.0, 7.0, 12.0, 4.0, 15.0, 9.0, 8.0, 5.0, 14.0, 5.0, 8.0, 3.0, 5.0, 7.0, 3.0, 5.0, 2.0, 9.0, 4.0, 4.0, 4.0, 1.0, 7.0, 12.0, 12.0, 6.0, 6.0, 9.0, 12.0, 6.0, 7.0, 4.0, 12.0, 9.0, 7.0, 6.0, 5.0, 2.0, 5.0, 7.0, 7.0, 2.0, 2.0, 0.0, 8.0, 4.0, 3.0, 3.0, 2.0, 5.0, 3.0, 5.0, 1.0, 1.0, 4.0, 3.0, 6.0, 3.0, 1.0, 7.0, 1.0, 4.0, 3.0, 1.0, 4.0, 4.0, 3.0, 4.0, 3.0, 4.0, 3.0, 5.0, 1.0, 1.0, 2.0, 2.0, 3.0, 0.0, 1.0, 2.0, 0.0, 4.0, 5.0, 2.0, 3.0, 4.0, 1.0, 1.0, 2.0, 4.0, 1.0, 1.0, 1.0, 0.0, 0.0, 2.0, 0.0, 3.0, 1.0, 3.0, 2.0, 1.0, 0.0, 2.0, 0.0, 2.0, 2.0, 2.0, 2.0, 1.0, 1.0, 4.0, 2.0, 3.0, 1.0, 1.0, 0.0, 0.0, 0.0, 3.0, 1.0, 1.0, 1.0, 2.0, 1.0, 1.0, 1.0, 0.0, 1.0, 3.0, 1.0, 4.0, 5.0, 0.0, 2.0, 3.0, 2.0, 0.0, 4.0, 1.0, 1.0, 1.0, 1.0, 2.0, 2.0, 2.0, 0.0, 1.0, 1.0, 2.0, 2.0, 0.0, 4.0, 4.0, 0.0, 2.0, 0.0, 1.0, 0.0, 0.0, 0.0, 1.0, 0.0, 0.0, 0.0, 0.0, 1.0, 0.0, 1.0, 2.0, 0.0, 3.0, 0.0, 2.0, 0.0, 0.0, 1.0, 0.0, 1.0, 1.0, 1.0, 0.0, 0.0, 1.0, 5.0, 0.0, 0.0, 0.0, 0.0, 0.0, 1.0, 2.0, 0.0, 2.0, 1.0, 1.0, 2.0, 0.0, 1.0, 0.0, 0.0]
  out "Range Corrected Altitude Array":dbl[](array[numeric])=[5625.0, 22500.0, 50625.0, 90000.0, 140625.0, 202500.0, 275625.0, 360000.0, 455625.0, 562500.0, 680625.0, 810000.0, 950625.0, 1102500.0, 1265625.0, 1440000.0, 1625625.0, 1822500.0, 2030625.0, 2250000.0, 2480625.0, 2722500.0, 2975625.0, 3240000.0, 3515625.0, 3802500.0, 4100625.0, 4410000.0, 4730625.0, 5062500.0, 5405625.0, 5760000.0, 6125625.0, 6502500.0, 6890625.0, 7290000.0, 7700625.0, 8122500.0, 8555625.0, 9000000.0, 9455625.0, 9922500.0, 10400625.0, 10890000.0, 11390625.0, 11902500.0, 12425625.0, 12960000.0, 13505625.0, 14062500.0, 14630625.0, 15210000.0, 15800625.0, 16402500.0, 17015625.0, 17640000.0, 18275625.0, 18922500.0, 19580625.0, 20250000.0, 20930625.0, 21622500.0, 22325625.0, 23040000.0, 23765625.0, 24502500.0, 25250625.0, 26010000.0, 26780625.0, 27562500.0, 28355625.0, 29160000.0, 29975625.0, 30802500.0, 31640625.0, 32490000.0, 33350625.0, 34222500.0, 35105625.0, 36000000.0, 36905625.0, 37822500.0, 38750625.0, 39690000.0, 40640625.0, 41602500.0, 42575625.0, 43560000.0, 44555625.0, 45562500.0, 46580625.0, 47610000.0, 48650625.0, 49702500.0, 50765625.0, 51840000.0, 52925625.0, 54022500.0, 55130625.0, 56250000.0, 57380625.0, 58522500.0, 59675625.0, 60840000.0, 62015625.0, 63202500.0, 64400625.0, 65610000.0, 66830625.0, 68062500.0, 69305625.0, 70560000.0, 71825625.0, 73102500.0, 74390625.0, 75690000.0, 77000625.0, 78322500.0, 79655625.0, 81000000.0, 82355625.0, 83722500.0, 85100625.0, 86490000.0, 87890625.0, 89302500.0, 90725625.0, 92160000.0, 93605625.0, 95062500.0, 96530625.0, 98010000.0, 99500625.0, 101002500.0, 102515625.0, 104040000.0, 105575625.0, 107122500.0, 108680625.0, 110250000.0, 111830625.0, 113422500.0, 115025625.0, 116640000.0, 118265625.0, 119902500.0, 121550625.0, 123210000.0, 124880625.0, 126562500.0, 128255625.0, 129960000.0, 131675625.0, 133402500.0, 135140625.0, 136890000.0, 138650625.0, 140422500.0, 142205625.0, 144000000.0, 145805625.0, 147622500.0, 149450625.0, 151290000.0, 153140625.0, 155002500.0, 156875625.0, 158760000.0, 160655625.0, 162562500.0, 164480625.0, 166410000.0, 168350625.0, 170302500.0, 172265625.0, 174240000.0, 176225625.0, 178222500.0, 180230625.0, 182250000.0, 184280625.0, 186322500.0, 188375625.0, 190440000.0, 192515625.0, 194602500.0, 196700625.0, 198810000.0, 200930625.0, 203062500.0, 205205625.0, 207360000.0, 209525625.0, 211702500.0, 213890625.0, 216090000.0, 218300625.0, 220522500.0, 222755625.0, 225000000.0, 227255625.0, 229522500.0, 231800625.0, 234090000.0, 236390625.0, 238702500.0, 241025625.0, 243360000.0, 245705625.0, 248062500.0, 250430625.0, 252810000.0, 255200625.0, 257602500.0, 260015625.0, 262440000.0, 264875625.0, 267322500.0, 269780625.0, 272250000.0, 274730625.0, 277222500.0, 279725625.0, 282240000.0, 284765625.0, 287302500.0, 289850625.0, 292410000.0, 294980625.0, 297562500.0, 300155625.0, 302760000.0, 305375625.0, 308002500.0, 310640625.0, 313290000.0, 315950625.0, 318622500.0, 321305625.0, 324000000.0, 326705625.0, 329422500.0, 332150625.0, 334890000.0, 337640625.0, 340402500.0, 343175625.0, 345960000.0, 348755625.0, 351562500.0, 354380625.0, 357210000.0, 360050625.0, 362902500.0, 365765625.0, 368640000.0, 371525625.0, 374422500.0, 377330625.0, 380250000.0, 383180625.0, 386122500.0, 389075625.0, 392040000.0, 395015625.0, 398002500.0, 401000625.0, 404010000.0, 407030625.0, 410062500.0, 413105625.0, 416160000.0, 419225625.0, 422302500.0, 425390625.0, 428490000.0, 431600625.0, 434722500.0, 437855625.0, 441000000.0]
  out "Altitude Array (km)":dbl[](array[numeric])=[0.075, 0.15, 0.22499999999999998, 0.3, 0.375, 0.45, 0.5249999999999999, 0.6, 0.6749999999999999, 0.7499999999999999, 0.825, 0.8999999999999999, 0.9749999999999999, 1.05, 1.125, 1.2, 1.275, 1.3499999999999999, 1.4249999999999998, 1.5, 1.575, 1.65, 1.7249999999999999, 1.7999999999999998, 1.8749999999999998, 1.95, 2.025, 2.1, 2.1750000000000003, 2.25, 2.325, 2.4, 2.475, 2.5500000000000003, 2.625, 2.7, 2.775, 2.85, 2.9250000000000003, 3.0, 3.075, 3.15, 3.225, 3.3000000000000003, 3.375, 3.45, 3.525, 3.6, 3.675, 3.75, 3.825, 3.9, 3.975, 4.05, 4.125, 4.2, 4.275, 4.35, 4.425, 4.5, 4.575, 4.65, 4.725, 4.8, 4.875, 4.95, 5.025, 5.1, 5.175, 5.25, 5.325, 5.4, 5.475, 5.55, 5.625, 5.7, 5.775, 5.85, 5.925, 6.0, 6.075, 6.15, 6.225, 6.3, 6.375, 6.45, 6.525, 6.6, 6.675, 6.75, 6.825, 6.9, 6.975, 7.05, 7.125, 7.2, 7.2749999999999995, 7.35, 7.425, 7.5, 7.575, 7.6499999999999995, 7.725, 7.8, 7.875, 7.95, 8.024999999999999, 8.1, 8.174999999999999, 8.249999999999998, 8.325, 8.399999999999999, 8.475, 8.549999999999999, 8.624999999999998, 8.7, 8.774999999999999, 8.85, 8.924999999999999, 8.999999999999998, 9.075, 9.149999999999999, 9.225, 9.299999999999999, 9.374999999999998, 9.45, 9.524999999999999, 9.6, 9.674999999999999, 9.749999999999998, 9.825, 9.899999999999999, 9.975, 10.049999999999999, 10.124999999999998, 10.2, 10.274999999999999, 10.35, 10.424999999999999, 10.499999999999998, 10.575, 10.649999999999999, 10.725, 10.799999999999999, 10.874999999999998, 10.95, 11.024999999999999, 11.1, 11.174999999999999, 11.249999999999998, 11.325, 11.399999999999999, 11.475, 11.549999999999999, 11.624999999999998, 11.7, 11.774999999999999, 11.85, 11.924999999999999, 11.999999999999998, 12.075, 12.149999999999999, 12.225, 12.299999999999999, 12.374999999999998, 12.45, 12.524999999999999, 12.6, 12.674999999999999, 12.749999999999998, 12.825, 12.899999999999999, 12.975, 13.049999999999999, 13.124999999999998, 13.2, 13.274999999999999, 13.35, 13.424999999999999, 13.499999999999998, 13.575, 13.649999999999999, 13.725, 13.799999999999999, 13.874999999999998, 13.95, 14.024999999999999, 14.1, 14.174999999999999, 14.249999999999998, 14.325, 14.399999999999999, 14.474999999999998, 14.549999999999999, 14.624999999999998, 14.7, 14.774999999999999, 14.849999999999998, 14.924999999999999, 14.999999999999998, 15.075, 15.149999999999999, 15.224999999999998, 15.299999999999999, 15.374999999999998, 15.45, 15.524999999999999, 15.599999999999998, 15.674999999999999, 15.749999999999998, 15.825, 15.899999999999999, 15.974999999999998, 16.05, 16.125, 16.2, 16.275, 16.349999999999998, 16.424999999999997, 16.5, 16.575, 16.65, 16.724999999999998, 16.799999999999997, 16.875, 16.95, 17.025, 17.099999999999998, 17.174999999999997, 17.25, 17.325, 17.4, 17.474999999999998, 17.549999999999997, 17.625, 17.7, 17.775, 17.849999999999998, 17.924999999999997, 18.0, 18.075, 18.15, 18.224999999999998, 18.299999999999997, 18.375, 18.45, 18.525, 18.599999999999998, 18.674999999999997, 18.75, 18.825, 18.9, 18.974999999999998, 19.049999999999997, 19.125, 19.2, 19.275, 19.349999999999998, 19.424999999999997, 19.5, 19.575, 19.65, 19.724999999999998, 19.799999999999997, 19.875, 19.95, 20.025, 20.099999999999998, 20.174999999999997, 20.25, 20.325, 20.4, 20.474999999999998, 20.549999999999997, 20.625, 20.7, 20.775, 20.849999999999998, 20.924999999999997, 21.0]
  out "Offline Pulse Energy":dbl
  out "Online Pulse Energy":dbl
  in  "Instrument Control":T5(tab)
  out "Readings":T6={"OnLineTEC"=19.6930485, "OnLineLD"=0.141470715, "OffLineTEC"=17.3787479, "OffLineLD"=0.145009771, "EtalonTEC"=25.2519455, "TSOA-TEC"=18.0371037, "Pro8000"=TRUE, "OnLine TEC"=TRUE, "OnLine LD"=TRUE, "OffLine TEC"=TRUE, "OffLine LD"=TRUE, "Etalon TEC"=TRUE, "TSOA TEC"=TRUE} {"OffLineLD" format="%.4g"; "OnLineLD" format="%.4g"; "TSOA-TEC" format="%.3g"; "EtalonTEC" format="%.3g"; "OffLineTEC" format="%.3g"; "OnLineTEC" format="%.3g"}
  in  "Settings":T7={"Module"=enum."Off Line LD", "OnLineTEC"=19.69, "OnLineLD"=0.14128899999999628, "OffLineTEC"=17.38, "OffLineLD"=0.14529099999999728, "EtalonTEC"=25.5, "TSOA-TEC"=18.0} {"OffLineLD" min=0.0 max=0.175 step=0.001 format="%.3p"; "OnLineLD" min=0.0 max=0.175 step=0.001 format="%.3p"; "TSOA-TEC" format="%.2g"; "EtalonTEC" format="%.2g"; "OffLineTEC" min=0.0 max=30.0 step=0.1 format="%.2g"; "OnLineTEC" min=0.0 max=30.0 step=0.1 format="%.2g"}
  in  "Pulse B Polarity":enum32{"Low", "High"}(ring)=enum."High"
  in  "Pulse A Delay(ns)":u32=1040 min=80 max=327600
  in  "Pulse B Delay(ns)":u32=170000 min=80 max=327600 step=1
  in  "Accumulation Delay(ns)":u32=10 min=10 max=1270 step=1
  in  "Sync Pulse Polarity":enum32{"Low", "High"}(ring)=enum."High"
  in  "Pulse A Polarity":enum32{"Low", "High"}(ring)=enum."High"
  in  "Number of Bins":u32=280 min=2 max=4095 step=1
  in  "Number of Accumulates":u32=10000 min=1 max=32767 step=1
  in  "Time Resolution Per Bin(ns)":u32=500 min=5 max=1063 step=1
  in  "Cancel online":bool
  in  "Cancel Offline":bool
  in  "Lambda On Set (nm)":dbl=828.191 format="%.5f"
  out "Lambda On Read (nm)":dbl=828.1909839042386 format="%.5f"
  out "Lambda Off Read (nm)":dbl=828.2904566874113 format="%.5f"
  in  "Lambda Off Set (nm)":dbl=828.29045 format="%#.5f"
  in  "Bristol In":i32=5
  out "Bristol Out":i32=27
  in  "AB_DIF":dbl=5e-05 format="%#_15g"
  in  "NONAB_DIF":dbl=5e-05 format="%#_15g"
  out "Wavelength Lock Online":bool=TRUE
  out "Wavelength Lock Offline":bool=TRUE
  out "WL Difference":dbl=-1.609576145256142e-05 format="%_7g"
  out "WL Difference off":dbl=6.68741131448769e-06 format="%_7g"
  in  "calculate absorption cross sections":bool
  in  "Smoothing Range":dbl=150.0
  in  "Total DIAL Integration Time (Minutes)":i32=4
  in  "Data Reads (number of loops)":i32=1
  in  "Total Aerosol Integration Time (Minutes)":dbl=0.05
  in  "Scalar Wait Time":u32=1400
  out "Smoothed Bins":dbl=2.0
  in  "NewportIn":string
  in  "logging":bool
  out "Newport Device Key":string
  in  "SampleSize":i32=2
  out "NewportRef":refnum<k24>
  in  "Switch Comm Port":refnum<visa-resource-name>="COM3"
  out "FF_On_Ref":refnum<file>
  out "FF_On_Ptr":i64=700128 format="%.2p"
  out "FF_Off_Ref":refnum<file>
  out "FF_Off_Ptr":i64=700128 format="%.2p"
  out "NF_On_Ref":refnum<file>
  out "NF_On_Ptr":i64=700128 format="%.2p"
  out "NF_Off_Ref":refnum<file>
  out "NF_Off_Ptr":i64=700128 format="%.2p"
  out "DataOpen":bool=TRUE
  out "File Path_Far Field (out)":string="D:\\Micropulse_DIAL_data\\151218FF\\01"
  out "File Path_Near Field (out)":string="D:\\Micropulse_DIAL_data\\151218NF\\01"
  in  "Data File DIR (in)":string="D:\\Micropulse_DIAL_data\\"
  in  "bins":u32=280 min=2 max=4095 step=1
  out "y offset":u32=10
  in  "ns scale":u32=500
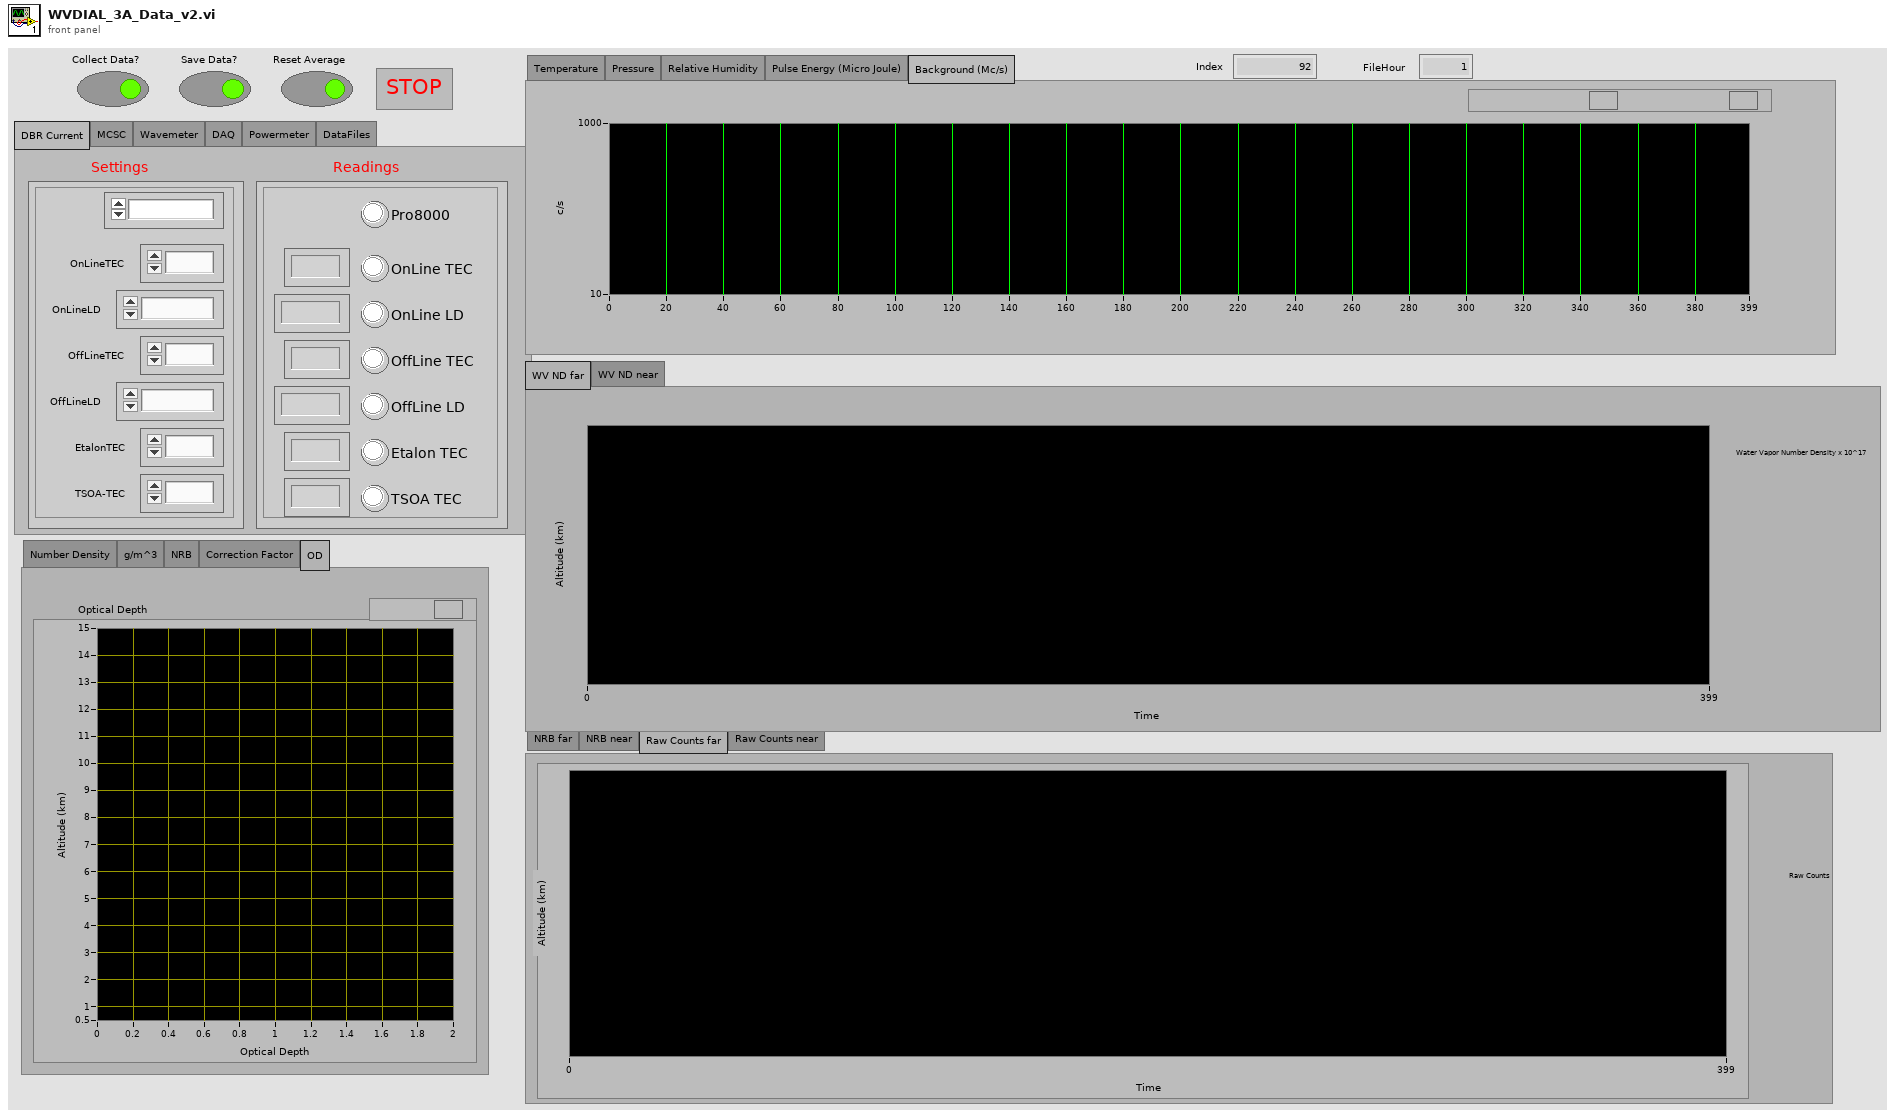
[diagram p1: front panel]
types:
  T1 = enum32{"NRB far", "NRB near", "Raw Counts far", "Raw Counts near"}
  T2 = enum32{"Number Density", "g/m^3", "NRB", "Correction Factor", "OD"}
  T3 = enum32{"Temperature", "Pressure", "Relative Humidity", "Pulse Energy (Micro Joule)", "Background (Mc/s)"}
  T4 = cluster{"Online Pulse Energy":dbl, "Pulse Energy Offline":dbl}
  T5 = enum32{"DBR Current", "MCSC", "Wavemeter", "DAQ", "Powermeter", "DataFiles"}
  T6 = cluster{"OnLineTEC":dbl, "OnLineLD":dbl, "OffLineTEC":dbl, "OffLineLD":dbl, "EtalonTEC":dbl, "TSOA-TEC":dbl, "Pro8000":bool, "OnLine TEC":bool, "OnLine LD":bool, "OffLine TEC":bool, "OffLine LD":bool, "Etalon TEC":bool, "TSOA TEC":bool}
  T7 = cluster{"Module":enum16{"On Line TEC", "On Line LD", "Off Line TEC", "Off Line LD", "Etalon TEC", "TSOA TEC"}, "OnLineTEC":dbl, "OnLineLD":dbl, "OffLineTEC":dbl, "OffLineLD":dbl, "EtalonTEC":dbl, "TSOA-TEC":dbl}
  T8 = enum16{"Open_TL", "Close_TL", "Verify_ID", "TEC_Sensor", "SET", "READ", "ON", "OFF", "Set_Limits", "Read_Limits", "Enable_Status", "Read_Status"}
  T9 = enum16{"Initialize ILX", "Set ON T", "Set Off T", "Set ON I", "Set Off I", "Set On Lim", "Set Off Lim", "Read ILX", "TEC ON/OFF", "LASER ON/OFF", "Status?", "ILX OFF"}
  T10 = enum16{"open", "replace", "create", "open or create", "replace or create", "replace or create with confirmation"}
  T11 = enum16{"On Line TEC", "On Line LD", "Off Line TEC", "Off Line LD", "Etalon TEC", "TSOA TEC"}
  T12 = typedef "LVDateTimeRec.ctl" = cluster{"fractional second":dbl, "second":i32, "minute":i32, "hour":i32, "day of month":i32, "month":i32, "year":i32, "day of week":i32, "day of year":i32, "DST":i32}
  T13 = cluster{"Online Pulse Energy":dbl, "Offline Pulse Energy":dbl}
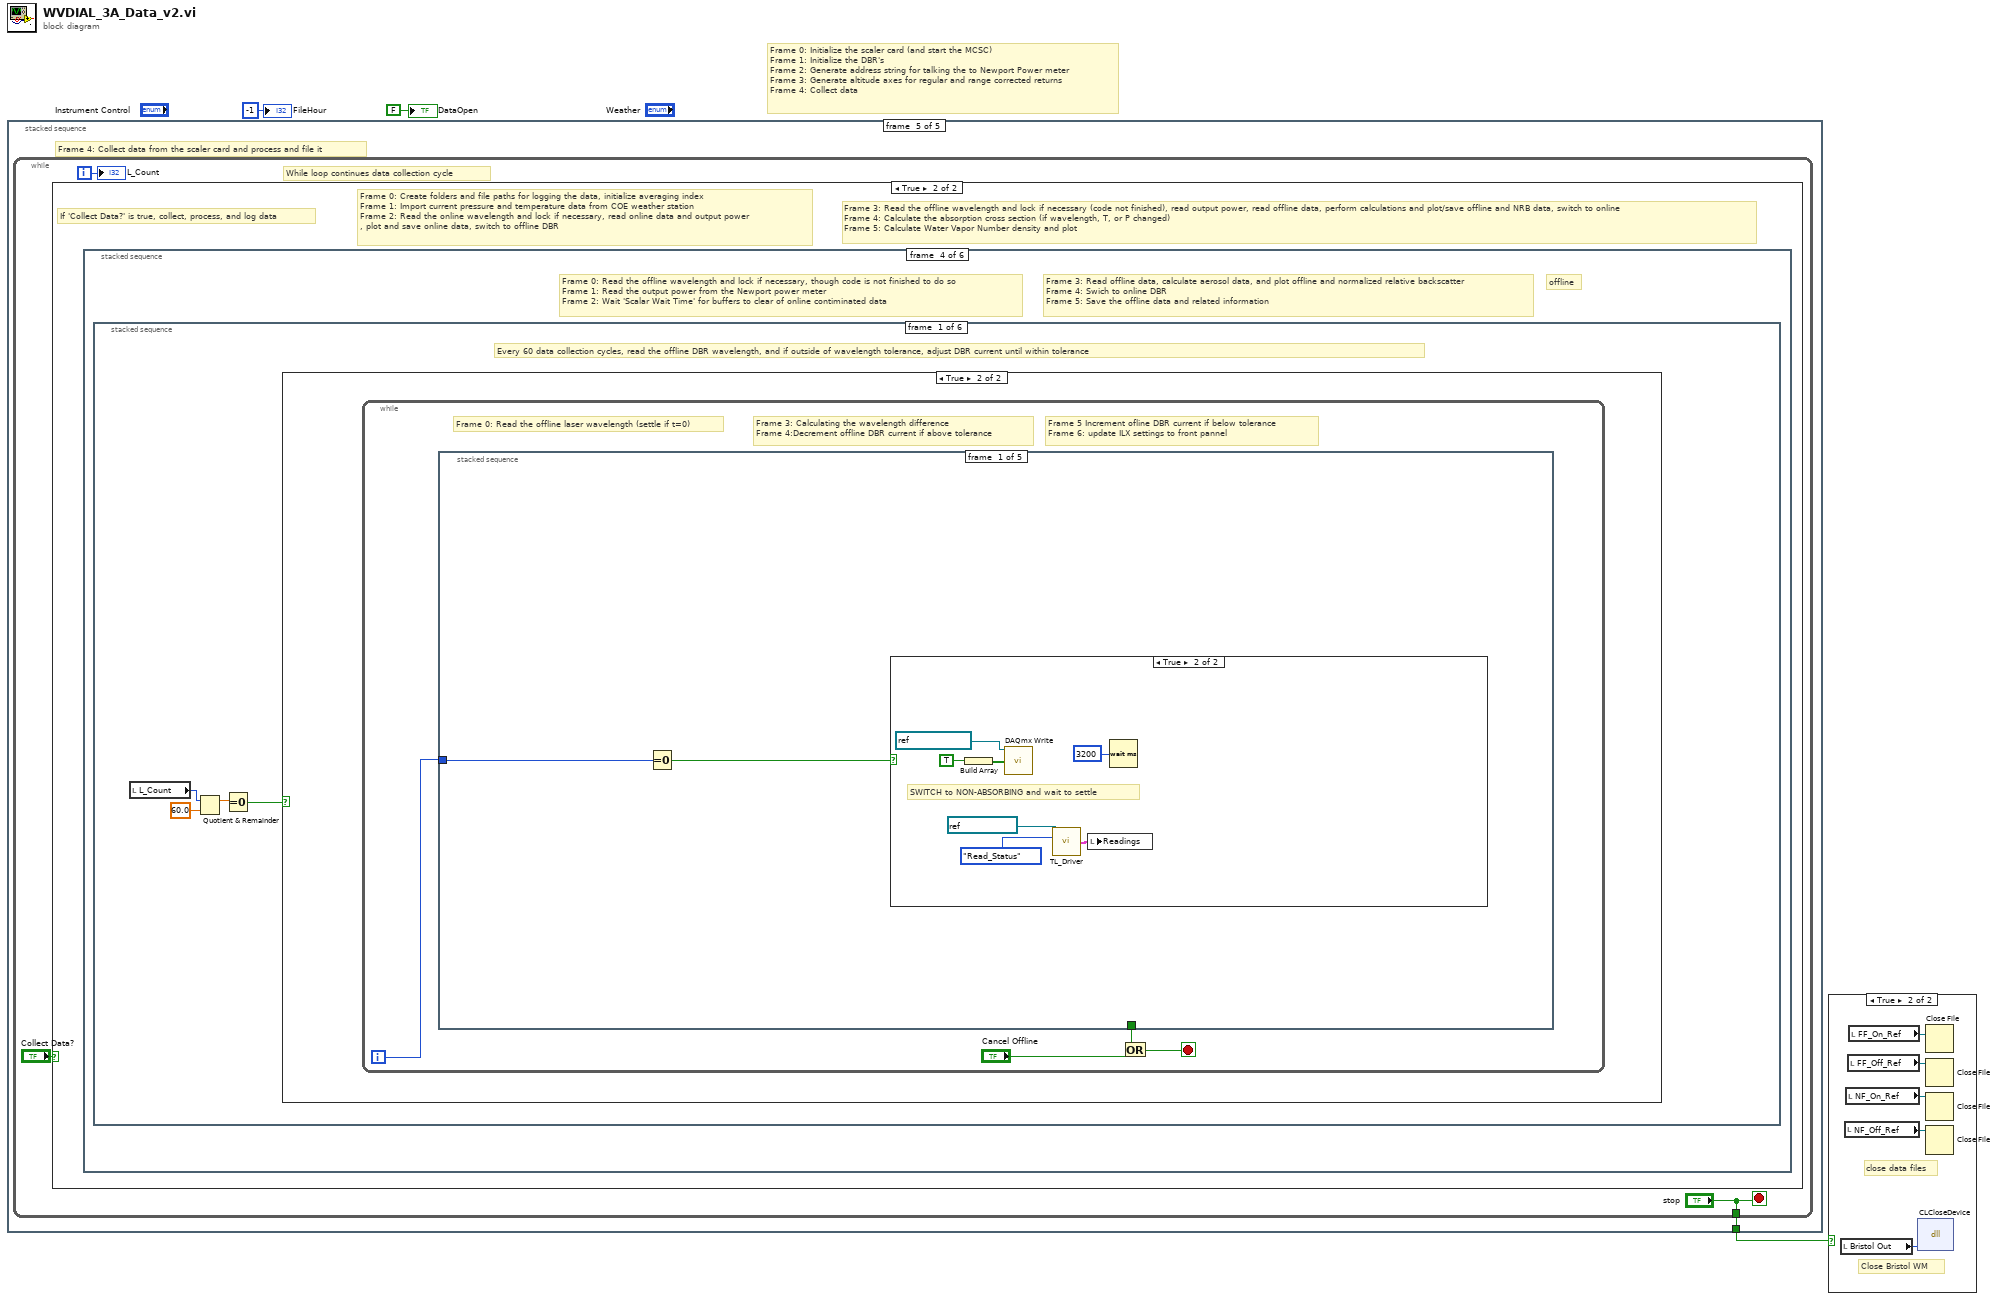
[diagram p0: block diagram]
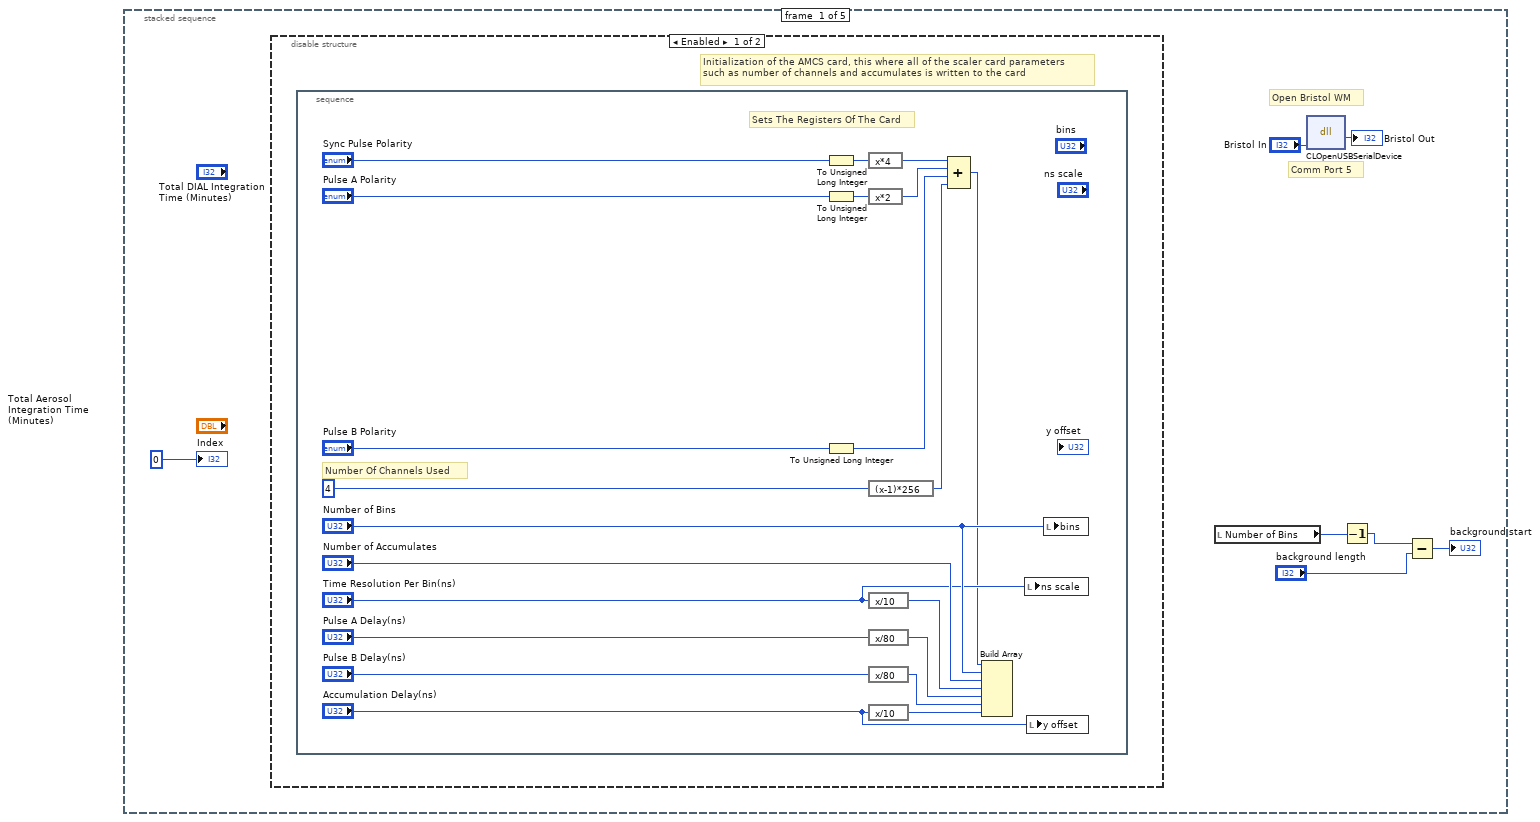
[diagram p3: hidden frame]
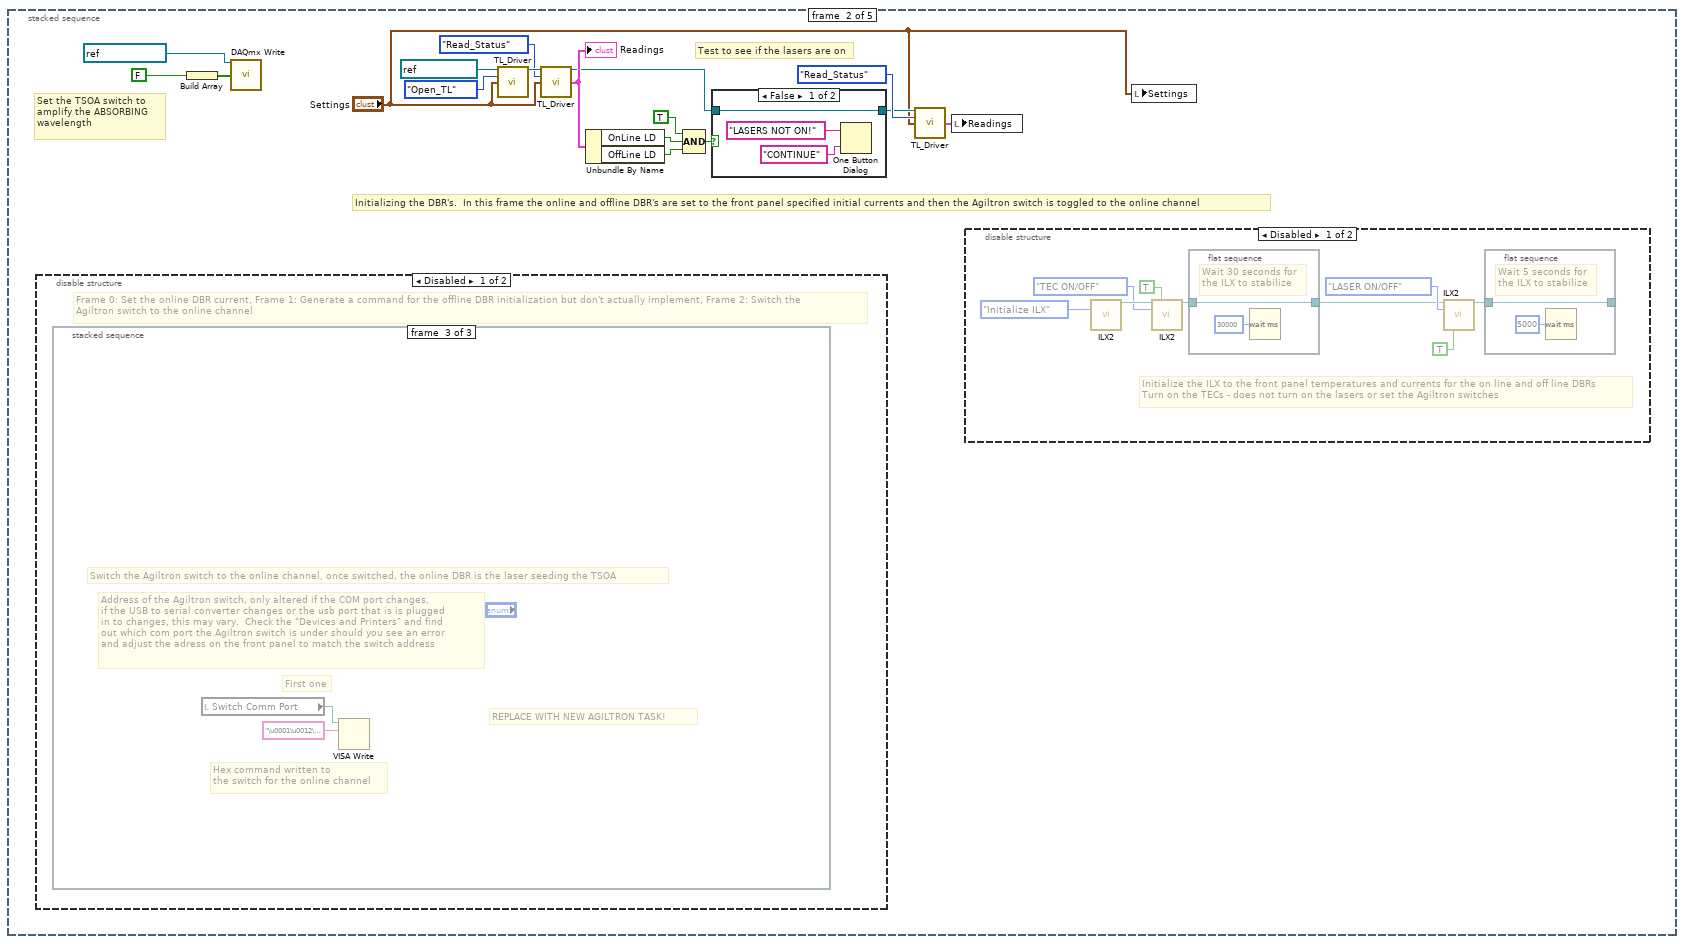
[diagram p5: hidden frame]
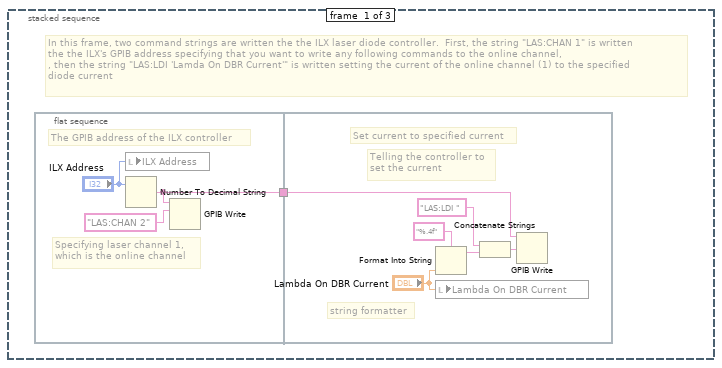
[diagram p8: hidden frame]
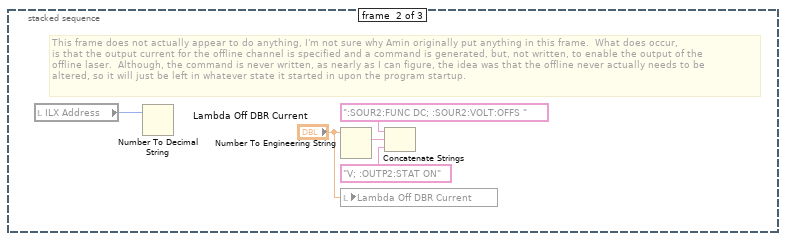
[diagram p9: hidden frame]
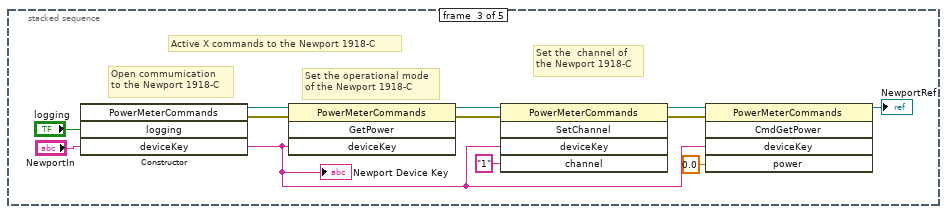
[diagram p11: hidden frame]
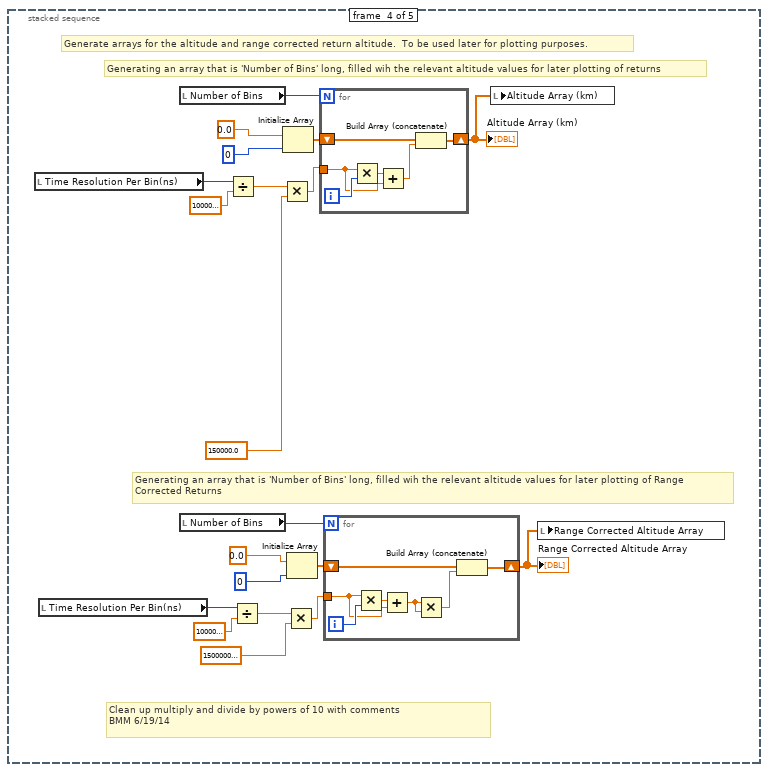
[diagram p12: hidden frame]
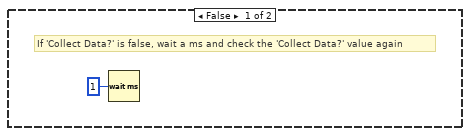
[diagram p13: hidden frame]
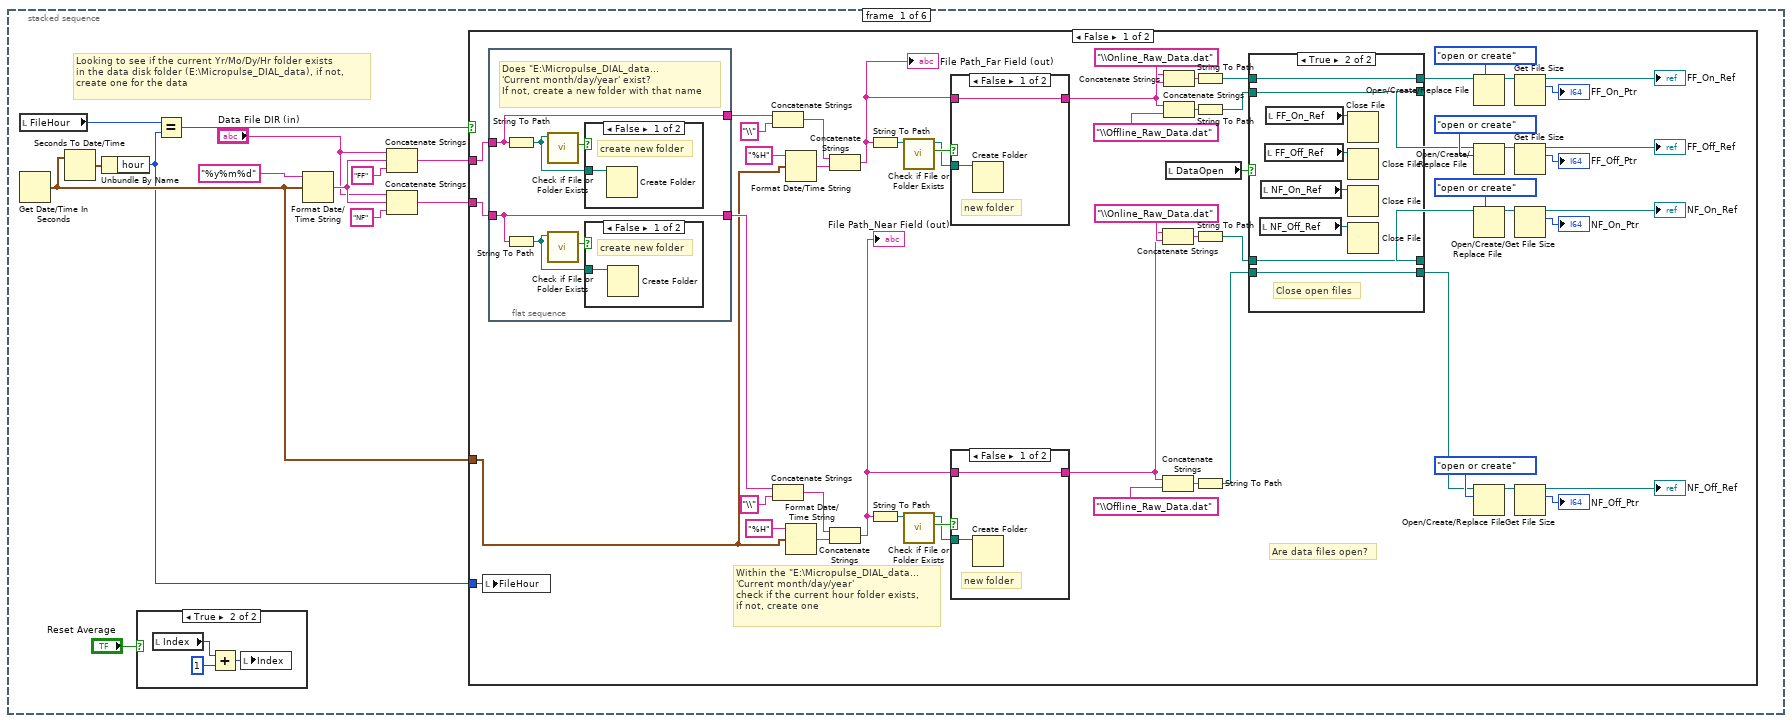
[diagram p14: hidden frame]
diagram:
  # "Frame 0: Initialize the scaler card (and start the MCSC)\nFrame 1: Initialize the DBR's\nFrame 2: Generate address string for talking the to Newport Power meter\nFrame 3: Generate altitude axes for regular and range corrected returns\nFrame 4: Collect data"
  n1 = stacked-sequence {
    tunnel: [_ _ _ _ w128] -> w3
    frame #0 {
      # "Comm Port 5"
      # "Open Bristol WM"
      n2 = disable-structure shown="Enabled" {
        frame Enabled {
          # "Initialization of the AMCS card, this where all of the scaler card parameters\nsuch as number of channels and accumulates is written to the card"
          n3 = stacked-sequence {
            frame #0 {
              # "Sets The Registers Of The Card"
              # "Number Of Channels Used"
              n4 = To Unsigned Long Integer(number="Sync Pulse Polarity") -> (unsigned 32bit integer=w11:u32)
              n5 = To Unsigned Long Integer(number="Pulse A Polarity") -> (unsigned 32bit integer=w15:u32)
              n6 = To Unsigned Long Integer(number="Pulse B Polarity") -> (unsigned 32bit integer=w13:u32)
              n7 = expression code="x*4"(w11) -> (w20:u32)
              n8 = expression code="x*2"(w15) -> (w19:u32)
              n9 = expression code="(x-1)*256"(u32 4 ("Number of Channels Used")) -> (w18:u32)
              n10 = expression code="x/10"("Time Resolution Per Bin(ns)") -> (w22:u32)
              n11 = expression code="x/80"("Pulse A Delay(ns)") -> (w29:u32)
              n12 = expression code="x/80"("Pulse B Delay(ns)") -> (w31:u32)
              n13 = expression code="x/10"("Accumulation Delay(ns)") -> (w30:u32)
              n14 = Compound Arithmetic op=ADD(w20, w19, w13, w18) -> (w17:u32)
              n15 = Build Array(w17, "Number of Bins", "Number of Accumulates", w22, w29, w31, w30) -> ()  [unwired: 1 out]
              n16 = local write "ns scale"("Time Resolution Per Bin(ns)") -> ()
              n17 = local write "y offset"("Accumulation Delay(ns)") -> ()
              n18 = local write "bins"("Number of Bins") -> ()
            }
          }
        }
        frame Disabled {
        }
      }
      n19 = local read "Number of Bins"() -> (w7:u32)
      n20 = dll-call lib="C:/H2O_DIAL/LabVIEW-2012/Bristol WM V2_31b/CLDevIface.dll" fn="CLOpenUSBSerialDevice"("commPort"="Bristol In") -> ("return type"=→"Bristol Out":i32)  [unwired: 4 in, 2 out]
      n21 = Decrement(x=w7) -> (x-1=w6:u32)
      n22 = Subtract(x=w6, y="background length") -> (x-y=→"background start":u32)
      "Index" <- 0 ("Index")
    }
    frame #1 {
      # "Test to see if the lasers are on"
      # "Set the TSOA switch to\namplify the ABSORBING\nwavelength"
      # "Initializing the DBR's.  In this frame the online and offline DBR's are set to the front panel specified initial currents and then the Agiltron switch is toggled to the online channel"
      n23 = disable-structure shown="Disabled" {
        frame Disabled {
          # "Frame 0: Set the online DBR current, Frame 1: Generate a command for the offline DBR initialization but don't actually implement, Frame 2: Switch the \nAgiltron switch to the online channel"
          n24 = stacked-sequence {
            frame #0 {
              # "In this frame, two command strings are written the the ILX laser diode controller.  First, the string \"LAS:CHAN 1\" is written\nthe the ILX's GPIB address specifying that you want to write any following commands to the online channel,\n, then the string \"LAS:LDI 'Lamda On DBR Current'\" is written setting the current of the online channel (1) to the specified \ndiode current"
              n25 = flat-sequence {
                tunnel: [w68] -> w66
                tunnel: w66 -> [w70]
                frame #0 {
                  # "The GPIB address of the ILX controller"
                  # "Specifying laser channel 1,\nwhich is the online channel"
                  n26 = local write "ILX Address"("ILX Address") -> ()
                  n27 = Number To Decimal String(number="ILX Address") -> (decimal integer string=w68:string)  [unwired: 1 in]
                  n28 = GPIB Write(0:w68, 1:"LAS:CHAN 2") -> ()  [unwired: 3 in, 2 out]
                }
                frame #1 {
                  # "Telling the controller to\nset the current"
                  # "string formatter"
                  # "Set current to specified current"
                  n29 = Format Into String(format string="%.4f" ("Format String"), "Lambda On DBR Current") -> (resulting string=w73:string)  [unwired: 2 in, 1 out]
                  n30 = local write "Lambda On DBR Current"("Lambda On DBR Current") -> ()
                  n31 = Concatenate Strings("LAS:LDI ", w73) -> (w74:string)
                  n32 = GPIB Write(0:w70, 1:w74) -> ()  [unwired: 3 in, 2 out]
                }
              }
            }
            frame #1 {
              # "This frame does not actually appear to do anything, I'm not sure why Amin originally put anything in this frame.  What does occur, \nis that the output current for the offline channel is specified and a command is generated, but, not written, to enable the output of the\noffline laser.  Although, the command is never written, as nearly as I can figure, the idea was that the offline never actually needs to be \naltered, so it will just be left in whatever state it started in upon the program startup."
              n33 = local read "ILX Address"() -> (w76:i32)
              n34 = Number To Decimal String(number=w76) -> ()  [unwired: 1 in, 1 out]
              n35 = Number To Engineering String(4:"Lambda Off DBR Current") -> (0:w80:string)  [unwired: 3 in]
              n36 = local write "Lambda Off DBR Current"("Lambda Off DBR Current") -> ()
              n37 = Concatenate Strings(":SOUR2:FUNC DC; :SOUR2:VOLT:OFFS ", w80, "V; :OUTP2:STAT ON") -> ()  [unwired: 1 out]
            }
            frame #2 {
              # "REPLACE WITH NEW AGILTRON TASK!"
              # "First one"
              # "Address of the Agiltron switch, only altered if the COM port changes,\nif the USB to serial converter changes or the usb port that is is plugged\nin to changes, this may vary.  Check the \"Devices and Printers\" and find \nout which com port the Agiltron switch is under should you see an error \nand adjust the adress on the front panel to match the switch address"
              # "Hex command written to \nthe switch for the online channel"
              # "Switch the Agiltron switch to the online channel, once switched, the online DBR is the laser seeding the TSOA"
              n38 = local read "Switch Comm Port"() -> (w81:refnum<visa-resource-name>)
              n39 = VISA Write(VISA resource name=w81, write buffer="\u0001\u0012\u0000\u0002") -> ()  [unwired: 1 in, 3 out]
            }
          }
        }
        frame Enabled {
        }
      }
      n40 = Build Array(FALSE ("Boolean")) -> (w33:bool[])
      n41 = call-poly <vilib>:"DAQmx Write.vi"("task/channels in"=refnum<k21> "BristolWM", "data"=w33) -> ()  [unwired: 11 in, 3 out]
      n42 = call "TL_Driver.vi"("Device In"=refnum<visa-resource-name> "ThorLabs", "Commands"=T8."Open_TL", "Settings"="Settings") -> ("Device Out"=w46:refnum<visa-resource-name>)  [unwired: 9 in, 3 out]
      n43 = call "TL_Driver.vi"("Device In"=w46, "Commands"=T8."Read_Status", "Settings"="Settings") -> ("Device Out"=w43:refnum<visa-resource-name>, "Readings"=w44:T6)  [unwired: 9 in, 2 out]
      "Readings" <- w44
      n44 = Unbundle By Name(w44) -> ("OnLine LD"=w38:bool, "OffLine LD"=w39:bool)
      n45 = Compound Arithmetic op=AND(TRUE, w38, w39) -> (w37:bool)
      n46 = case shown="False" w37 {
        tunnel: w43 -> [w49 w52]
        tunnel: [w49 w52] -> w41
        frame False {
          n47 = One Button Dialog(message="LASERS NOT ON!", button name ("OK")="CONTINUE") -> ()  [unwired: 1 out]
        }
        frame True {
        }
      }
      n48 = call "TL_Driver.vi"("Device In"=w41, "Commands"=T8."Read_Status", "Settings"="Settings") -> ("Readings"=w32:T6)  [unwired: 9 in, 3 out]
      n49 = local write "Readings"(w32) -> ()
      n50 = disable-structure shown="Disabled" {
        frame Disabled {
          # "Initialize the ILX to the front panel temperatures and currents for the on line and off line DBRs\nTurn on the TECs - does not turn on the lasers or set the Agiltron switches"
          n51 = call "ILX2.vi"("ILX Command"=T9."Initialize ILX") -> ("Device Out"=w60:refnum<visa-resource-name>)  [unwired: 10 in, 4 out]
          n52 = call "ILX2.vi"("Device In"=w60, "TEC Control"=TRUE, "ILX Command"=T9."TEC ON/OFF") -> ("Device Out"=w57:refnum<visa-resource-name>)  [unwired: 8 in, 4 out]
          n53 = flat-sequence {
            tunnel: w57 -> [w64]
            tunnel: [w64] -> w54
            frame #0 {
              # "Wait 30 seconds for\nthe ILX to stabilize"
              n54 = Wait (ms)(milliseconds to wait=u32 30000) -> ()  [unwired: 1 out]
            }
          }
          n55 = call "ILX2.vi"("Device In"=w54, "ILX Command"=T9."LASER ON/OFF", "Laser Control"=TRUE ("TEC Control")) -> ("Device Out"=w53:refnum<visa-resource-name>)  [unwired: 8 in, 4 out]
          n56 = flat-sequence {
            tunnel: w53 -> [w62]
            tunnel: [w62] -> _
            frame #0 {
              # "Wait 5 seconds for\nthe ILX to stabilize"
              n57 = Wait (ms)(milliseconds to wait=u32 5000) -> ()  [unwired: 1 out]
            }
          }
        }
        frame Enabled {
        }
      }
      n58 = local write "Settings"("Settings") -> ()
    }
    frame #2 {
      # "Active X commands to the Newport 1918-C"
      # "Set the  channel of\nthe Newport 1918-C"
      # "Set the operational mode\nof the Newport 1918-C"
      # "Open commumication\nto the Newport 1918-C"
      n59 = constructor class="PowerMeterCommands"("logging"="logging", "deviceKey"="NewportIn") -> (reference out=w94:refnum<k24>, error out=w91:errorcluster, "deviceKey"=w86:string)  [unwired: 3 in, 2 out]
      "Newport Device Key" <- w86
      n60 = invoke class="PowerMeterCommands" method="GetPower"(reference=w94, error in=w91, "deviceKey"=w86) -> (reference out=w93:refnum<k24>, error out=w90:errorcluster)  [unwired: 1 in, 2 out]
      n61 = invoke class="PowerMeterCommands" method="SetChannel"(reference=w93, error in=w90, "deviceKey"=w86, "channel"="1") -> (reference out=w87:refnum<k24>, error out=w89:errorcluster)  [unwired: 1 in, 3 out]
      n62 = invoke class="PowerMeterCommands" method="CmdGetPower"(reference=w87, error in=w89, "deviceKey"=w86, "power"=sgl 0.0) -> (reference out=→"NewportRef":refnum<k24>)  [unwired: 1 in, 4 out]
    }
    frame #3 {
      # "Clean up multiply and divide by powers of 10 with comments\nBMM 6/19/14"
      # "Generating an array that is 'Number of Bins' long, filled wih the relevant altitude values for later plotting of Range \nCorrected Returns"
      # "Generating an array that is 'Number of Bins' long, filled wih the relevant altitude values for later plotting of returns"
      # "Generate arrays for the altitude and range corrected return altitude.  To be used later for plotting purposes."
      n63 = local read "Time Resolution Per Bin(ns)"() -> (w107:u32)
      n64 = local read "Time Resolution Per Bin(ns)"() -> (w97:u32)
      n65 = local read "Number of Bins"() -> (w110:u32)
      n66 = local read "Number of Bins"() -> (w100:u32)
      n67 = Divide(x=w107, y=1000000000.0) -> (x/y=w105:dbl)
      n68 = Divide(x=w97, y=1000000000.0) -> (x/y=w95:dbl)
      n69 = Multiply(x=w105, y=150000.0) -> (x*y=w108:dbl)
      n70 = Initialize Array(0.0, 0) -> (w113:dbl[])
      n71 = Multiply(x=w95, y=150000000.0) -> (x*y=w98:dbl)
      n72 = Initialize Array(0.0, 0) -> (w103:dbl[])
      n73 = for {
        N: w110 -> [_]
        shift-right: [w126] -> w111
        shift-left: w113 -> [w127]
        tunnel: w108 -> [w123]
        i -> [w125]
        n74 = Multiply(x=w123, y=w125) -> (x*y=w124:dbl)
        n75 = Add(x=w124, y=w123) -> (x+y=w122:dbl)
        n76 = Build Array (concatenate)(w127, w122) -> (w126:dbl[])
      }
      "Altitude Array (km)" <- w111
      n77 = for {
        N: w100 -> [_]
        shift-right: [w120] -> w101
        shift-left: w103 -> [w121]
        tunnel: w98 -> [w116]
        i -> [w119]
        n78 = Multiply(x=w116, y=w119) -> (x*y=w117:dbl)
        n79 = Add(x=w117, y=w116) -> (x+y=w115:dbl)
        n80 = Multiply(x=w115, y=w115) -> (x*y=w118:dbl)
        n81 = Build Array (concatenate)(w121, w118) -> (w120:dbl[])
      }
      "Range Corrected Altitude Array" <- w101
      n82 = local write "Altitude Array (km)"(w111) -> ()
      n83 = local write "Range Corrected Altitude Array"(w101) -> ()
    }
    frame #4 {
      # "Frame 4: Collect data from the scaler card and process and file it"
      n84 = while {
        tunnel: ["stop"] -> w128
        i -> [w129]
        stop <- "stop" stop-if-true
        # "While loop continues data collection cycle"
        n85 = case shown="True" "Collect Data?" {
          frame False {
            # "If 'Collect Data?' is false, wait a ms and check the 'Collect Data?' value again"
            n86 = Wait (ms)(milliseconds to wait=u32 1) -> ()  [unwired: 1 out]
          }
          frame True {
            # "Frame 3: Read the offline wavelength and lock if necessary (code not finished), read output power, read offline data, perform calculations and plot/save offline and NRB data, switch to online\nFrame 4: Calculate the absorption cross section (if wavelength, T, or P changed)\nFrame 5: Calculate Water Vapor Number density and plot"
            # "Frame 0: Create folders and file paths for logging the data, initialize averaging index\nFrame 1: Import current pressure and temperature data from COE weather station\nFrame 2: Read the online wavelength and lock if necessary, read online data and output power\n, plot and save online data, switch to offline DBR"
            # "If 'Collect Data?' is true, collect, process, and log data"
            n87 = stacked-sequence {
              frame #0 {
                # "Looking to see if the current Yr/Mo/Dy/Hr folder exists\nin the data disk folder (E:\\Micropulse_DIAL_data), if not,\ncreate one for the data"
                n88 = local read "FileHour"() -> (w142:i32)
                n89 = Get Date/Time In Seconds() -> (seconds since 1Jan1904=w134:timestamp)
                n90 = Seconds To Date/Time(time stamp (now)=w134) -> (date time rec=w144:T12)  [unwired: 1 in]
                n91 = Unbundle By Name(w144) -> ("hour"=w133:i32)
                n92 = case shown="True" "Reset Average" {
                  frame False {
                    n93 = local write "Index"(0 ("Index")) -> ()
                  }
                  frame True {
                    n94 = local read "Index"() -> (w232:i32)
                    n95 = Add(x=w232, y=1) -> (x+y=w231:i32)
                    n96 = local write "Index"(w231) -> ()
                  }
                }
                n97 = Equal?(x=w142, y=w133) -> (x = y?=w143:bool)
                n98 = Format Date/Time String(time format string (%c)="%y%m%d", seconds (now)=w134) -> (date/time string=w138:string)  [unwired: 1 in]
                n99 = Concatenate Strings("Data File DIR (in)", w138, "FF" ("string")) -> (w140:string)
                n100 = Concatenate Strings("Data File DIR (in)", w138, "NF" ("string")) -> (w135:string)
                n101 = case shown="False" w143 {
                  tunnel: w140 -> [w202 _]
                  tunnel: w135 -> [w201 _]
                  tunnel: w134 -> [w188 _]
                  tunnel: w133 -> [w164 _]
                  frame False {
                    # "Are data files open?"
                    # "Within the \"E:\\Micropulse_DIAL_data...\n'Current month/day/year' \ncheck if the current hour folder exists,\nif not, create one"
                    n102 = local write "FileHour"(w164) -> ()
                    n103 = flat-sequence {
                      tunnel: [w222] -> w189
                      tunnel: w202 -> [w221]
                      tunnel: w201 -> [w222]
                      tunnel: [w221] -> w190
                      frame #0 {
                        # "Does \"E:\\Micropulse_DIAL_data...\n'Current month/day/year' exist?\nIf not, create a new folder with that name"
                        n104 = String To Path(string=w221) -> (path=w226:path)
                        n105 = String To Path(string=w222) -> (path=w224:path)
                        n106 = call <vilib>:"Check if File or Folder Exists.vi"("path"=w226) -> ("file or folder exists?"=w225:bool)  [unwired: 8 in, 2 out]
                        n107 = call <vilib>:"Check if File or Folder Exists.vi"("path"=w224) -> ("file or folder exists?"=w223:bool)  [unwired: 8 in, 2 out]
                        n108 = case shown="False" w225 {
                          tunnel: w226 -> [w228 _]
                          frame False {
                            # "create new folder"
                            n109 = Create Folder(path (use dialog)=w228) -> ()  [unwired: 2 in, 3 out]
                          }
                          frame True {
                            # "Folder exists\ndo nothing"
                          }
                        }
                        n110 = case shown="False" w223 {
                          tunnel: w224 -> [w227 _]
                          frame False {
                            # "create new folder"
                            n111 = Create Folder(path (use dialog)=w227) -> ()  [unwired: 2 in, 3 out]
                          }
                          frame True {
                            # "Folder exists\ndo nothing"
                          }
                        }
                      }
                    }
                    n112 = Concatenate Strings(w190, "\\" ("string")) -> (w197:string)
                    n113 = Concatenate Strings(w189, "\\" ("string")) -> (w192:string)
                    n114 = Format Date/Time String(time format string (%c)="%H", seconds (now)=w188) -> (date/time string=w200:string)  [unwired: 1 in]
                    n115 = Format Date/Time String(time format string (%c)="%H", seconds (now)=w188) -> (date/time string=w195:string)  [unwired: 1 in]
                    n116 = Concatenate Strings(w197, w200) -> (w160:string)
                    "File Path_Far Field (out)" <- w160
                    n117 = Concatenate Strings(w192, w195) -> (w161:string)
                    "File Path_Near Field (out)" <- w161
                    n118 = String To Path(string=w160) -> (path=w198:path)
                    n119 = String To Path(string=w161) -> (path=w193:path)
                    n120 = call <vilib>:"Check if File or Folder Exists.vi"("path"=w198) -> ("file or folder exists?"=w187:bool, "dup path"=w185:path)  [unwired: 8 in, 1 out]
                    n121 = call <vilib>:"Check if File or Folder Exists.vi"("path"=w193) -> ("file or folder exists?"=w186:bool, "dup path"=w184:path)  [unwired: 8 in, 1 out]
                    n122 = case shown="False" w187 {
                      tunnel: w185 -> [w219 _]
                      tunnel: w160 -> [w218 w220]
                      tunnel: [w218 w220] -> w158
                      frame False {
                        # "new folder"
                        n123 = Create Folder(path (use dialog)=w219) -> ()  [unwired: 2 in, 3 out]
                      }
                      frame True {
                        # "Folder exists\ndo nothing"
                      }
                    }
                    n124 = case shown="False" w186 {
                      tunnel: w184 -> [w216 _]
                      tunnel: w161 -> [w215 w217]
                      tunnel: [w215 w217] -> w159
                      frame False {
                        # "new folder"
                        n125 = Create Folder(path (use dialog)=w216) -> ()  [unwired: 2 in, 3 out]
                      }
                      frame True {
                        # "Folder exists\ndo nothing"
                      }
                    }
                    n126 = Concatenate Strings(w159, "\\Online_Raw_Data.dat" ("string")) -> (w178:string)
                    n127 = Concatenate Strings(w159, "\\Offline_Raw_Data.dat" ("string")) -> (w177:string)
                    n128 = Concatenate Strings(w158, "\\Online_Raw_Data.dat" ("string")) -> (w183:string)
                    n129 = Concatenate Strings(w158, "\\Offline_Raw_Data.dat" ("string")) -> (w182:string)
                    n130 = local read "DataOpen"() -> (w175:bool)
                    n131 = String To Path(string=w183) -> (path=w174:path)
                    n132 = String To Path(string=w182) -> (path=w173:path)
                    n133 = String To Path(string=w178) -> (path=w172:path)
                    n134 = String To Path(string=w177) -> (path=w171:path)
                    n135 = case shown="True" w175 {
                      tunnel: w174 -> [w206 w210]
                      tunnel: [w206 w210] -> w168
                      tunnel: w173 -> [w205 w209]
                      tunnel: [w205 w209] -> w167
                      tunnel: w172 -> [w204 w208]
                      tunnel: [w204 w208] -> w166
                      tunnel: [w203 w207] -> w165
                      tunnel: w171 -> [w203 w207]
                      frame False {
                        # "No files open\ndo nothing"
                      }
                      frame True {
                        # "Close open files"
                        n136 = local read "NF_Off_Ref"() -> (w212:refnum<file>)
                        n137 = local read "NF_On_Ref"() -> (w211:refnum<file>)
                        n138 = local read "FF_Off_Ref"() -> (w214:refnum<file>)
                        n139 = local read "FF_On_Ref"() -> (w213:refnum<file>)
                        n140 = Close File(refnum=w213) -> ()  [unwired: 1 in, 2 out]
                        n141 = Close File(refnum=w214) -> ()  [unwired: 1 in, 2 out]
                        n142 = Close File(refnum=w211) -> ()  [unwired: 1 in, 2 out]
                        n143 = Close File(refnum=w212) -> ()  [unwired: 1 in, 2 out]
                      }
                    }
                    n144 = Open/Create/Replace File(file path (use dialog)=w168, operation (0:open)=T10."open or create") -> (refnum out=w154:refnum<file>)  [unwired: 4 in, 2 out]
                    n145 = Open/Create/Replace File(file path (use dialog)=w167, operation (0:open)=T10."open or create") -> (refnum out=w155:refnum<file>)  [unwired: 4 in, 2 out]
                    n146 = Open/Create/Replace File(file path (use dialog)=w166, operation (0:open)=T10."open or create") -> (refnum out=w156:refnum<file>)  [unwired: 4 in, 2 out]
                    n147 = Open/Create/Replace File(file path (use dialog)=w165, operation (0:open)=T10."open or create") -> (refnum out=w157:refnum<file>)  [unwired: 4 in, 2 out]
                    n148 = Get File Size(file=w154) -> (refnum out=→"FF_On_Ref":refnum<file>, size (in bytes)=→"FF_On_Ptr":i64)  [unwired: 1 in, 1 out]
                    n149 = Get File Size(file=w155) -> (refnum out=→"FF_Off_Ref":refnum<file>, size (in bytes)=→"FF_Off_Ptr":i64)  [unwired: 1 in, 1 out]
                    n150 = Get File Size(file=w156) -> (refnum out=→"NF_On_Ref":refnum<file>, size (in bytes)=→"NF_On_Ptr":i64)  [unwired: 1 in, 1 out]
                    n151 = Get File Size(file=w157) -> (refnum out=→"NF_Off_Ref":refnum<file>, size (in bytes)=→"NF_Off_Ptr":i64)  [unwired: 1 in, 1 out]
                  }
                  frame True {
                    # "Don't need to do anything!"
                  }
                }
              }
              frame #1 {
                # "Writing and plotting retrieved\nweather parameters"
                # "Matlab script goes online and retrieves most recent press, temp, and relative humidity data \nfrom the weather station on the roof of Cobleigh"
                # "Importing the current weather conditions from the COE weather station"
                n152 = disable-structure shown="Disabled" {
                  frame Disabled {
                    n153 = script code="%try\n%s=urlread('http://www.coe.montana.edu/ee/weather/mostCurrentCSV.php');\n%amin=textscan(s,'%s %s %s %s %s %s %s %s %s %s %s %s %s');\n%data=amin{1}{2};\n%[test remain]=strtok(data,',');\n%remain=str2num(remain);\n%press=remain(3)./1000;\n%temp=remain(5);\n%RH=remain(7);\n%catch\npress=.850;\ntemp=20;\nRH=40;\n%end"() -> ()  [unwired: 1 in, 4 out]
                  }
                  frame Enabled {
                  }
                }
                "Temperature (C)" <- "Temperature (C)"
                "Pressure (mb)" <- "Pressure (mbar or hPa)"
                "Relative Humdity (%)" <- 40.0 ("Real")
              }
              frame #2 {
                # "Frame 3: Read, process, and plot online data\nFrame 4: Switch to the offline DBR seed\nFrame 5: Write the data to the folders from Frame 0 of outter sequence"
                # "Frame 0: Read the online wavelength and adjust to locking tolerance if out of range\nFrame 1: Read the output power from the Newport meter, calculate and plot the output pulse energy\nFrame 2: Wait 'Scalar Wait Time' for buffer to clear other wavelength data"
                # "Online"
                n154 = stacked-sequence {
                  frame #0 {
                    # "Read the online wavelength and continue adjusting the online DBR if outside the wavelength tolerance\nuntil it is within tolerance"
                    n155 = while {
                      i -> [w239]
                      stop <- w237 stop-if-true
                      # "Frame 2: Decrement DBR current if above tolerance\nFrame 3: Increment DBR current if below tolerance"
                      # "Frame 0: Read the current wavelength from the wavemeter\nFrame 1: Calculate the difference between desired and actual wavelength"
                      # "Continue reading and adjusting online DBR current until within locking tolerance"
                      n156 = stacked-sequence {
                        tunnel: w239 -> [w241 _ _ _ _]
                        tunnel: [_ _ w248 _ _] -> w238
                        frame #0 {
                          n157 = Equal To 0?(x=w241) -> (x = 0?=w240:bool)
                          n158 = case shown="True" w240 {
                            frame False {
                            }
                            frame True {
                              # "SWITCH to ABSORBING"
                              n159 = Build Array(FALSE ("Boolean")) -> (w242:bool[])
                              n160 = call-poly <vilib>:"DAQmx Write.vi"("task/channels in"=refnum<k21> "BristolWM", "data"=w242) -> ()  [unwired: 11 in, 3 out]
                            }
                          }
                        }
                        frame #1 {
                          # "Read Bristol WM"
                          n161 = local read "Bristol Out"() -> (w245:i32)
                          n162 = dll-call lib="C:/H2O_DIAL/LabVIEW-2012/Bristol WM V2_31b/CLDevIface.dll" fn="CLGetLambdaReading"("devHandle"=w245) -> ("return type"=→"Lambda On Read (nm)":dbl)  [unwired: 4 in, 2 out]
                        }
                        frame #2 {
                          # "If WL difference is within tolerance, stop looping, and illuminate 'Wavelength Lock Online' indicator"
                          # "Calculating the difference between the actual and desired online wavelength"
                          n163 = local read "Lambda On Read (nm)"() -> (w255:dbl)
                          n164 = local read "AB_DIF"() -> (w252:dbl)
                          n165 = Subtract(x=w255, y="Lambda On Set (nm)") -> (x-y=w247:dbl)
                          "WL Difference" <- w247
                          n166 = Multiply(x=-1.0, y=w252) -> (x*y=w253:dbl)
                          n167 = Greater?(x=w247, y=w253) -> (0:w249:bool)
                          n168 = Less?(x=w247, y=w252) -> (x < y?=w250:bool)
                          n169 = And(x=w249, y=w250) -> (x .and. y?=w248:bool)
                          "Wavelength Lock Online" <- w248
                        }
                        frame #3 {
                          # "If the wavelength difference is greater that 0.0002 nm, decrement the \nDBR current by 0.01 mA"
                          n170 = local read "WL Difference"() -> (w258:dbl)
                          n171 = Greater Or Equal?(x=w258, y="AB_DIF") -> (x >= y?=w256:bool)
                          n172 = case shown="True" w256 {
                            frame False {
                              # "Wavelength difference is not greater than 0.0002 nm, do nothing"
                            }
                            frame True {
                              # "Generating a command string\nto decrement the current"
                              # "WL difference is greater than 0.0002 nm,\ndecrement the DBR current by 0.01 mA"
                              n173 = local read "Settings"() -> (w263:T7)
                              n174 = Unbundle By Name(w263) -> ("OnLineLD"=w265:dbl)
                              n175 = Subtract(x=w265, y=3e-06) -> (x-y=w266:dbl)
                              n176 = Bundle By Name(cluster=w263, "OnLineLD"=w266, "Module"=T11."On Line LD") -> (w261:T7)
                              n177 = call "TL_Driver.vi"("Device In"=refnum<visa-resource-name> "ThorLabs", "Commands"=T8."SET", "Settings"=w261) -> ("Readings"=w259:T6)  [unwired: 9 in, 3 out]
                              n178 = local write "Settings"(w261) -> ()
                              n179 = local write "Readings"(w259) -> ()
                            }
                          }
                        }
                        frame #4 {
                          # "If the wavelength difference is less that 0.0002 nm, increment the \nDBR current by 0.01 mA"
                          n180 = local read "WL Difference"() -> (w272:dbl)
                          n181 = local read "AB_DIF"() -> (w270:dbl)
                          n182 = Multiply(x=-1.0, y=w270) -> (x*y=w268:dbl)
                          n183 = Less Or Equal?(x=w272, y=w268) -> (x <= y?=w271:bool)
                          n184 = case shown="True" w271 {
                            frame False {
                              # "WL difference is no <= to -0.0002 nm, do nothing"
                            }
                            frame True {
                              # "WL difference is < -0.0002,\nincrement the DBR current by 0.01 mA"
                              # "Generating a command string\nto decrement the current"
                              n185 = local read "Settings"() -> (w277:T7)
                              n186 = Unbundle By Name(w277) -> ("OnLineLD"=w279:dbl)
                              n187 = Add(x=w279, y=3e-06) -> (x+y=w280:dbl)
                              n188 = Bundle By Name(cluster=w277, "OnLineLD"=w280, "Module"=T11."On Line LD") -> (w274:T7)
                              n189 = call "TL_Driver.vi"("Device In"=refnum<visa-resource-name> "ThorLabs", "Commands"=T8."SET", "Settings"=w274) -> ("Readings"=w273:T6)  [unwired: 9 in, 3 out]
                              n190 = local write "Settings"(w274) -> ()
                              n191 = local write "Readings"(w273) -> ()
                            }
                          }
                        }
                      }
                      n192 = Or(x=w238, y="Cancel online") -> (x .or. y?=w237:bool)
                    }
                  }
                  frame #1 {
                    # "Converting to pulse energy, assumes 5 percent pickoff"
                    # "Reading the Newport Power meter"
                    # "Reading the output power of the laser transmitter from the Newport power meter, once read, convert to corresponding pulse energy and plot"
                    n193 = local read "Newport Device Key"() -> (w286:string)
                    n194 = local read "NewportRef"() -> (w282:refnum<k24>)
                    n195 = Number To Decimal String(number="SampleSize") -> (decimal integer string=w284:string)  [unwired: 1 in]
                    n196 = disable-structure shown="Disabled" {
                      frame Disabled {
                        # "Plotting the online and offling pulse energies"
                        n197 = local read "Online Pulse Energy"() -> (w297:dbl)
                        n198 = local read "Offline Pulse Energy"() -> (w296:dbl)
                        n199 = Bundle("Online Pulse Energy"=w297, "Offline Pulse Energy"=w296) -> (→"Pulse Energy (Micro Joule)":T13)  [unwired: 1 in]
                      }
                      frame Enabled {
                      }
                    }
                    n200 = invoke class="PowerMeterCommands" method="PerformDAQ"(reference=w282, "deviceKey"=w286, "interval"="1", "sampleSize"=w284) -> ("PerformDAQ"=w287:dbl[])  [unwired: 2 in, 5 out]
                    n201 = call-poly <vilib>:"Mean.vi"("X"=w287) -> ("mean"=w285:dbl)  [unwired: 1 out]
                    n202 = Multiply(x=w285, y=1000.0) -> (x*y=w293:dbl)
                    n203 = Divide(x=w293, y=0.05) -> (x/y=w291:dbl)
                    n204 = Divide(x=w291, y="PRF (kHz)") -> (x/y=→"Online Pulse Energy":dbl)
                  }
                  frame #2 {
                    # "Waiting 'Scalar Wait Time'"
                    # "Wait 'Scalar Wait Time' for the next available batch of scalar card data"
                    n205 = Wait (ms)(milliseconds to wait="Scalar Wait Time") -> ()  [unwired: 1 out]
                  }
                  frame #3 {
                    # "convert time per range bin to meters\nand calculate smoothed bins using\nsmoothing range"
                    # "Plotting online cross section and smoothed online data"
                    # "Calculate the bin by bin mean of the data"
                    # "Collect 'Integration Period (Seconds)' number\nof scalar data"
                    # "Reading, processing, and plotting the online data"
                    n206 = local read "Data Reads (number of loops)"() -> (w324:i32)
                    n207 = for {
                      N: w324 -> [_]
                      tunnel: [w345] -> w336 mode=indexing
                      tunnel: [w344] -> w316 mode=indexing
                      # "Scalar Data is retrieved from Global \nVariable that scaler.vi is writing to,"
                      n208 = global read "Scalar_Data.vi" "Scalar Data"() -> (w345:u16[])
                      n209 = global read "Scalar_Data.vi" "Scalar Data  3"() -> (w344:u16[])
                    }
                    n210 = Transpose 2D Array(2D array=w336) -> (transposed array=w340:u16[][])
                    n211 = Transpose 2D Array(2D array=w316) -> (transposed array=w322:u16[][])
                    n212 = for {
                      tunnel: w340 -> [w347] mode=indexing
                      tunnel: [w346] -> w341 mode=indexing
                      n213 = call-poly <vilib>:"Mean.vi"("X"=w347) -> ("mean"=w346:dbl)  [unwired: 1 out]
                    }
                    n214 = for {
                      tunnel: w322 -> [w343] mode=indexing
                      tunnel: [w342] -> w323 mode=indexing
                      n215 = call-poly <vilib>:"Mean.vi"("X"=w343) -> ("mean"=w342:dbl)  [unwired: 1 out]
                    }
                    n216 = local read "bins"() -> (w315:u32)
                    n217 = Array Subset(array=w341, index=1 ("dimension size"), length=w315) -> (w328:dbl[])
                    n218 = Array Subset(array=w323, index=1 ("dimension size"), length=w315) -> (w320:dbl[])
                    n219 = local read "background length"() -> (w305:i32)
                    n220 = local read "background start"() -> (w306:u32)
                    n221 = Array Size(array=w328) -> (size(s)=w325:i32)
                    n222 = Array Size(array=w320) -> (size(s)=w317:i32)
                    n223 = Initialize Array(1.0 ("element"), w325) -> (w327:dbl[])
                    n224 = Initialize Array(1.0 ("element"), w317) -> (w319:dbl[])
                    n225 = Multiply(x=w328, y=w327) -> (x*y=w329:dbl[])
                    "On-Line Bin Readings" <- w329
                    n226 = Multiply(x=w320, y=w319) -> (x*y=w309:dbl[])
                    "On-Line Bin Readings 2" <- w309
                    n227 = local read "Total DIAL Integration Time (Minutes)"() -> (w332:i32)
                    n228 = local read "Time Resolution Per Bin(ns)"() -> (w301:u32)
                    n229 = Array Subset(array=w329, index=w306, length=w305) -> (w338:dbl[])
                    n230 = Array Subset(array=w309, index=w306, length=w305) -> (w311:dbl[])
                    n231 = call-poly <vilib>:"Mean.vi"("X"=w338) -> ("mean"=w337:dbl)  [unwired: 1 out]
                    n232 = call-poly <vilib>:"Mean.vi"("X"=w311) -> ("mean"=w312:dbl)  [unwired: 1 out]
                    n233 = Divide(x=w332, y=w324) -> (x/y=w330:dbl)
                    n234 = local read "Index"() -> (w310:i32)
                    n235 = Subtract(x=w329, y=w337) -> (x-y=w334:dbl[])
                    n236 = Subtract(x=w309, y=w312) -> (x-y=w313:dbl[])
                    n237 = To Double Precision Float(number=w301) -> (double precision float=w302:dbl)
                    n238 = Multiply(x=w330, y=60.0) -> (x*y=w307:dbl)
                    n239 = Multiply(x=w302, y=0.15) -> (x*y=w304:dbl)
                    n240 = call "Ring Buffer Online Far.vi"("Index"=w310, "Profiles to Average"=w307, "Input Array"=w334) -> ("AvgArray"=w333:dbl[])  [unwired: 7 in, 1 out]
                    n241 = call "Ring Buffer Online Near.vi"("Index"=w310, "Profiles to Average"=w307, "Input Array"=w313) -> ("AvgArray"=w314:dbl[])  [unwired: 7 in, 1 out]
                    n242 = Divide(x="Smoothing Range", y=w304) -> (x/y=w299:dbl)
                    "Smoothed Bins" <- w299
                    n243 = call "Smooth Arrray.vi"("smooth size"=w299, "Raw Array"=w333) -> ("Smoothed Array"=→"On-Line  Smoothed":dbl[])  [unwired: 9 in]
                    n244 = call "Smooth Arrray.vi"("smooth size"=w299, "Raw Array"=w314) -> ("Smoothed Array"=→"On-Line Smoothed 2":dbl[])  [unwired: 9 in]
                    n245 = disable-structure shown="Disabled" {
                      frame Disabled {
                        n246 = script code="format long;\ncounts=sum(Online);\nif counts >=0.5e6\ntime=time;\nelse\ntime=time\nend"() -> ()  [unwired: 3 in, 2 out]
                      }
                      frame Enabled {
                      }
                    }
                  }
                  frame #4 {
                    # "Toggling the Agiltron switch to the offline DBR seed laser"
                    n247 = disable-structure shown="Disabled" {
                      frame Disabled {
                        n248 = flat-sequence {
                          frame #0 {
                            # "Second one"
                            # "Command the switch to switch to position 2\ncorresponding to the offline DBR"
                            # "Hex string command \ncorrespond to offline"
                            n249 = VISA Write(VISA resource name="Switch Comm Port", write buffer="\u0001\u0012\u0000\u0001") -> ()  [unwired: 1 in, 3 out]
                          }
                        }
                      }
                      frame Enabled {
                      }
                    }
                  }
                  frame #5 {
                    # "Save the recently collected online data if 'Save Data?' is true"
                    n250 = case shown="True" "Save Data?" {
                      frame False {
                        # "'Save Data?' is false, do nothing"
                      }
                      frame True {
                        # "'Save Data?' is true, save onfline data to the Data Disk"
                        # "Write only one copy of data at this time"
                        # "Retrieve Julian Date"
                        n251 = local read "Readings"() -> (w358:T6)
                        n252 = local read "Time Resolution Per Bin(ns)"() -> (w356:u32)
                        n253 = local read "Number of Accumulates"() -> (w354:u32)
                        n254 = local read "Number of Bins"() -> (w355:u32)
                        n255 = local write "DataOpen"(TRUE ("DataOpen")) -> ()
                        n256 = local read "Lambda On Read (nm)"() -> (w380:dbl)
                        n257 = local read "On-Line Bin Readings 2"() -> (w378:dbl[])
                        n258 = local read "On-Line Bin Readings"() -> (w382:dbl[])
                        n259 = local read "Online Pulse Energy"() -> (w379:dbl)
                        n260 = Unbundle By Name(w358) -> ("OnLineLD"=w357:dbl)
                        n261 = To Double Precision Float(number=w356) -> (double precision float=w353:dbl)
                        n262 = To Double Precision Float(number=w355) -> (double precision float=w352:dbl)
                        n263 = To Double Precision Float(number=w354) -> (double precision float=w351:dbl)
                        n264 = call "Julian_Date_2.vi"() -> ("Julian Date"=w381:dbl)  [unwired: 11 in]
                        n265 = Build Array (concatenate)(w381, w380, w357, w379, w353, w352, w351, w382) -> (w373:dbl[])
                        n266 = Build Array (concatenate)(w381, w380, w357, w379, w353, w352, w351, w378) -> (w363:dbl[])
                        n267 = local read "NF_On_Ref"() -> (w361:refnum<file>)
                        n268 = local read "FF_On_Ref"() -> (w377:refnum<file>)
                        n269 = local read "NF_On_Ptr"() -> (w362:i64)
                        n270 = local read "FF_On_Ptr"() -> (w376:i64)
                        n271 = Set File Position(offset (in bytes) (0)=w376, refnum=w377) -> (refnum out=w374:refnum<file>, error out=w371:errorcluster)  [unwired: 2 in]
                        n272 = Set File Position(offset (in bytes) (0)=w362, refnum=w361) -> (refnum out=w367:refnum<file>, error out=w365:errorcluster)  [unwired: 2 in]
                        n273 = Write to Binary File(file (use dialog)=w367, data=w363, error in=w365, 5:FALSE ("prepend array or string size? (T)")) -> (refnum out=w366:refnum<file>, error out=w364:errorcluster)  [unwired: 2 in, 1 out]
                        n274 = Write to Binary File(file (use dialog)=w374, data=w373, error in=w371, 5:FALSE ("prepend array or string size? (T)")) -> (refnum out=w372:refnum<file>, error out=w370:errorcluster)  [unwired: 2 in, 1 out]
                        n275 = Get File Position(4:w364, 7:w366) -> (2:w360:i64)  [unwired: 2 out]
                        n276 = Get File Position(4:w370, 7:w372) -> (2:w369:i64)  [unwired: 2 out]
                        n277 = local write "NF_On_Ptr"(w360) -> ()
                        n278 = local write "FF_On_Ptr"(w369) -> ()
                      }
                    }
                  }
                }
              }
              frame #3 {
                # "Frame 3: Read offline data, calculate aerosol data, and plot offline and normalized relative backscatter\nFrame 4: Swich to online DBR\nFrame 5: Save the offline data and related information"
                # "Frame 0: Read the offline wavelength and lock if necessary, though code is not finished to do so\nFrame 1: Read the output power from the Newport power meter\nFrame 2: Wait 'Scalar Wait Time' for buffers to clear of online contiminated data"
                # "offline"
                n279 = stacked-sequence {
                  frame #0 {
                    # "Every 60 data collection cycles, read the offline DBR wavelength, and if outside of wavelength tolerance, adjust DBR current until within tolerance"
                    n280 = local read "L_Count"() -> (w384:i32)
                    n281 = Quotient & Remainder(x=w384, y=60.0) -> (x-y*floor(x/y)=w385:dbl)  [unwired: 1 out]
                    n282 = Equal To 0?(x=w385) -> (x = 0?=w383:bool)
                    n283 = case shown="True" w383 {
                      frame False {
                      }
                      frame True {
                        n284 = while {
                          i -> [w390]
                          stop <- w388 stop-if-true
                          # "Frame 5 Increment ofline DBR current if below tolerance\nFrame 6: update ILX settings to front pannel"
                          # "Frame 3: Calculating the wavelength difference\nFrame 4:Decrement offline DBR current if above tolerance"
                          # "Frame 0: Read the offline laser wavelength (settle if t=0)"
                          n285 = stacked-sequence {
                            tunnel: w390 -> [w392 _ _ _ _]
                            tunnel: [_ _ w402 _ _] -> w389
                            frame #0 {
                              n286 = Equal To 0?(x=w392) -> (x = 0?=w391:bool)
                              n287 = case shown="True" w391 {
                                frame False {
                                }
                                frame True {
                                # "SWITCH to NON-ABSORBING and wait to settle"
                                n288 = Build Array(TRUE ("Boolean")) -> (w397:bool[])
                                n289 = call-poly <vilib>:"DAQmx Write.vi"("task/channels in"=refnum<k21> "BristolWM", "data"=w397) -> ()  [unwired: 11 in, 3 out]
                                n290 = call "TL_Driver.vi"("Device In"=refnum<visa-resource-name> "ThorLabs", "Commands"=T8."Read_Status") -> ("Readings"=w395:T6)  [unwired: 10 in, 3 out]
                                n291 = local write "Readings"(w395) -> ()
                                n292 = Wait (ms)(milliseconds to wait=u32 3200) -> ()  [unwired: 1 out]
                                }
                              }
                            }
                            frame #1 {
                              # "Read Bristol WM"
                              n293 = local read "Bristol Out"() -> (w400:i32)
                              n294 = dll-call lib="C:/H2O_DIAL/LabVIEW-2012/Bristol WM V2_31b/CLDevIface.dll" fn="CLGetLambdaReading"("devHandle"=w400) -> ("return type"=→"Lambda Off Read (nm)":dbl)  [unwired: 4 in, 2 out]
                            }
                            frame #2 {
                              # "Once locked, stop looping and illuminate 'Wavelength Lock Offline'"
                              # "While loop continues locking process until the wavelength is within tolerance"
                              # "Calculating the difference between the actual and desired \noffline wavelength"
                              n295 = local read "Lambda Off Read (nm)"() -> (w410:dbl)
                              n296 = Subtract(x=w410, y="Lambda Off Set (nm)") -> (x-y=w403:dbl)
                              "WL Difference off" <- w403
                              n297 = local read "NONAB_DIF"() -> (w407:dbl)
                              n298 = Multiply(x=-1.0, y=w407) -> (x*y=w408:dbl)
                              n299 = Greater?(x=w403, y=w408) -> (0:w404:bool)
                              n300 = Less?(x=w403, y=w407) -> (x < y?=w405:bool)
                              n301 = And(x=w404, y=w405) -> (x .and. y?=w402:bool)
                              "Wavelength Lock Offline" <- w402
                              n302 = case shown="True" w402 {
                                frame False {
                                }
                                frame True {
                                # "SWITCH back to ABSORBING and wait to settle"
                                n303 = Build Array(FALSE ("Boolean")) -> (w412:bool[])
                                n304 = call-poly <vilib>:"DAQmx Write.vi"("task/channels in"=refnum<k21> "BristolWM", "data"=w412) -> ()  [unwired: 11 in, 3 out]
                                n305 = Wait (ms)(milliseconds to wait=u32 3000) -> ()  [unwired: 1 out]
                                }
                              }
                            }
                            frame #3 {
                              # "Would adjust the offline wavelength if code was finished"
                              n306 = local read "WL Difference off"() -> (w417:dbl)
                              n307 = Greater Or Equal?(x=w417, y="NONAB_DIF") -> (x >= y?=w415:bool)
                              n308 = case shown="True" w415 {
                                frame False {
                                # "WL difference is not out of range, do nothing"
                                }
                                frame True {
                                # "Generating a command string\nto decrement the current"
                                # "WL difference is greater than 0.0002 nm,\ndecrement the DBR current by 0.01 mA"
                                # "WL difference is out of range, this is where you would decrement\nthe laser current"
                                n309 = local read "Settings"() -> (w422:T7)
                                n310 = Unbundle By Name(w422) -> ("OffLineLD"=w423:dbl)
                                n311 = Subtract(x=w423, y=3e-06) -> (x-y=w424:dbl)
                                n312 = Bundle By Name(cluster=w422, "OffLineLD"=w424, "Module"=T11."Off Line LD") -> (w421:T7)
                                n313 = call "TL_Driver.vi"("Device In"=refnum<visa-resource-name> "ThorLabs", "Commands"=T8."SET", "Settings"=w421) -> ("Readings"=w418:T6)  [unwired: 9 in, 3 out]
                                n314 = local write "Settings"(w421) -> ()
                                n315 = local write "Readings"(w418) -> ()
                                }
                              }
                            }
                            frame #4 {
                              # "This is where you would increment the offline current if below tolerance"
                              n316 = local read "NONAB_DIF"() -> (w428:dbl)
                              n317 = local read "WL Difference off"() -> (w431:dbl)
                              n318 = Multiply(x=-1.0, y=w428) -> (x*y=w427:dbl)
                              n319 = Less Or Equal?(x=w431, y=w427) -> (x <= y?=w430:bool)
                              n320 = case shown="True" w430 {
                                frame False {
                                # "WL difference is not outisde tolerance, do nothing"
                                }
                                frame True {
                                # "Generating a command string\nto decrement the current"
                                # "WL difference is less than 0.0002 nm,\nincrement the DBR current by 0.01 mA"
                                # "Incrementing the current if below tolerance"
                                n321 = local read "Settings"() -> (w435:T7)
                                n322 = Unbundle By Name(w435) -> ("OffLineLD"=w437:dbl)
                                n323 = Add(x=w437, y=3e-06) -> (x+y=w438:dbl)
                                n324 = Bundle By Name(cluster=w435, "OffLineLD"=w438, "Module"=T11."Off Line LD") -> (w436:T7)
                                n325 = call "TL_Driver.vi"("Device In"=refnum<visa-resource-name> "ThorLabs", "Commands"=T8."SET", "Settings"=w436) -> ("Readings"=w432:T6)  [unwired: 9 in, 3 out]
                                n326 = local write "Settings"(w436) -> ()
                                n327 = local write "Readings"(w432) -> ()
                                }
                              }
                            }
                          }
                          n328 = Or(x=w389, y="Cancel Offline") -> (x .or. y?=w388:bool)
                        }
                      }
                    }
                  }
                  frame #1 {
                    # "Reading the power meter"
                    # "Updating the pulse energy plot"
                    # "Converting to pulse energy"
                    # "Reading the offline output power, converting to pulse energy,  and updating the Pulse energy plot"
                    n329 = local read "SampleSize"() -> (w444:i32)
                    n330 = local read "Newport Device Key"() -> (w445:string)
                    n331 = local read "Online Pulse Energy"() -> (w451:dbl)
                    n332 = local read "Offline Pulse Energy"() -> (w450:dbl)
                    n333 = local read "NewportRef"() -> (w442:refnum<k24>)
                    n334 = Number To Decimal String(number=w444) -> (decimal integer string=w446:string)  [unwired: 1 in]
                    n335 = invoke class="PowerMeterCommands" method="PerformDAQ"(reference=w442, "deviceKey"=w445, "interval"="1", "sampleSize"=w446) -> ("PerformDAQ"=w447:dbl[])  [unwired: 2 in, 5 out]
                    n336 = Bundle("Online Pulse Energy"=w451, "Offline Pulse Energy"=w450) -> (w449:T13)  [unwired: 1 in]
                    n337 = local write "Pulse Energy (Micro Joule)"(w449) -> ()
                    n338 = call-poly <vilib>:"Mean.vi"("X"=w447) -> ("mean"=w443:dbl)  [unwired: 1 out]
                    n339 = local read "PRF (kHz)"() -> (w441:dbl)
                    n340 = Multiply(x=w443, y=1000.0) -> (x*y=w455:dbl)
                    n341 = Divide(x=w455, y=0.05) -> (x/y=w453:dbl)
                    n342 = Divide(x=w453, y=w441) -> (x/y=→"Offline Pulse Energy":dbl)
                  }
                  frame #2 {
                    # "Wait 'Scalar Wait Time' for buffers to clear of online contiminated offline data"
                    n343 = disable-structure shown="Disabled" {
                      frame Disabled {
                        # "Wait 'Scalar Wait Time'"
                        n344 = local read "Scalar Wait Time"() -> (w457:u32)
                        n345 = Wait (ms)(milliseconds to wait=w457) -> ()  [unwired: 1 out]
                      }
                      frame Enabled {
                      }
                    }
                  }
                  frame #3 {
                    w489 = 1 ("dimension size")
                    w493 = 1
                    # "Plotting the normalized relative \nbackscatter"
                    # "Calculating the normalized relative backscatter"
                    # "Calculating/Plotting smoothed data,\ncross sections etc."
                    # "Pick off data with\nout header"
                    # "Calculate mean bin by bin mean"
                    # "Reading in 'Integration Period (Seconds)' of data"
                    # "Read the offline data from the scalar card, perform smoothing, calculate normalized relative backscatter, and plot"
                    # "File path in MATLAB script is of old dial is:\nF:\\Micropulse DIAL\\Micropulse DIAL Matlab\\\nFinal Overlap Function.mat')];"
                    # "Collects Data From Card,\nSends It To The Chart,\nAnd Saves A Copy As A\nFile If Option Selected On\nFront Panel"
                    n346 = for {
                      N: "Data Reads (number of loops)" -> [_]
                      tunnel: [w527] -> w524 mode=indexing
                      tunnel: [w526] -> w506 mode=indexing
                      # "Read in latest scalar card data from \n'Scalar Data' global variable that \nscaler.vi is writing to, then wait 1 sec\nfor next batch of data"
                      n347 = global read "Scalar_Data.vi" "Scalar Data  4"() -> (w526:u16[])
                      n348 = global read "Scalar_Data.vi" "Scalar Data  2"() -> (w527:u16[])
                    }
                    n349 = local read "Total DIAL Integration Time (Minutes)"() -> (w515:i32)
                    n350 = Divide(x=w515, y="Data Reads (number of loops)") -> (x/y=w513:dbl)
                    n351 = local read "Total Aerosol Integration Time (Minutes)"() -> (w517:dbl)
                    n352 = local read "background length"() -> (w461:i32)
                    n353 = Multiply(x=w513, y=60.0) -> (x*y=w499:dbl)
                    n354 = local read "background start"() -> (w462:u32)
                    n355 = Transpose 2D Array(2D array=w524) -> (transposed array=w523:u16[][])
                    n356 = Transpose 2D Array(2D array=w506) -> (transposed array=w505:u16[][])
                    n357 = Divide(x=w517, y="Data Reads (number of loops)") -> (x/y=w518:dbl)
                    n358 = for {
                      tunnel: w523 -> [w531] mode=indexing
                      tunnel: [w530] -> w525 mode=indexing
                      tunnel: w505 -> [w529] mode=indexing
                      tunnel: [w528] -> _ mode=indexing
                      tunnel: [w528] -> w502 mode=indexing
                      n359 = call-poly <vilib>:"Mean.vi"("X"=w531) -> ("mean"=w530:dbl)  [unwired: 1 out]
                      n360 = call-poly <vilib>:"Mean.vi"("X"=w529) -> ("mean"=w528:dbl)  [unwired: 1 out]
                    }
                    n361 = local read "bins"() -> (w490:u32)
                    n362 = Multiply(x=w518, y=60.0) -> (x*y=w480:dbl)
                    n363 = Array Subset(array=w502, index=w489, length=w490) -> (w503:dbl[])
                    "Off-Line Bin Readings 2" <- w503
                    n364 = Array Subset(array=w525, index=w489, length=w490) -> (w501:dbl[])
                    "Off-Line  Bin Readings" <- w501
                    n365 = Array Subset(array=w503, index=w462, length=w461) -> (w504:dbl[])
                    n366 = Array Subset(array=w501, index=w462, length=w461) -> (w522:dbl[])
                    n367 = local read "Smoothed Bins"() -> (w458:dbl)
                    n368 = call-poly <vilib>:"Mean.vi"("X"=w504) -> ("mean"=w468:dbl)  [unwired: 1 out]
                    n369 = call-poly <vilib>:"Mean.vi"("X"=w522) -> ("mean"=w469:dbl)  [unwired: 1 out]
                    n370 = local read "Index"() -> (w479:i32)
                    n371 = Subtract(x=w503, y=w468) -> (x-y=w481:dbl[])
                    n372 = Subtract(x=w501, y=w469) -> (x-y=w497:dbl[])
                    n373 = call "Ring Buffer Offline Far.vi"("Index"=w479, "Profiles to Average"=w499, "Input Array"=w497) -> ("AvgArray"=w520:dbl[], "RingBufferOut"=→"RingBuffer offline far":dbl[][])  [unwired: 7 in]
                    n374 = call "Ring Buffer Aerosol Far.vi"("Index"=w479, "Profiles to Average"=w480, "Input Array"=w497) -> ("AvgArray"=w516:dbl[], "RingBufferOut"=→"RingBuffer aerosol far":dbl[][])  [unwired: 7 in]
                    n375 = call "Ring Buffer Offline Near.vi"("Index"=w479, "Profiles to Average"=w499, "Input Array"=w481) -> ("AvgArray"=w500:dbl[], "RingBufferOut"=→"RingBuffer offline near":dbl[][])  [unwired: 7 in]
                    n376 = call "Ring Buffer Aerosol Near.vi"("Index"=w479, "Profiles to Average"=w480, "Input Array"=w481) -> ("AvgArray"=w477:dbl[], "RingBufferOut"=→"RingBuffer aerosol near":dbl[][])  [unwired: 7 in]
                    n377 = Reshape Array(w497, w489, w490) -> (→"raw counts":dbl[][])
                    n378 = Reshape Array(w481, w489, w490) -> (→"raw counts near":dbl[][])
                    n379 = call "Smooth Arrray.vi"("smooth size"=w458, "Raw Array"=w520) -> ("Smoothed Array"=→"Off-Line Smoothed":dbl[])  [unwired: 9 in]
                    n380 = call "Smooth Arrray.vi"("smooth size"=w458, "Raw Array"=w516) -> ("Smoothed Array"=w488:dbl[])  [unwired: 9 in]
                    "Aerosol Smoothed" <- w488
                    n381 = call "Smooth Arrray.vi"("smooth size"=w458, "Raw Array"=w500) -> ("Smoothed Array"=→"Off-Line Smoothed 2":dbl[])  [unwired: 9 in]
                    n382 = call "Smooth Arrray.vi"("smooth size"=w458, "Raw Array"=w477) -> ("Smoothed Array"=w460:dbl[])  [unwired: 9 in]
                    "Aerosol Smoothed 2" <- w460
                    n383 = local read "Number of Accumulates"() -> (w464:u32)
                    n384 = local read "Temperature (C)"() -> (w512:dbl)
                    n385 = local read "Pressure (mb)"() -> (w511:dbl)
                    n386 = script code="%accum_num=10000;     % scaler card setting number of accumulations\nt_bin = 500e-9                 % scaler card setting time per bin\n%t_d = 37.3e-9;                % APD dead time from spec sheet\n\n% conversion from accumulated counts to count rate  (c/s)\nc_convert = 1./t_bin./accum_num;\nCR_far = p_raw_far.*c_convert;\nCR_near = p_raw_near.*c_convert;\nCR_total_far = (p_raw_far+b_far).*c_convert;\nCR_total_near = (p_raw_near+b_near).*c_convert;\nb_CR_far =b_far.*c_convert;\nb_CR_near =b_near.*c_convert;\n\n% create a range array\nsize_p =  size(p_raw_far,2);\nr = (75:75:size_p*75)./1e3; \n    \n%APD correction factor\n D_far = 1./(1-(t_d*CR_total_far));\n D_near = 1./(1-(t_d*CR_total_near));\n\n %Calculating normalize relative backscatter profile\n nrb_far = CR_far.*D_far.*r.^2./E.*1e-6;\n nrb_near = CR_near.*D_near.*r.^2./E.*1e-6;"("E"=6.0 ("Real"), "temp"=w512, "press"=w511, "p_raw_far"=w488, "b_far"=w469, "b_near"=w468, "p_raw_near"=w460, "accum_num"=w464, "t_d"="dead time") -> ("nrb_far"=w483:cdb[], "D_far"=w474:dbl[], "nrb_near"=w482:cdb[], "D_near"=w473:dbl[], "b_CR_far"=w466:dbl, "b_CR_near"=w465:dbl)  [unwired: 1 in, 1 out]
                    n387 = local read "bins"() -> (w492:u32)
                    n388 = local read "Altitude Array (km)"() -> (w485:dbl[])
                    n389 = Bundle(w466, w465) -> (→"?":cluster{dbl, dbl})  [unwired: 1 in]
                    n390 = Build Array(w483, w482) -> (w487:cdb[][])
                    n391 = Build Array(w474, w473) -> (w472:dbl[][])
                    n392 = Reshape Array(w482, w493, w492) -> (→"NRB 2":cdb[][])
                    n393 = Reshape Array(w483, w493, w492) -> (→"NRB":cdb[][])
                    n394 = Build Array(w485, w485) -> (w484:dbl[][])
                    n395 = call "Convert to Dynamic Data7"("2D Array"=w472) -> ("Dynamic Data Type"=w471:dynamicdata)  [unwired: 3 in]
                    n396 = call "Convert to Dynamic Data3"("2D Array"=w487) -> ("Dynamic Data Type"=w486:dynamicdata)  [unwired: 3 in]
                    n397 = call "Convert to Dynamic Data4"("2D Array"=w484) -> ("Dynamic Data Type"=w475:dynamicdata)  [unwired: 3 in]
                    n398 = call "Build XY Graph2"("Y Input"=w475, "X Input"=w486) -> ("XY Graph"=→"NRB plot":cluster{"Y":dbl[], "Y":dbl[]}[])  [unwired: 3 in, 6 out]
                    n399 = call "Build XY Graph4"("Y Input"=w475, "X Input"=w471) -> ("XY Graph"=→"Correction":cluster{"Y":dbl[], "Y":dbl[]}[])  [unwired: 3 in, 6 out]
                  }
                  frame #4 {
                    # "REPLACE WITH NEW AGILTRON TASK!"
                    # "Toggle Agiltron switch to online DBR"
                    n400 = disable-structure shown="Disabled" {
                      frame Disabled {
                        # "ABSORBING"
                        n401 = flat-sequence {
                          frame #0 {
                            # "Third one"
                            # "Command the switch to switch to position 1\ncorresponding to the online DBR"
                            # "Hex string command \ncorrespond to online"
                            n402 = local read "Switch Comm Port"() -> (w535:refnum<visa-resource-name>)
                            n403 = VISA Write(VISA resource name=w535, write buffer="\u0001\u0012\u0000\u0002") -> ()  [unwired: 1 in, 3 out]
                          }
                        }
                        n404 = Build Array(FALSE ("Boolean")) -> (w534:bool[])
                        n405 = call-poly <vilib>:"DAQmx Write.vi"("task/channels in"=refnum<k21> "AgiltronSwitch", "data"=w534) -> ()  [unwired: 11 in, 3 out]
                      }
                      frame Enabled {
                      }
                    }
                  }
                  frame #5 {
                    # "If 'Save Data?' is true, save all relavant offline info"
                    n406 = local read "Save Data?"() -> (w537:bool)
                    n407 = case shown="True" w537 {
                      frame False {
                        # "'Save Data?' is false, do nothing"
                      }
                      frame True {
                        # "Write only one data file at this time"
                        # "Retrive Julian Date"
                        # "'Save Data?' is true, save offline data to the Data Disk"
                        n408 = local read "Readings"() -> (w539:T6)
                        n409 = local read "Off-Line Bin Readings 2"() -> (w558:dbl[])
                        n410 = local read "Lambda Off Read (nm)"() -> (w560:dbl)
                        n411 = local read "Off-Line  Bin Readings"() -> (w565:dbl[])
                        n412 = local read "Relative Humdity (%)"() -> (w564:dbl)
                        n413 = local read "Offline Pulse Energy"() -> (w561:dbl)
                        n414 = local read "Temperature (C)"() -> (w562:dbl)
                        n415 = Unbundle By Name(w539) -> ("OffLineLD"=w538:dbl)
                        n416 = local read "Pressure (mb)"() -> (w563:dbl)
                        n417 = call "Julian_Date_2.vi"() -> ("Julian Date"=w559:dbl)  [unwired: 11 in]
                        n418 = Build Array (concatenate)(w559, w560, w538, w561, w562, w563, w564, w565) -> (w544:dbl[])
                        n419 = Build Array (concatenate)(w559, w560, w538, w561, w562, w563, w564, w558) -> (w541:dbl[])
                        n420 = local read "FF_Off_Ref"() -> (w546:refnum<file>)
                        n421 = local read "NF_Off_Ref"() -> (w543:refnum<file>)
                        n422 = local read "FF_Off_Ptr"() -> (w545:i64)
                        n423 = local read "NF_Off_Ptr"() -> (w542:i64)
                        n424 = Set File Position(offset (in bytes) (0)=w545, refnum=w546) -> (refnum out=w557:refnum<file>, error out=w555:errorcluster)  [unwired: 2 in]
                        n425 = Set File Position(offset (in bytes) (0)=w542, refnum=w543) -> (refnum out=w553:refnum<file>, error out=w551:errorcluster)  [unwired: 2 in]
                        n426 = Write to Binary File(file (use dialog)=w557, data=w544, error in=w555, 5:FALSE ("prepend array or string size? (T)")) -> (refnum out=w556:refnum<file>, error out=w554:errorcluster)  [unwired: 2 in, 1 out]
                        n427 = Write to Binary File(file (use dialog)=w553, data=w541, error in=w551, 5:FALSE ("prepend array or string size? (T)")) -> (refnum out=w552:refnum<file>, error out=w550:errorcluster)  [unwired: 2 in, 1 out]
                        n428 = Get File Position(4:w554, 7:w556) -> (2:w547:i64)  [unwired: 2 out]
                        n429 = Get File Position(4:w550, 7:w552) -> (2:w540:i64)  [unwired: 2 out]
                        n430 = local write "FF_Off_Ptr"(w547) -> ()
                        n431 = local write "NF_Off_Ptr"(w540) -> ()
                      }
                    }
                  }
                }
              }
              frame #4 {
                n432 = First Call?() -> (First Call?: T/F=w568:bool)
                n433 = Or(x="calculate absorption cross sections", y=w568) -> (x .or. y?=w566:bool)
                n434 = case shown="True" w566 {
                  frame False {
                  }
                  frame True {
                    # "calculate absorption cross sections from HITRAN data base"
                    n435 = local read "Off-Line Smoothed"() -> (w569:dbl[])
                    n436 = local read "Lambda On Read (nm)"() -> (w572:dbl)
                    n437 = local read "Lambda Off Set (nm)"() -> (w575:dbl)
                    n438 = local read "Temperature (C)"() -> (w573:dbl)
                    n439 = local read "Pressure (mb)"() -> (w574:dbl)
                    n440 = script code="hitran = dlmread('C:\\H2O_DIAL\\LabVIEW-2012\\Micropulse DIAL Matlab\\815nm_841nm_HITRAN_2008.csv', ',',[1 1 1676 8]);\n%hitran = dlmread('C:\\H2O_DIAL\\LabVIEW-2012\\Micropulse DIAL Matlab\\824nm_841nm_H2O_Spectral_Calc.csv', ',',[1 1 1209 7]);\n\n\n\n%Range vector in meters\nrange = ([75:75:size(Online,2)*75]);\n\nif lambda< 828\nlambda=828.195;\nelse\nlambda=lambda;\nend;\n\n%%\n\n%Voigt profile calculation\nWNmin = 1/(828+4)*1e7;  % 832.0 nm converted to wavenumber\nWNmax = 1/(828-4)*1e7;  % 824.0 nm converted to wavenumber\n\n%Find lines from WNmin to WNmax to calculate voigt profile\nline_indices = hitran(1:size(hitran,1),1)>WNmin & hitran(1:size(hitran,1),1)<WNmax;\n\nline = double(hitran(line_indices, 1:size(hitran,2)));\n\n%Calculate temperature and pressure profile\nT0 = 273+25; % surface temperature\nT0 = 273+T0_C;\nT = T0-0.0065.*range; % set to match the sounding\n\n% pressure in atmospheres\nP0  = 0.83; % surface pressure\nP0  = P0_mb/1000*0.986; %pressure in mb converted to atm\nP = P0.*(T0./T).^-5.5;   % set this value to match sounding\n\nT00 = 296;              % HITRAN reference temperature [K]\nP00 = 1;                % HITRAN reference pressure [atm]\nnu0_0 = line(:,1);      % absorption line center wavenumber from HITRAN [cm^-1]\nS0 = line(:,2);         % initial linestrength from HITRAN [cm^-1/(mol*cm^-2)]   \ngammal0 = line(:,4);    % air-broadened halfwidth at T_ref and P_ref from HITRAN [cm^-1/atm]\ngamma_s = line(:,5);    % self-broadened halfwidth at T_ref and P_ref from HITRAN [cm^-1/atm]\nE = line(:,6);          % ground state transition energy from HITRAN [cm^-1]  \nalpha = line(:,7);      % linewidth temperature dependence factor from HITRAN\ndelta = line(:,8);      % pressure shift from HiTRAN [cm^-1 atm^-1]\n\nnu_on = 1/(lambda)*1e7;\nnu_off = 1/(lambda_off)*1e7;\n\nfor i = 1:size(Online,2); % calculate the absorption cross section at each range\n  \n    nu0 = nu0_0+delta.*(P(i)./P00); % unclear if it should be Pi/P00  \n    gammal = gammal0.*(P(i)./P00).*((T00./T(i)).^alpha);    %Calculate Lorentz lineweidth at P(i) and T(i)\n\n    const.m = 18.015E-3./6.022E23; % mass of a single water molecule\n    const.k_B = 1.3806488e-23; % (J/K)\n    const.c = 299792458; % (m/s) (exact)\n \n    gammad = (nu0).*((2.0.*const.k_B.*T(i).*log(2.0))./(const.m.*const.c^2)).^(0.5);  %Calculate HWHM Doppler linewidth at T(i)\n     \n    % term 1 in the Voigt profile\n    y = (gammal./gammad).*((log(2.0)).^(0.5));\n    \n    % term 2 in the Voigt profile\n    x_on = ((nu_on-nu0)./gammad).*(log(2.0)).^(0.5);\n    x_off = ((nu_off-nu0)./gammad).*(log(2.0)).^(0.5);\n    \n    %setting up Voigt convolution\n    t = (-(size(line,1))/2:1:size(line,1)/2-1); %set up the integration spectral step size\n    t = repmat(t',1,length(x_on))';\n    x_on = repmat(x_on,1,length(t));\n    x_off = repmat(x_off,1,length(t));\n    y = repmat(y,1,length(t));\n    f_on = (exp(-t.^2.0))./(y.^2.0+(x_on-t).^2.0);  % combined Voigt term 1 and 2\n    f_off = (exp(-t.^2.0))./(y.^2.0+(x_off-t).^2.0);\n    %Voigt integration over all of the lines at the on and offline locations\n    z_on = trapz(t(1,:),f_on,2);\n    z_off =  trapz(t(1,:),f_off,2);\n    integral_on = z_on;\n    integral_off = z_off;\n    %Calculate linestrength at temperature T\n    S = S0.*((T00./T(i)).^(1.5)).*exp(1.439.*E.*((1./T00)-(1./T(i))));\n \n    %Calculate the Voigt profile\n    K_on = (y(:,1)./pi).*integral_on;\n    K_off = (y(:,1)./pi).*integral_off;\n    \n    %Calculate the Voigt profile absorption cross section [cm^2]\n    sigmav_on = S.*(1./gammad).*(((log(2.0))./pi).^(0.5)).*K_on; %.*far_wing_on;\n    sigmav_off = S.*(1./gammad).*(((log(2.0))./pi).^(0.5)).*K_off; %.*far_wing_off;\n    \n    %Sum contributions from all of the surrounding lines\n    sigma_on_total(i) = sum(sigmav_on);\n    sigma_off_total(i) = sum(sigmav_off);\n    \nend;"("lambda"=w572, "lambda_off"=w575, "P0_mb"=w574, "T0_C"=w573, "Online"=w569) -> ("sigma_on_total"=→"sigma_on_total":dbl[], "sigma_off_total"=→"sigma_off_total":dbl[])  [unwired: 1 in, 1 out]
                  }
                }
              }
              frame #5 {
                w586 = 1
                # "normalization factor\nfrom 300 to 450m"
                # "OPTICAL DEPTH PLOT"
                # "new rainbow color bar display"
                # "Data Processing Far Channel"
                # "new rainbow color bar display"
                # "Calculating the range resolved water vapor number density and plotting"
                n441 = local read "sigma_off_total"() -> (w609:dbl[])
                n442 = local read "sigma_on_total"() -> (w606:dbl[])
                n443 = local read "On-Line  Smoothed"() -> (w584:dbl[])
                n444 = local read "Off-Line Smoothed"() -> (w583:dbl[])
                n445 = local read "Off-Line Smoothed 2"() -> (w607:dbl[])
                n446 = local read "On-Line Smoothed 2"() -> (w608:dbl[])
                n447 = script code="%Time averaging in seconds.  180 Seconds =3 minutes\ntemporal_average = 180;\n\n%Spatial averaging in bins.  2 bins = 150 meters\nspatial_average = 2;\n\n%Creating r and r+deltar vectors..this can also be acsomplished using the\n%diff command\np_oni = Online(:,1:size(Online,2)-1);\n\np_onii = Online(:,2:size(Online,2));\n\np_offi = Offline(:,1:size(Offline,2)-1);\n\np_offii = Offline(:,2:size(Offline,2));\n\nInside = (p_oni.*p_offii)./(p_onii.*p_offi);\n\ndel_cross = 1./(2.*(sigma_on_total(1:size(Online,2)-1)-sigma_off_total(1:size(Offline,2)-1)).*75*100);\n\ndel_cross(isinf(del_cross)) = 0;\n\n%Calculating Number density\nN = del_cross.*log(Inside);\n\n%Spatial smoothing of the profiles\nfilter1 = ones(1,2)./2;\n\nN_1 = N;\n\nN_1_avg = filter2(filter1,N_1);\n\nfilter1 = ones(1,10)./10;\n\nN_2 = N;\n\nN_2_avg = filter2(filter1,N_2);\n\nN_new = zeros(size(N,1),size(N,2));\n \n%Using different averaging windows for different altitudes \nN_avg=[N_1_avg(:,1:40)';N_2_avg(:,41:size(N,2))']';\n\n\nw = N_avg.*1e6.*18.015./6.022e23"("Online"=w608, "Offline"=w607, "sigma_on_total"=w606, "sigma_off_total"=w609) -> ("N_avg"=w610:cdb[], "w"=w619:cdb[])  [unwired: 1 in, 1 out]
                n448 = script code="%Time averaging in seconds.  180 Seconds = 3 minutes\ntemporal_average = 180;\n\n%Spatial averaging in bins.  2 bins = 150 meters\nspatial_average = 2;\n\n%Creating r and r+deltar vectors..this can also be acsomplished using the\n%diff command\np_oni = Online(:,1:size(Online,2)-1);\n\np_onii = Online(:,2:size(Online,2));\n\np_offi = Offline(:,1:size(Offline,2)-1);\n\np_offii = Offline(:,2:size(Offline,2));\n\nInside = (p_oni.*p_offii)./(p_onii.*p_offi);\n\ndel_cross = 1./(2.*(sigma_on_total(1:size(Online,2)-1)-sigma_off_total(1:size(Offline,2)-1)).*75*100);\n\ndel_cross(isinf(del_cross)) = 0;\n\n%Calculating Number density\nN = del_cross.*log(Inside);\n\n%Spatial smoothing of the profiles\nfilter1 = ones(1,2)./2;\n\nN_1 = N;\n\nN_1_avg = filter2(filter1,N_1);\n\nfilter1 = ones(1,10)./10;\n\nN_2 = N;\n\nN_2_avg = filter2(filter1,N_2);\n\nN_new = zeros(size(N,1),size(N,2));\n \n%Using different averaging windows for different altitudes \nN_avg=[N_1_avg(:,1:40)';N_2_avg(:,41:size(N,2))']';\n\n \nw = N_avg.*1e6.*18.015./6.022e23"("Online"=w584, "Offline"=w583, "sigma_on_total"=w606, "sigma_off_total"=w609) -> ("N_avg"=w615:cdb[], "w"=w616:cdb[])  [unwired: 1 in, 1 out]
                n449 = local read "Time Resolution Per Bin(ns)"() -> (w585:u32)
                n450 = local read "bins"() -> (w611:u32)
                n451 = local read "Altitude Array (km)"() -> (w581:dbl[])
                n452 = Build Array(w616, w619) -> (w622:cdb[][])
                n453 = To Double Precision Float(number=w585) -> (double precision float=w604:dbl)
                n454 = Reshape Array(w615, w586, w611) -> (w626:cdb[][])
                n455 = Reshape Array(w610, w586, w611) -> (w613:cdb[][])
                n456 = Multiply(x=0.15, y=w604) -> (x*y=w602:dbl)
                n457 = Build Array(w615, w610) -> (w620:cdb[][])
                n458 = Divide(x=300.0, y=w602) -> (x/y=w599:dbl)
                n459 = Divide(x=450.0, y=w602) -> (x/y=w598:dbl)
                n460 = Build Array(w581, w581) -> (w605:dbl[][])
                n461 = call "Convert to Dynamic Data5"("2D Array"=w622) -> ("Dynamic Data Type"=w621:dynamicdata)  [unwired: 3 in]
                n462 = call "Convert to Dynamic Data2"("2D Array"=w620) -> ("Dynamic Data Type"=w617:dynamicdata)  [unwired: 3 in]
                n463 = Divide(x=w626, y=1e+17) -> (x/y=→"Water Vapor Number Density":cdb[][])
                n464 = Divide(x=w613, y=1e+17) -> (x/y=→"Water Vapor Number Density 2":cdb[][])
                n465 = call "Convert to Dynamic Data6"("Array"=w581) -> ("Dynamic Data Type"=w582:dynamicdata)  [unwired: 3 in]
                n466 = To Long Integer(number=w599) -> (32bit integer=w597:i32)
                n467 = To Long Integer(number=w598) -> (32bit integer=w596:i32)
                n468 = call "Convert to Dynamic Data"("2D Array"=w605) -> ("Dynamic Data Type"=w618:dynamicdata)  [unwired: 3 in]
                n469 = call "Convert to Dynamic Data8"("2D Array"=w605) -> ("Dynamic Data Type"=w623:dynamicdata)  [unwired: 3 in]
                n470 = Decrement(x=w597) -> (x-1=w594:i32)
                n471 = Decrement(x=w596) -> (x-1=w595:i32)
                n472 = call "Build XY Graph"("Y Input"=w618, "X Input"=w617) -> ("XY Graph"=→"Water Vapor Number Density  2":cluster{"Y":dbl[], "Y":dbl[]}[])  [unwired: 3 in, 6 out]
                n473 = call "Build XY Graph3"("Y Input"=w623, "X Input"=w621) -> ("XY Graph"=→"Absolute Humidity":cluster{"Y":dbl[], "Y":dbl[]}[])  [unwired: 3 in, 6 out]
                n474 = Array Subset(array=w584, index=w594, length=w595) -> (w593:dbl[])
                n475 = Array Subset(array=w583, index=w594, length=w595) -> (w592:dbl[])
                n476 = call-poly <vilib>:"Mean.vi"("X"=w593) -> ("mean"=w591:dbl)  [unwired: 1 out]
                n477 = call-poly <vilib>:"Mean.vi"("X"=w592) -> ("mean"=w590:dbl)  [unwired: 1 out]
                n478 = Divide(x=w591, y=w590) -> (x/y=w589:dbl)
                n479 = Multiply(x=w583, y=w589) -> (x*y=w588:dbl[])
                n480 = Divide(x=w584, y=w588) -> (x/y=w587:dbl[])
                n481 = Natural Logarithm(1:w587) -> (0:w578:dbl[])
                n482 = Multiply(x=-1.0, y=w578) -> (x*y=w577:dbl[])
                n483 = call "Convert to Dynamic Data9"("Array"=w577) -> ("Dynamic Data Type"=w580:dynamicdata)  [unwired: 3 in]
                n484 = call "Build OD Plot"("Y Input"=w582, "X Input"=w580) -> ("XY Graph"=→"Optical Depth":cluster{"Y":dbl[], "Y":dbl[]}[])  [unwired: 3 in, 6 out]
              }
            }
          }
        }
        "L_Count" <- w129
      }
    }
  }
  n485 = case shown="True" w3 {
    frame False {
    }
    frame True {
      # "close data files"
      # "Close Bristol WM"
      n486 = local read "Bristol Out"() -> (w633:i32)
      n487 = local read "NF_Off_Ref"() -> (w629:refnum<file>)
      n488 = local read "NF_On_Ref"() -> (w630:refnum<file>)
      n489 = local read "FF_Off_Ref"() -> (w631:refnum<file>)
      n490 = local read "FF_On_Ref"() -> (w632:refnum<file>)
      n491 = dll-call lib="C:/H2O_DIAL/LabVIEW-2012/Bristol WM V2_31b/CLDevIFace.dll" fn="CLCloseDevice"("CommPort"=w633) -> ()  [unwired: 5 in, 2 out]
      n492 = Close File(refnum=w632) -> ()  [unwired: 1 in, 2 out]
      n493 = Close File(refnum=w631) -> ()  [unwired: 1 in, 2 out]
      n494 = Close File(refnum=w630) -> ()  [unwired: 1 in, 2 out]
      n495 = Close File(refnum=w629) -> ()  [unwired: 1 in, 2 out]
    }
  }
  "FileHour" <- -1 ("FileHour")
  "DataOpen" <- FALSE
